vi "SpectrometerSpinCoater_v13.vi"() -> ()   [LabVIEW 2020]
uses:
  TypDef/TabControl_InSitu_Type.ctl
  <instrlib>/Classes/CCD/Abstract_CCD/Abstract_CCD.lvclass
  <instrlib>/Classes/SpinCoater/SpinCoater.lvclass
  TypDef/DeviceQueue_TypeDef.ctl
  TypDef/DeviceQueue_Action.ctl
  TypDef/TabControl.ctl
  TypDef/DataQueue_TypeDef.ctl
  TypDef/DataQueue_Action.ctl
  <vilib>/Utility/error.llb/DialogType.ctl
  <instrlib>/Classes/CCD/Avantes/Avantes.lvclass
  C:/Program Files/National Instruments/LabVIEW 2020/instr.lib/Classes/CCD/Abstract_CCD/Abstract_CCD.lvclass
  <vilib>/Analysis/baseanly.llb/A x Vector.vi
  <vilib>/Analysis/NI_AALBase.lvlib
panel:
  out "x-y":dbl
  in  "Reference\nValue":dbl=1.0
  out "WL-Det\nPos":i32
  in  "Motor_ShortStop":bool
  out "UpperWLLimit":i32=1065
  out "LowerWLLimit":i32=149
  out "Nr After Spin":u16
  out "Action":string="TimeOut"
  out "Time.spin":refnum<file>
  out "Meas.spin":refnum<file>
  out "Arduino":bool
  out "NKT":bool
  out "Spectromter":bool
  in  "Abort Button":bool
  in  "Stop Button":bool=TRUE
  in  "Tab Control":T1(tab)=enum."Settings"
  in  "Trim\nSpec":bool=TRUE
  in  "Wl \nUp":dbl[unit]=9.102385253906251e-07
  in  "Wl \nLow":dbl[unit]=3.7998095703125003e-07
  in  "Frames for Ref/Dark":dbl=10000.0
  in  "Shutter Toggle":bool
  in  "Program Spin Coater":T2(array[cluster])=[{"Speed (rpm)"=1430.0, "Time (s)"=45.0, "Acc (rpm/s)"=0.0}]
  in  "Spectra Count":u16
  in  "Measure_MeasureSpectrum":bool
  out "Overall Time":dbl=47.0
  in  "Frames":i32=123685
  in  "StartMeasurement_Button":bool
  in  "Measure_Preview":bool
  out "Measure_Graph":T3(graph) caption="XY Graph"
  in  "Measure_FramesSpectrometer":dbl=200.0 caption="Frames for Spectrometer"
  in  "StartSpin_Button":bool
  in  "Record RefSpec":bool
  in  "Measure:\nRecord_Darkspec":bool
  in  "Measure_Comments":string="Just for testing" caption="Comments"
  in  "Measure_FileName":string="Testing" caption="File Name"
  in  "Measure_SavePath":path=path "C:/Users/Cerberus/Desktop/Test/v12Test" caption="Save Path"
  out "Measure_FrameRate":dbl[unit]=2631.5791015625 caption="Frame Rate"
  in  "Measure_IntegrationTime":dbl[unit]=3e-05 caption="Integration Time"
  in  "Tab Control SpinType":T4
  in  "Seconds after Spin":dbl[unit]=1.0
  in  "Calculate Frames_Normal":bool=TRUE caption="Calculate Frames"
  in  "periodic time":dbl[unit]=2.0
  in  "Duration after":dbl[unit]
  in  "Spin at end":bool
  in  "Seconds to Spin_Normal":dbl[unit]=1.0 caption="Seconds to Spin"
  in  "Threshold":dbl=0.3
  in  "Time Detect":dbl[unit]=2.0
  in  "Seconds to Spin_Short":dbl[unit]=1.0 caption="Seconds to Spin"
  in  "Spin Time":dbl[unit]=2.0
  in  "Calculate Frames_Short":bool=TRUE caption="Calculate Frames"
  in  "Wavelenght Detect":dbl[unit]=6.000000000000001e-07
  out "SS_StepsLeft":dbl
  out "SS_TimePrediction":dbl[unit]=-6.0
  out "Horizontal Progress Bar":u8(slide) scale=0.0..100.0
  in  "SpectralStability:\nRecord_Darkspec":bool
  in  "SpectralStability_Record":bool
  in  "SpectralStability_\nMeasurementNumber":u32 caption="Measurement Number"
  in  "SpectralStability_Duration":dbl[unit] caption="Duration"
  in  "Duration/Times":bool
  in  "SpectralStability_\nPeriodicTime":dbl[unit] caption="Periodic Time"
  in  "SpectralStability_MeasureSpectrum":bool
  in  "SpectralStability_Preview":bool
  out "SpectralStability_Graph":T3(graph) caption="XY Graph"
  in  "SpectralStability_FramesSpectrometer":dbl=200.0 caption="Frames for Spectrometer"
  in  "SpectralStability_Comments":string="Just for testing" caption="Comments"
  in  "SpectralStability_FileName":string="TestingAfter" caption="File Name"
  in  "SpectralStability_SavePath":path=path "C:/Users/Timo/Desktop/Test/180824" caption="Save Path"
  out "SpectralStability_FrameRate":dbl[unit]=2631.5791015625 caption="Frame Rate"
  in  "SpectralStability_IntegrationTime":dbl[unit]=3e-05 caption="Integration Time"
  in  "Shutter Close":bool
  in  "Shutter Open":bool
  in  "SHUTTER DEBUG":bool
  in  "Shutter Position":u16=1000
  in  "Dividider Get Spectra":u32=1 min=1
  in  "Automatically \nadjust count":bool=TRUE
  in  "Reset Count\nafter Spin Coating":bool=TRUE
  in  "ESC_Speed":dbl
  in  "ESC_Milliseconds":dbl
  in  "ESC DEBUG":bool
  in  "Port Arduino":refnum<visa-resource-name>="COM7"
  out "Error Arduino":bool caption="Error"
  in  "Init_Arduino":bool caption="Init"
  out "Caption_Settings_Arduino":string="Arduino"
  out "Caption_Settings_NKT":string="NKT Laser"
  out "Error_Spectromter":bool caption="Error"
  in  "Init_Spectrometer":bool caption="Init"
  out "Caption_Settings_Spectrometer":string="Spectromter"
  # "Speed (rpm)   Time (s)        Acceleration \n                                               (rpm/s)"
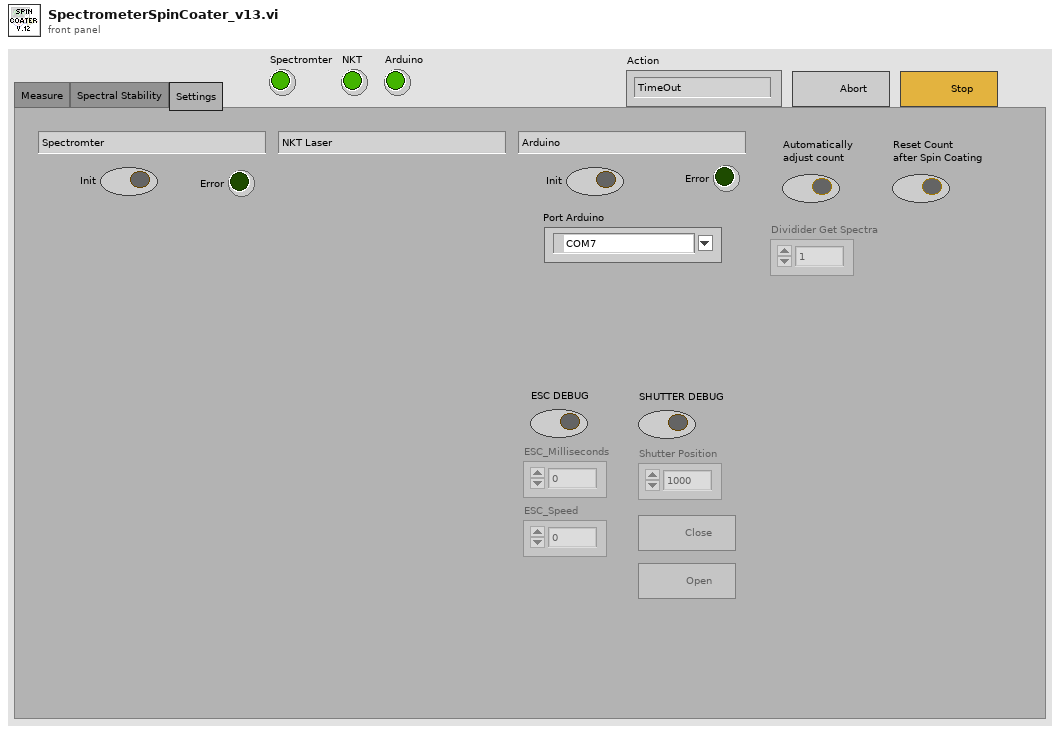
[diagram p1: front panel]
types:
  T1 = enum32{"Measure", "Spectral Stability", "Settings"}
  T2 = cluster{"Speed (rpm)":dbl, "Time (s)":dbl, "Acc (rpm/s)":dbl}[]
  T3 = cluster{"Wavlength":dbl[unit][], "Image":dbl[]}[]
  T4 = typedef "TabControl_InSitu_Type.ctl" = enum32{"Normal", "Short"}
  T5 = cluster{"Dark":cluster{"Image":dbl[][][], "Frame Size":cluster{"F":i32, "Y":i32, "X":i32}}[], "Ref":cluster{"Image":dbl[][][], "Frame Size":cluster{"F":i32, "Y":i32, "X":i32}}[], "Wavlength":dbl[unit][], "Wavlength Trim":dbl[unit][], "spec":dbl[][]}
  T6 = cluster{"Abstract_CCD.lvclass":refnum<class "Abstract_CCD.lvclass">, "SpinCoater.lvclass":refnum<class "SpinCoater.lvclass">}
  T7 = enum8{"Enabled", "Disabled", "Disabled and Grayed Out"}
  T8 = typedef "DataQueue_TypeDef.ctl" = cluster{"QueueAction":T9, "Data":cluster{"Image":dbl[][][], "Frame Size":cluster{"F":i32, "Y":i32, "X":i32}}[], "Data_Raw":cluster{"Image":dbl[][][], "Frame Size":cluster{"F":i32, "Y":i32, "X":i32}}[], "Data_Dark":cluster{"Image":dbl[][][], "Frame Size":cluster{"F":i32, "Y":i32, "X":i32}}[], "Data_Ref":cluster{"Image":dbl[][][], "Frame Size":cluster{"F":i32, "Y":i32, "X":i32}}[], "Device Information":string[], "Numeric Control":dbl, "Boolean":bool, "Wavelength":dbl[unit][], "Time":dbl[], "Time Stamp":timestamp, "Numeric Control 2":dbl, "TabControl":T10, "Numeric Control 3":dbl}
  T9 = typedef "DataQueue_Action.ctl" = enum16{"TimeOut", "Close_Program", "Abort", "Stop_Measurement", "Measure_InSituSpinCoating", "Measure_InSituSpinCoating_Short", "Measure_Spectrum", "Measure_SpectrumAdvanced", "Measure_SpectralStability", "Save_InSitu", "Save_SpectralStability", "Set_Ref", "Set_Dark", "Set_Wavelength", "Spectrometer_Measure", "Spectrometer_Preview", "Transfer_Settings", "Change_TrimSettings"}
  T10 = typedef "TabControl.ctl" = enum16{"Measure", "Spectral Stability", "Settings"}
  T11 = typedef "DeviceQueue_TypeDef.ctl" = cluster{"QueueAction":T12, "Numeric 1":dbl, "Numeric 2":dbl, "Boolean 1":bool, "Boolean 2":bool, "Spin Program":dbl[][], "Spin Prg v07":cluster{"Speed (rpm)":dbl, "Time (s)":dbl, "Acc (rpm/s)":dbl}[], "Time Stamp":timestamp, "TabControl":T10}
  T12 = typedef "DeviceQueue_Action.ctl" = enum16{"TimeOut", "Wait", "Close_Program", "Abort", "Spectrometer_Init", "Spectrometer_Close", "Spectrometer_DeviceInformation", "Spectrometer_Measure", "Spectrometer_MeasureAdvanced", "Spectrometer_Preview", "Spectrometer_Abort", "Spectrometer_StartMeasurement", "Spectrometer_GetData", "Spectrometer_GetData_Short", "Spectrometer_StopMeasurement", "Spectrometer_SetIntegrationTime", "Spectrometer_SetFrames", "Spectrometer_SetDarkspec", "Spectrometer_SetReference", "Spectrometer_SetTriggerMode", "Laser_Init", "Laser_Close", "Arduino_Init", "Arduino_Close", "Arduino_LoadProgram", "Arduino_StartProgram", "Arduino_SetSpeed", "Arduino_SetMillis", "Arduino_StopSpin", "Arduino_ShortStop", "Arduino_Shutter_SetPosition", "Arduino_Shutter_Close", "Arduino_Shutter_Open", "Measure_InSitu", "Measure_Spectrum", "Measure_InSituAdvanced", "Measure_InSituAdvanced_Short", "Measure_SpectralStability", "Measure_Stop"}
  T13 = enum16{"open", "replace", "create", "open or create", "replace or create", "replace or create with confirmation"}
  T14 = cluster{"Image":dbl[][][], "Frame Size":cluster{"F":i32, "Y":i32, "X":i32}}[]
  T15 = cluster{"Image":dbl[][][], "Frame Size":cluster{"F":i32, "Y":i32, "X":i32}}
  T16 = cluster{"Wavlength":dbl[unit][], "A x Vector":dbl[]}
  T17 = cluster{"Wavlength":dbl[unit][], "A x Vector":dbl[]}[]
  T18 = cluster{u16[][][], u16[][][], dbl[], "Numeric Control":dbl, "Numeric Control 2":dbl}
  T19 = typedef "DialogType.ctl" = u16
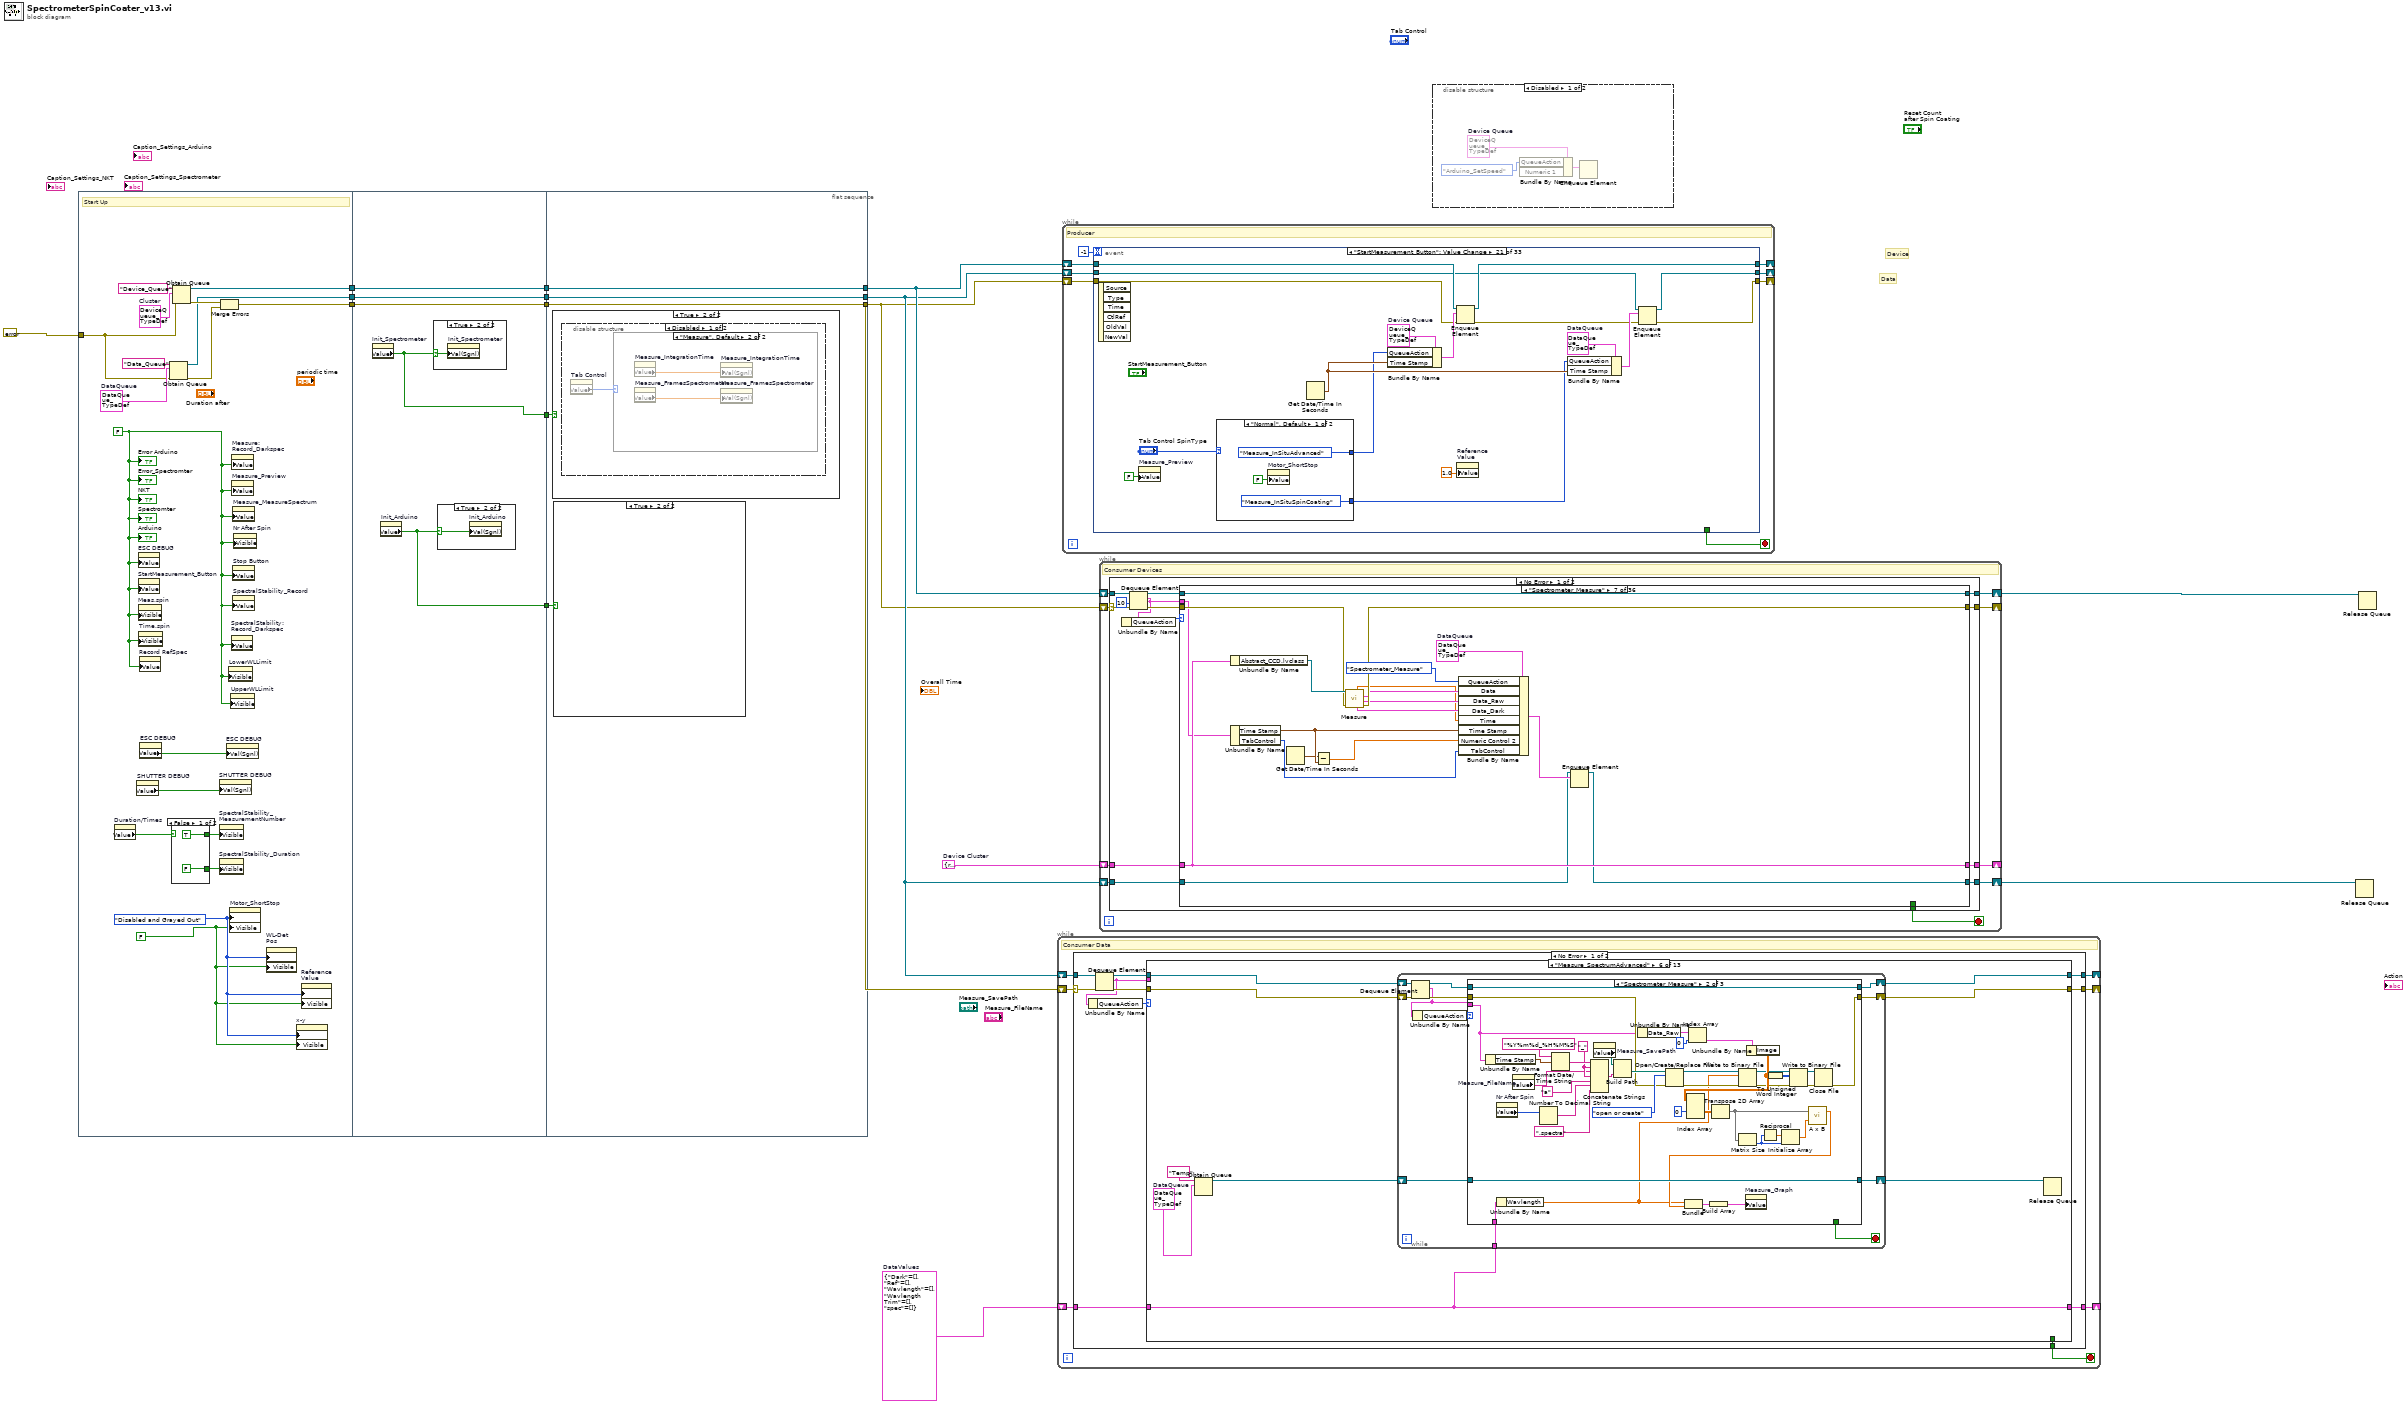
[diagram p0: block diagram]
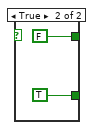
[diagram p3: hidden frame]
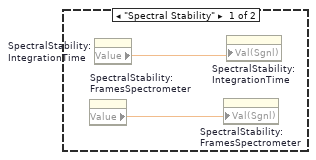
[diagram p8: hidden frame]
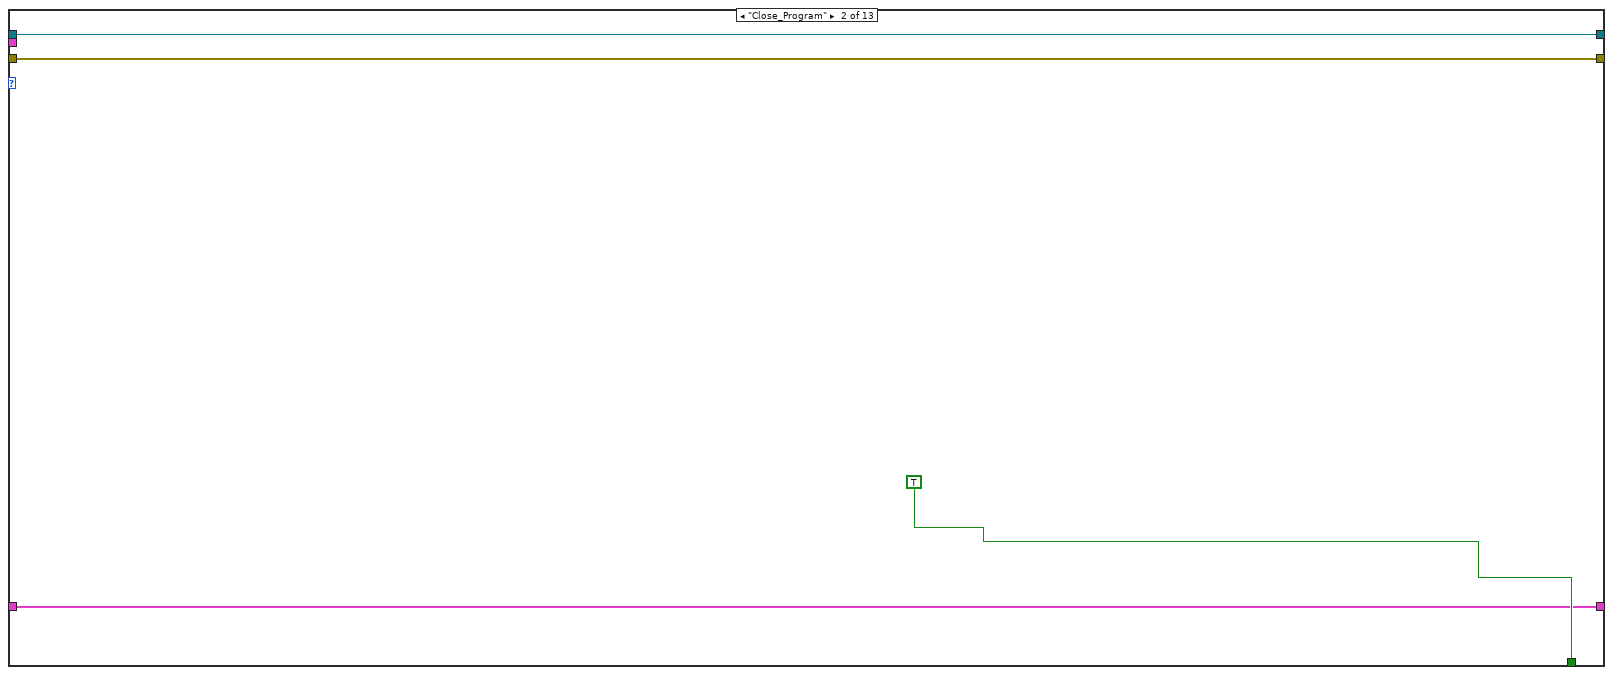
[diagram p11: hidden frame]
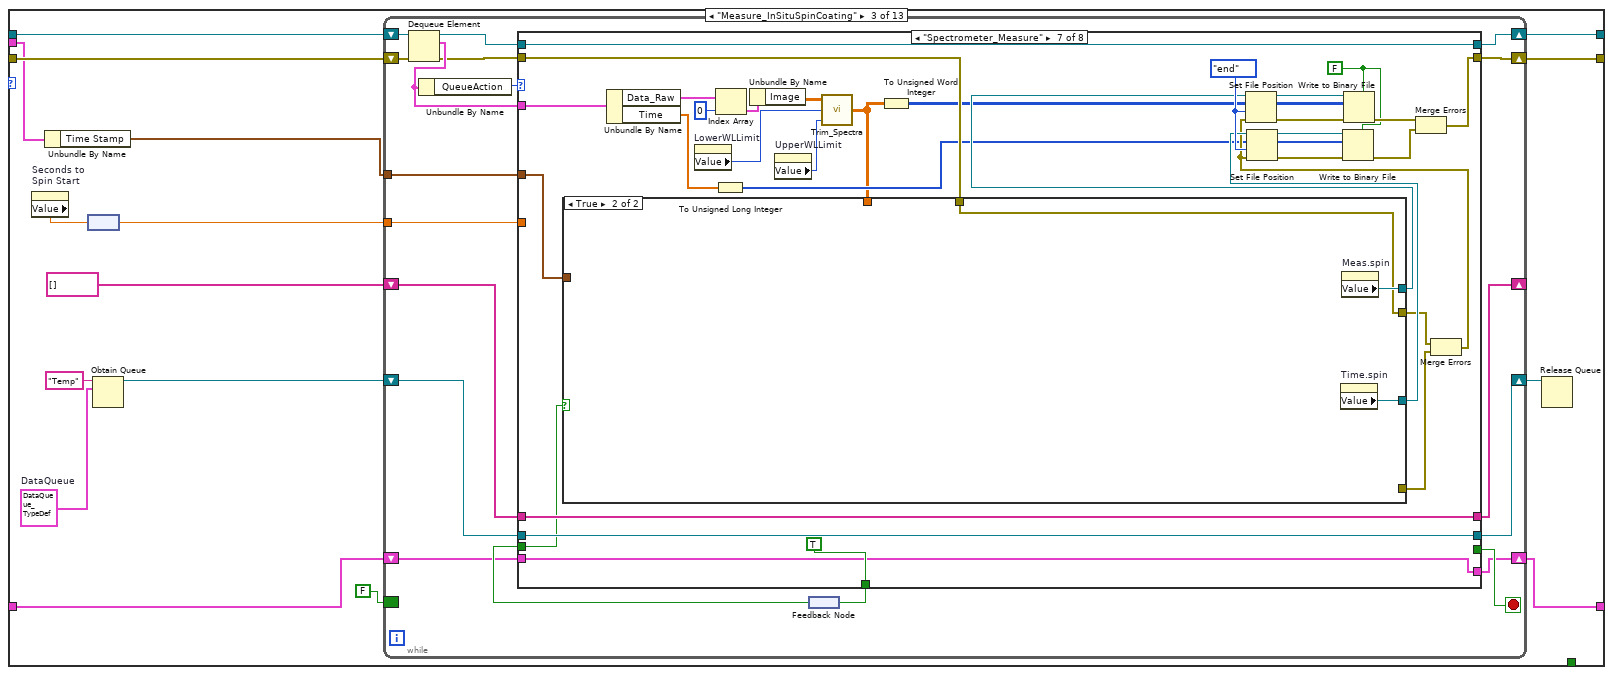
[diagram p12: hidden frame]
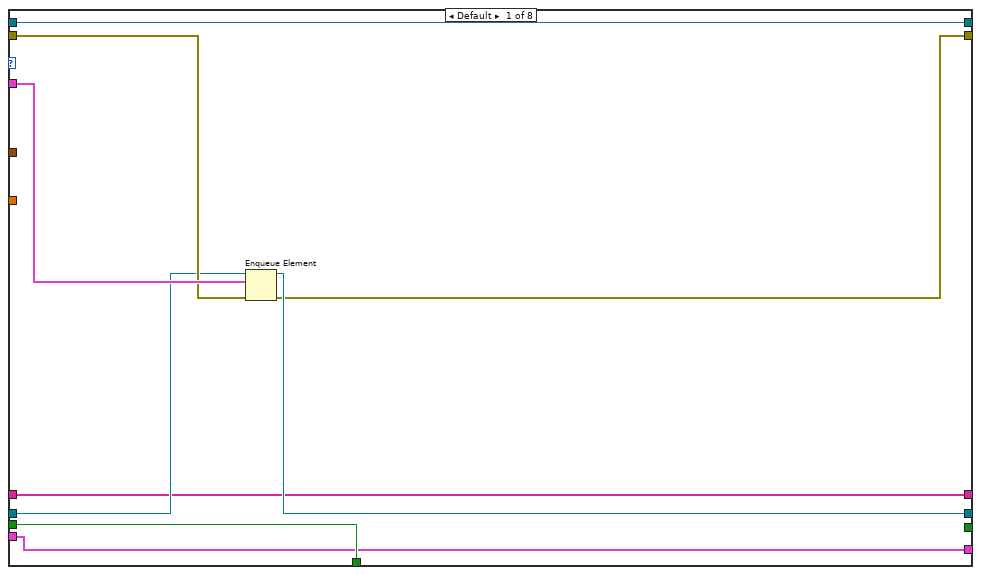
[diagram p13: hidden frame]
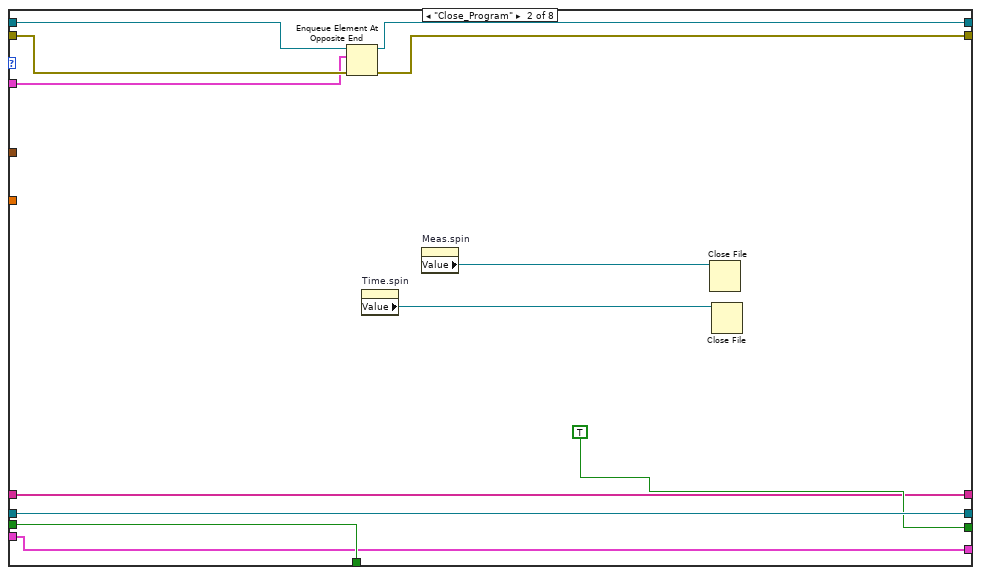
[diagram p14: hidden frame]
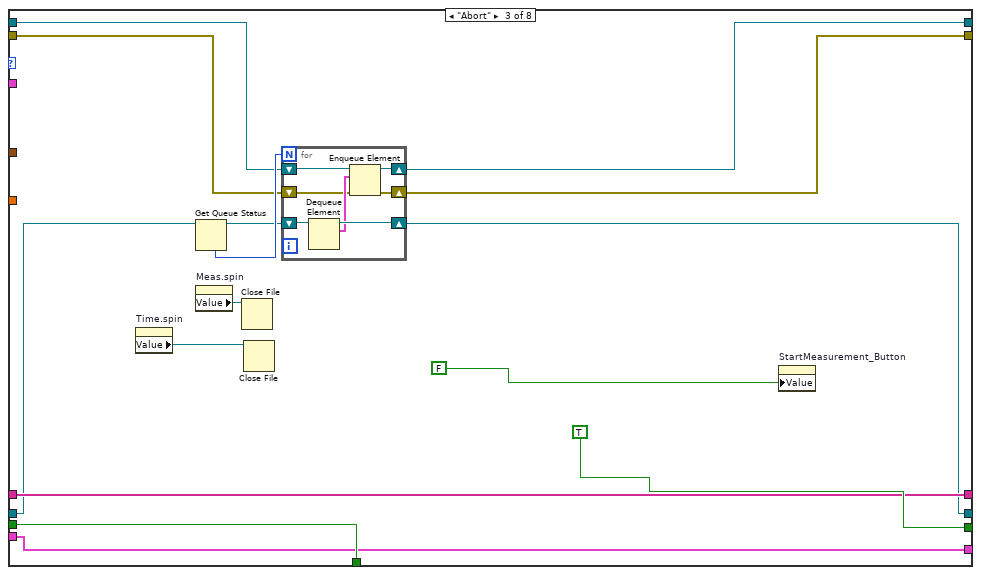
[diagram p15: hidden frame]
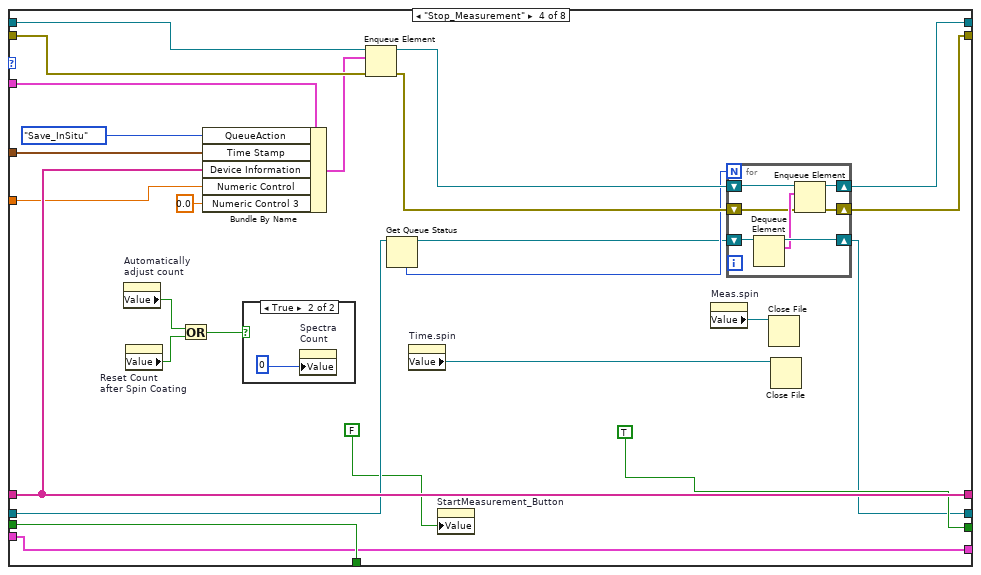
[diagram p16: hidden frame]
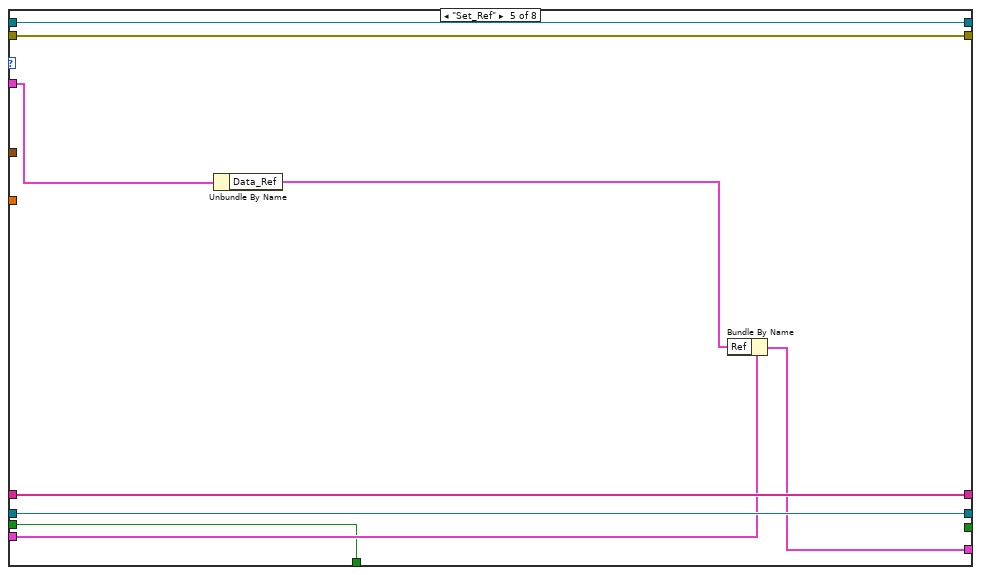
[diagram p18: hidden frame]
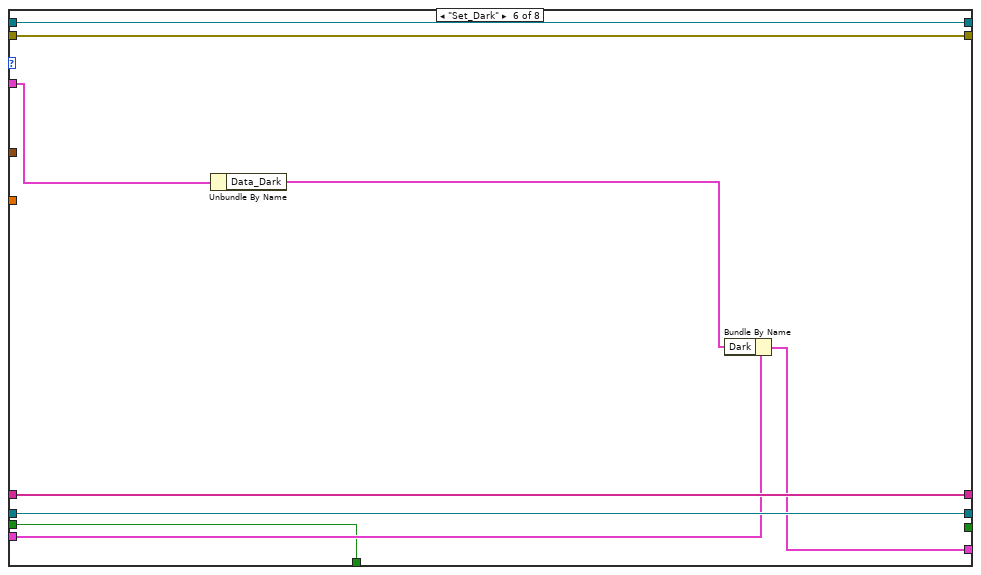
[diagram p19: hidden frame]
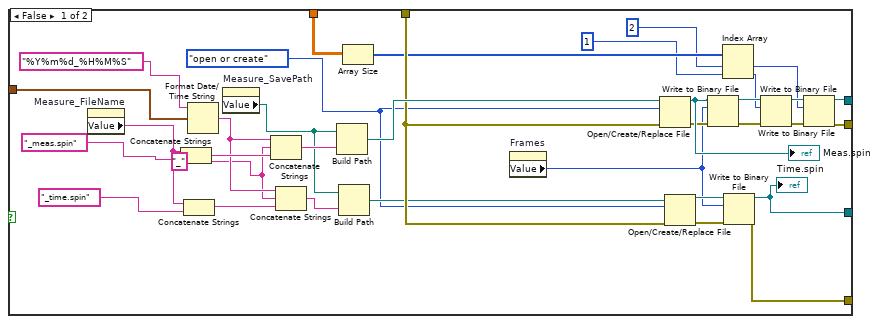
[diagram p20: hidden frame]
diagram:
  w7 = T5 {"Dark"=[], "Ref"=[], "Wavlength"=[], "Wavlength Trim"=[], "spec"=[]}  # DataValues
  w11 = T6 {"Abstract_CCD.lvclass"=refnum, "SpinCoater.lvclass"=refnum}  # Device Cluster
  # "Data"
  # "Device"
  n1 = flat-sequence {
    tunnel: errorcluster {"status"=FALSE, "code"=0, "source"=""} ("error constant") -> [w29]
    tunnel: [w32] -> w15
    tunnel: [w26] -> w14
    tunnel: [w25] -> w13
    tunnel: w15 -> [w43]
    tunnel: w14 -> [w42]
    tunnel: w13 -> [w41]
    tunnel: [w43] -> w6
    tunnel: [w42] -> w5
    tunnel: [w41] -> w4
    tunnel: [w40] -> w3
    tunnel: [w39] -> w2
    tunnel: [w48] -> w1
    tunnel: [w49] -> w8
    tunnel: [w50] -> w12
    tunnel: w6 -> [w50]
    tunnel: w5 -> [w49]
    tunnel: w4 -> [w48]
    tunnel: w3 -> [w47]
    tunnel: w2 -> [w46]
    frame #0 {
      w18 = T7."Disabled and Grayed Out" ("Disabled")
      w17 = FALSE ("Visible")
      w30 = T8 {"QueueAction"=enum."TimeOut", "Data"=[], "Data_Raw"=[], "Data_Dark"=[], "Data_Ref"=[], "Device Information"=[], "Numeric Control"=0.0, "Boolean"=FALSE, "Wavelength"=[], "Time"=[], "Time Stamp"=timestamp(0 s since 1904-01-01), "Numeric Control 2"=0.0, "TabControl"=enum."Measure", "Numeric Control 3"=0.0}  # DataQueue
      w33 = T11 {"QueueAction"=enum."TimeOut", "Numeric 1"=0.0, "Numeric 2"=0.0, "Boolean 1"=FALSE, "Boolean 2"=FALSE, "Spin Program"=[], "Spin Prg v07"=[], "Time Stamp"=timestamp(0 s since 1904-01-01), "TabControl"=enum."Measure"}  # Cluster
      w19 = FALSE ("Error Arduino")
      # "Start Up"
      n2 = property on="Duration/Times" class="Bool (strict)"() -> ("Value"=w21:bool)  [unwired: 2 in, 2 out]
      n3 = property on="SHUTTER DEBUG" class="Bool (strict)"() -> ("Value"=w20:bool)  [unwired: 2 in, 2 out]
      n4 = property on="ESC DEBUG" class="Bool (strict)"("Value"=w19) -> ()  [unwired: 2 in, 2 out]
      n5 = property on="StartMeasurement_Button" class="Bool (strict)"("Value"=w19) -> ()  [unwired: 2 in, 2 out]
      n6 = property on="Meas.spin" class="Ref (strict)"("Visible"=w19) -> ()  [unwired: 2 in, 2 out]
      n7 = property on="Time.spin" class="Ref (strict)"("Visible"=w19) -> ()  [unwired: 2 in, 2 out]
      n8 = property on="Record RefSpec" class="Bool (strict)"("Value"=w19) -> ()  [unwired: 2 in, 2 out]
      n9 = property on="ESC DEBUG" class="Bool (strict)"() -> ("Value"=w24:bool)  [unwired: 2 in, 2 out]
      n10 = Obtain Queue(name (unnamed)="Data_Queue", element data type=w30, error in (no error)=w29) -> (queue out=w26:refnum<queue>, error out=w27:errorcluster)  [unwired: 2 in, 1 out]
      n11 = case shown="False" w21 {
        tunnel: [FALSE TRUE] -> w23
        tunnel: [TRUE FALSE] -> w22
        frame False {
        }
        frame True {
        }
      }
      n12 = Obtain Queue(name (unnamed)="Device_Queue", element data type=w33, error in (no error)=w29) -> (queue out=w32:refnum<queue>, error out=w28:errorcluster)  [unwired: 2 in, 1 out]
      n13 = property on="SHUTTER DEBUG" class="Bool (strict)"("Val(Sgnl)"=w20) -> ()  [unwired: 2 in, 2 out]
      n14 = property on="SpectralStability_\nMeasurementNumber" class="DigNum (strict)"("Visible"=w22) -> ()  [unwired: 2 in, 2 out]
      n15 = property on="SpectralStability_Duration" class="DigNum (strict)"("Visible"=w23) -> ()  [unwired: 2 in, 2 out]
      n16 = Merge Errors(w28, w27) -> (w25:errorcluster)
      n17 = property on="ESC DEBUG" class="Bool (strict)"("Val(Sgnl)"=w24) -> ()  [unwired: 2 in, 2 out]
      n18 = property on="LowerWLLimit" class="DigNum (strict)"("Visible"=w19) -> ()  [unwired: 2 in, 2 out]
      n19 = property on="Motor_ShortStop" class="Bool (strict)"("DisabledEnum"=w18, "Visible"=w17) -> ()  [unwired: 2 in, 2 out]
      n20 = property on="UpperWLLimit" class="DigNum (strict)"("Visible"=w19) -> ()  [unwired: 2 in, 2 out]
      n21 = property on="SpectralStability:\nRecord_Darkspec" class="Bool (strict)"("Value"=w19) -> ()  [unwired: 2 in, 2 out]
      n22 = property on="Measure:\nRecord_Darkspec" class="Bool (strict)"("Value"=w19) -> ()  [unwired: 2 in, 2 out]
      n23 = property on="Measure_Preview" class="Bool (strict)"("Value"=w19) -> ()  [unwired: 2 in, 2 out]
      n24 = property on="Measure_MeasureSpectrum" class="Bool (strict)"("Value"=w19) -> ()  [unwired: 2 in, 2 out]
      n25 = property on="Stop Button" class="Bool (strict)"("Value"=w19) -> ()  [unwired: 2 in, 2 out]
      n26 = property on="SpectralStability_Record" class="Bool (strict)"("Value"=w19) -> ()  [unwired: 2 in, 2 out]
      n27 = property on="Nr After Spin" class="DigNum (strict)"("Visible"=w19) -> ()  [unwired: 2 in, 2 out]
      n28 = property on="WL-Det\nPos" class="DigNum (strict)"("DisabledEnum"=w18, "Visible"=w17) -> ()  [unwired: 2 in, 2 out]
      n29 = property on="x-y" class="DigNum (strict)"("DisabledEnum"=w18, "Visible"=w17) -> ()  [unwired: 2 in, 2 out]
      n30 = property on="Reference\nValue" class="DigNum (strict)"("DisabledEnum"=w18, "Visible"=w17) -> ()  [unwired: 2 in, 2 out]
      "Error_Spectromter" <- w19
      "Error Arduino" <- w19
      "Spectromter" <- w19
      "NKT" <- w19
      "Arduino" <- w19
    }
    frame #1 {
      n31 = property on="Init_Spectrometer" class="Bool (strict)"() -> ("Value"=w40:bool)  [unwired: 2 in, 2 out]
      n32 = property on="Init_Arduino" class="Bool (strict)"() -> ("Value"=w39:bool)  [unwired: 2 in, 2 out]
      n33 = case shown="True" w40 {
        selector: w40 -> [_ w45]
        frame False {
        }
        frame True {
          n34 = property on="Init_Spectrometer" class="Bool (strict)"("Val(Sgnl)"=w45) -> ()  [unwired: 2 in, 2 out]
        }
      }
      n35 = case shown="True" w39 {
        selector: w39 -> [_ w44]
        frame False {
        }
        frame True {
          n36 = property on="Init_Arduino" class="Bool (strict)"("Val(Sgnl)"=w44) -> ()  [unwired: 2 in, 2 out]
        }
      }
    }
    frame #2 {
      n37 = case shown="True" w47 {
        frame False {
        }
        frame True {
          n38 = disable-structure shown="Disabled" {
            frame Disabled {
              n39 = property on="Tab Control" class="TabCtl (strict)"() -> ("Value"=w51:T1)  [unwired: 2 in, 2 out]
              n40 = case shown="\"Measure\", Default" w51 {
                frame "Spectral Stability" {
                  n41 = property on="SpectralStability:\nFramesSpectrometer" class="DigNum (strict)"() -> ("Value"=w52:dbl)  [unwired: 2 in, 2 out]
                  n42 = property on="SpectralStability:\nIntegrationTime" class="DigNum (strict)"() -> ("Value"=w53:dbl[unit])  [unwired: 2 in, 2 out]
                  n43 = property on="SpectralStability:\nFramesSpectrometer" class="DigNum (strict)"("Val(Sgnl)"=w52) -> ()  [unwired: 2 in, 2 out]
                  n44 = property on="SpectralStability:\nIntegrationTime" class="DigNum (strict)"("Val(Sgnl)"=w53) -> ()  [unwired: 2 in, 2 out]
                }
                frame "Measure", Default {
                  n45 = property on="Measure_IntegrationTime" class="DigNum (strict)"() -> ("Value"=w54:dbl[unit])  [unwired: 2 in, 2 out]
                  n46 = property on="Measure_FramesSpectrometer" class="DigNum (strict)"() -> ("Value"=w55:dbl)  [unwired: 2 in, 2 out]
                  n47 = property on="Measure_IntegrationTime" class="DigNum (strict)"("Val(Sgnl)"=w54) -> ()  [unwired: 2 in, 2 out]
                  n48 = property on="Measure_FramesSpectrometer" class="DigNum (strict)"("Val(Sgnl)"=w55) -> ()  [unwired: 2 in, 2 out]
                }
              }
            }
            frame Enabled {
            }
          }
        }
      }
      n49 = case shown="True" w46 {
        frame False {
        }
        frame True {
        }
      }
    }
  }
  n50 = while {
    shift-right: [w56] -> _
    shift-left: w1 -> [w62]
    shift-right: [w57] -> _
    shift-left: w8 -> [w61]
    shift-right: [w58] -> _
    shift-left: w7 -> [w60]
    stop <- w59 stop-if-true
    # "Consumer Data"
    n51 = case shown="No Error" w62 {
      selector: w62 -> [w73 w1053]
      tunnel: w61 -> [w72 w1054]
      tunnel: w60 -> [w70 w1051]
      tunnel: [w69 _] -> w59
      tunnel: [w68 w1051] -> w58
      tunnel: [w67 w1054] -> w57
      tunnel: [w65 w1052] -> w56
      frame No Error {
        n52 = Dequeue Element(queue=w72, error in (no error)=w73) -> (queue out=w66:refnum<queue>, element=w63:T8, error out=w64:errorcluster)  [unwired: 1 in, 1 out]
        n53 = Unbundle By Name(w63) -> ("QueueAction"=w71:T9)
        n54 = case shown="\"Measure_SpectrumAdvanced\"" w71 {
          tunnel: w70 -> [w74 w79 w81 w294 w502 w609 w713 w932 w969 w978 w1001 w1014 w1021]
          tunnel: [_ TRUE _ _ _ _ _ _ _ _ _ _ _] -> w69
          tunnel: [w74 w79 w83 w296 w502 w609 w704 w932 w973 w992 w1000 w1014 w1020] -> w68
          tunnel: [w76 w78 w96 w309 w508 w615 w697 w954 w974 w993 w997 w1016 w1027] -> w67
          tunnel: w66 -> [w76 w78 w94 w307 w509 w616 w708 w954 w974 w993 w997 w1016 w1027]
          tunnel: [w75 w77 w95 w308 w507 w614 w698 w953 w975 w994 w998 w1015 w1024] -> w65
          tunnel: w64 -> [w75 w77 w93 w306 w510 w617 w707 w953 w975 w994 w998 w1015 w1024]
          tunnel: w63 -> [_ _ w88 w301 _ _ w700 w944 w976 w995 w999 w1005 w1026]
          frame "TimeOut", Default {
          }
          frame "Close_Program" {
          }
          frame "Measure_InSituSpinCoating" {
            w91 = T8 {"QueueAction"=enum."TimeOut", "Data"=[], "Data_Raw"=[], "Data_Dark"=[], "Data_Ref"=[], "Device Information"=[], "Numeric Control"=0.0, "Boolean"=FALSE, "Wavelength"=[], "Time"=[], "Time Stamp"=timestamp(0 s since 1904-01-01), "Numeric Control 2"=0.0, "TabControl"=enum."Measure", "Numeric Control 3"=0.0}  # DataQueue
            n55 = property on="Seconds to\nSpin Start" class="DigNum (strict)"() -> ("Value"=w85:dbl[unit])  [unwired: 2 in, 2 out]
            n56 = Unbundle By Name(w88) -> ("Time Stamp"=w87:timestamp)
            n57 = node(w85) -> (w84:dbl)
            n58 = Obtain Queue(name (unnamed)="Temp", element data type=w91) -> (queue out=w90:refnum<queue>)  [unwired: 3 in, 2 out]
            n59 = while {
              shift-right: [w106] -> w96
              shift-left: w94 -> [w115]
              shift-right: [w107] -> w95
              shift-left: w93 -> [w114]
              shift-right: [w108] -> w89
              shift-left: w90 -> [w109]
              tunnel: w87 -> [w102]
              shift-right: [w103] -> _
              shift-left: string[] [] ("Device Information") -> [w104]
              border: FALSE -> [_]
              tunnel: w84 -> [w99]
              shift-right: [w97] -> w83
              shift-left: w81 -> [w98]
              stop <- w105 stop-if-true
              n60 = Dequeue Element(queue=w115, error in (no error)=w114) -> (queue out=w110:refnum<queue>, element=w112:T8, error out=w111:errorcluster)  [unwired: 1 in, 1 out]
              n61 = Unbundle By Name(w112) -> ("QueueAction"=w113:T9)
              n62 = feedback #1() -> (w101:bool)
              n63 = case shown="\"Spectrometer_Measure\"" w113 {
                tunnel: w112 -> [w124 w134 _ w183 w201 w210 w242 w287]
                tunnel: w111 -> [w123 w135 w142 w180 w199 w208 w233 w284]
                tunnel: w110 -> [w119 w136 w141 w179 w200 w209 w241 w285]
                tunnel: w109 -> [w122 w131 w143 w174 w197 w206 w230 w288]
                tunnel: [w121 w131 w138 w171 w197 w206 w230 w288] -> w108
                tunnel: [w120 w132 w140 w170 w199 w208 w231 w284] -> w107
                tunnel: [w119 w133 w139 w169 w200 w209 w241 w285] -> w106
                tunnel: [_ TRUE TRUE TRUE _ _ _ _] -> w105
                tunnel: w104 -> [w118 w129 w150 w181 w198 w207 w228 _]
                tunnel: [w118 w129 w150 w181 w198 w207 w228 w286] -> w103
                tunnel: w102 -> [_ _ _ w182 _ _ w243 _]
                tunnel: w101 -> [w117 w128 w149 w168 w193 w202 w226 w283]
                tunnel: [w117 w128 w149 w168 w193 w202 TRUE w283] -> w100
                tunnel: w99 -> [_ _ _ w165 _ _ _ _]
                tunnel: w98 -> [w116 w125 w137 w160 w196 w205 w211 w282]
                tunnel: [w116 w125 w137 w160 w194 w203 w211 w282] -> w97
                frame Default {
                  n64 = Enqueue Element(queue=w122, element=w124, error in (no error)=w123) -> (queue out=w121:refnum<queue>, error out=w120:errorcluster)  [unwired: 1 in, 1 out]
                }
                frame "Close_Program" {
                  n65 = Enqueue Element At Opposite End(queue=w136, element=w134, error in (no error)=w135) -> (queue out=w133:refnum<queue>, error out=w132:errorcluster)  [unwired: 1 in, 1 out]
                  n66 = property on="Time.spin" class="Ref (strict)"() -> ("Value"=w126:refnum<file>)  [unwired: 2 in, 2 out]
                  n67 = property on="Meas.spin" class="Ref (strict)"() -> ("Value"=w127:refnum<file>)  [unwired: 2 in, 2 out]
                  n68 = Close File(refnum=w127) -> ()  [unwired: 1 in, 2 out]
                  n69 = Close File(refnum=w126) -> ()  [unwired: 1 in, 2 out]
                }
                frame "Abort" {
                  n70 = property on="Time.spin" class="Ref (strict)"() -> ("Value"=w147:refnum<file>)  [unwired: 2 in, 2 out]
                  n71 = Get Queue Status(queue=w143) -> (queue out=w144:refnum<queue>, # elements in queue=w145:i32)  [unwired: 2 in, 6 out]
                  n72 = property on="Meas.spin" class="Ref (strict)"() -> ("Value"=w148:refnum<file>)  [unwired: 2 in, 2 out]
                  n73 = Close File(refnum=w148) -> ()  [unwired: 1 in, 2 out]
                  n74 = Close File(refnum=w147) -> ()  [unwired: 1 in, 2 out]
                  n75 = for {
                    N: w145 -> [_]
                    shift-right: [w157] -> w138
                    shift-left: w144 -> [w158]
                    shift-right: [w154] -> w139
                    shift-left: w141 -> [w155]
                    shift-right: [w152] -> w140
                    shift-left: w142 -> [w153]
                    n76 = Dequeue Element(queue=w158) -> (queue out=w157:refnum<queue>, element=w156:T8)  [unwired: 2 in, 2 out]
                    n77 = Enqueue Element(queue=w155, element=w156, error in (no error)=w153) -> (queue out=w154:refnum<queue>, error out=w152:errorcluster)  [unwired: 1 in, 1 out]
                  }
                  n78 = property on="StartMeasurement_Button" class="Bool (strict)"("Value"=FALSE ("StartMeasurement_Button")) -> ()  [unwired: 2 in, 2 out]
                }
                frame "Stop_Measurement" {
                  n79 = property on="Automatically \nadjust count" class="Bool (strict)"() -> ("Value"=w162:bool)  [unwired: 2 in, 2 out]
                  n80 = property on="Reset Count\nafter Spin Coating" class="Bool (strict)"() -> ("Value"=w163:bool)  [unwired: 2 in, 2 out]
                  n81 = Or(x=w162, y=w163) -> (x .or. y?=w161:bool)
                  n82 = Bundle By Name(cluster=w183, "QueueAction"=DataQueue_Action."Save_InSitu", "Time Stamp"=w182, "Device Information"=w181, "Numeric Control"=w165, "Numeric Control 3"=0.0) -> (w178:T8)
                  n83 = case shown="True" w161 {
                    frame False {
                    }
                    frame True {
                      n84 = property on="Spectra \nCount" class="DigNum (strict)"("Value"=u16 0 ("Spectra Count")) -> ()  [unwired: 2 in, 2 out]
                    }
                  }
                  n85 = Enqueue Element(queue=w179, element=w178, error in (no error)=w180) -> (queue out=w176:refnum<queue>, error out=w175:errorcluster)  [unwired: 1 in, 1 out]
                  n86 = Get Queue Status(queue=w174) -> (queue out=w172:refnum<queue>, # elements in queue=w173:i32)  [unwired: 2 in, 6 out]
                  n87 = property on="Time.spin" class="Ref (strict)"() -> ("Value"=w166:refnum<file>)  [unwired: 2 in, 2 out]
                  n88 = property on="StartMeasurement_Button" class="Bool (strict)"("Value"=FALSE ("StartMeasurement_Button")) -> ()  [unwired: 2 in, 2 out]
                  n89 = property on="Meas.spin" class="Ref (strict)"() -> ("Value"=w167:refnum<file>)  [unwired: 2 in, 2 out]
                  n90 = for {
                    N: w173 -> [_]
                    shift-right: [w191] -> w171
                    shift-left: w172 -> [w192]
                    shift-right: [w188] -> w169
                    shift-left: w176 -> [w189]
                    shift-right: [w186] -> w170
                    shift-left: w175 -> [w187]
                    n91 = Dequeue Element(queue=w192) -> (queue out=w191:refnum<queue>, element=w190:T8)  [unwired: 2 in, 2 out]
                    n92 = Enqueue Element(queue=w189, element=w190, error in (no error)=w187) -> (queue out=w188:refnum<queue>, error out=w186:errorcluster)  [unwired: 1 in, 1 out]
                  }
                  n93 = Close File(refnum=w167) -> ()  [unwired: 1 in, 2 out]
                  n94 = Close File(refnum=w166) -> ()  [unwired: 1 in, 2 out]
                }
                frame "Set_Ref" {
                  n95 = Unbundle By Name(w201) -> ("Data_Ref"=w195:T14)
                  n96 = Bundle By Name(cluster=w196, "Ref"=w195) -> (w194:T5)
                }
                frame "Set_Dark" {
                  n97 = Unbundle By Name(w210) -> ("Data_Dark"=w204:T14)
                  n98 = Bundle By Name(cluster=w205, "Dark"=w204) -> (w203:T5)
                }
                frame "Spectrometer_Measure" {
                  w216 = FALSE ("prepend array or string size? (T)")
                  w229 = enum16{"start", "end", "current"}."end" ("from (0:start)")
                  n99 = Unbundle By Name(w242) -> ("Data_Raw"=w238:T14, "Time"=w232:dbl[])
                  n100 = property on="LowerWLLimit" class="DigNum (strict)"() -> ("Value"=w213:i32)  [unwired: 2 in, 2 out]
                  n101 = To Unsigned Long Integer(number=w232) -> (unsigned 32bit integer=w218:u32[])
                  n102 = Index Array(array=w238, index=0) -> (element=w237:T15)
                  n103 = Unbundle By Name(w237) -> ("Image"=w215:dbl[][][])
                  n104 = property on="UpperWLLimit" class="DigNum (strict)"() -> ("Value"=w212:i32)  [unwired: 2 in, 2 out]
                  n105 = call "Trim_Spectra.vi"("WL_UpperIndex"=w212, "WL_LowerIndex"=w213, "Image"=w215) -> ("ImageCut"=w214:dbl[][][])
                  n106 = case shown="True" w226 {
                    tunnel: w243 -> [w275 _]
                    tunnel: w233 -> [w270 w279]
                    tunnel: [w256 w279] -> w220
                    tunnel: [w244 _] -> w221
                    tunnel: [w255 w281] -> w223
                    tunnel: [w245 w280] -> w222
                    tunnel: w214 -> [w253 _]
                    frame False {
                      w265 = T13."open or create" ("operation (0:open)")
                      w264 = "_" ("string")
                      n107 = property on="Measure_FileName" class="Str"() -> ("Value"=w273:string)  [unwired: 2 in, 2 out]
                      n108 = Concatenate Strings(w273, "_meas.spin" ("string")) -> (w276:string)
                      n109 = Concatenate Strings(w273, "_time.spin" ("string")) -> (w268:string)
                      n110 = Format Date/Time String(time format string (%c)="%Y%m%d_%H%M%S", seconds (now)=w275) -> (date/time string=w269:string)  [unwired: 1 in]
                      n111 = property on="Measure_SavePath" class="Path"() -> ("Value"=w247:path)  [unwired: 2 in, 2 out]
                      n112 = Concatenate Strings(w269, w264, w276) -> (w274:string)
                      n113 = Concatenate Strings(w269, w264, w268) -> (w267:string)
                      n114 = Build Path(base path=w247, name or relative path=w274) -> (appended path=w271:path)
                      n115 = Build Path(base path=w247, name or relative path=w267) -> (appended path=w266:path)
                      n116 = Array Size(array=w253) -> (size(s)=w252:i32[])
                      n117 = property on="Frames" class="DigNum (strict)"() -> ("Value"=w246:i32)  [unwired: 2 in, 2 out]
                      n118 = Open/Create/Replace File(file path (use dialog)=w271, error in=w270, operation (0:open)=w265) -> (refnum out=w263:refnum<file>, error out=w262:errorcluster)  [unwired: 3 in, 1 out]
                      "Meas.spin" <- w263
                      n119 = Open/Create/Replace File(file path (use dialog)=w266, error in=w270, operation (0:open)=w265) -> (refnum out=w261:refnum<file>, error out=w260:errorcluster)  [unwired: 3 in, 1 out]
                      n120 = Write to Binary File(file (use dialog)=w263, data=w246, error in=w262) -> (refnum out=w259:refnum<file>, error out=w258:errorcluster)  [unwired: 3 in, 1 out]
                      n121 = Index Array(array=w252, index #1=2 ("index"), index #2=1 ("index")) -> (element #1=w248:i32, element #2=w249:i32)
                      n122 = Write to Binary File(file (use dialog)=w261, data=w246, error in=w260) -> (refnum out=w245:refnum<file>, error out=w244:errorcluster)  [unwired: 3 in, 1 out]
                      "Time.spin" <- w245
                      n123 = Write to Binary File(file (use dialog)=w259, data=w249, error in=w258) -> (refnum out=w254:refnum<file>, error out=w257:errorcluster)  [unwired: 3 in, 1 out]
                      n124 = Write to Binary File(file (use dialog)=w254, data=w248, error in=w257) -> (refnum out=w255:refnum<file>, error out=w256:errorcluster)  [unwired: 3 in, 1 out]
                    }
                    frame True {
                      n125 = property on="Time.spin" class="Ref (strict)"() -> ("Value"=w280:refnum<file>)  [unwired: 2 in, 2 out]
                      n126 = property on="Meas.spin" class="Ref (strict)"() -> ("Value"=w281:refnum<file>)  [unwired: 2 in, 2 out]
                    }
                  }
                  n127 = To Unsigned Word Integer(number=w214) -> (unsigned 16bit integer=w217:u16[][][])
                  n128 = Merge Errors(w220, w221) -> (w219:errorcluster)
                  n129 = Set File Position(refnum=w223, from (0:start)=w229, error in=w219) -> (refnum out=w235:refnum<file>, error out=w234:errorcluster)  [unwired: 1 in]
                  n130 = Set File Position(refnum=w222, from (0:start)=w229, error in=w219) -> (refnum out=w240:refnum<file>, error out=w239:errorcluster)  [unwired: 1 in]
                  n131 = Write to Binary File(file (use dialog)=w240, data=w218, error in=w239, 5:w216) -> (error out=w224:errorcluster)  [unwired: 2 in, 2 out]
                  n132 = Write to Binary File(file (use dialog)=w235, data=w217, error in=w234, 5:w216) -> (error out=w225:errorcluster)  [unwired: 2 in, 2 out]
                  n133 = Merge Errors(w225, w224) -> (w231:errorcluster)
                }
                frame "Transfer_Settings" {
                  n134 = Unbundle By Name(w287) -> ("Device Information"=w286:string[])
                }
              }
              n135 = feedback-in #1(w100) -> ()
            }
            n136 = Release Queue(queue=w89) -> ()  [unwired: 2 in, 3 out]
          }
          frame "Measure_InSituSpinCoating_Short" {
            w304 = T8 {"QueueAction"=enum."TimeOut", "Data"=[], "Data_Raw"=[], "Data_Dark"=[], "Data_Ref"=[], "Device Information"=[], "Numeric Control"=0.0, "Boolean"=FALSE, "Wavelength"=[], "Time"=[], "Time Stamp"=timestamp(0 s since 1904-01-01), "Numeric Control 2"=0.0, "TabControl"=enum."Measure", "Numeric Control 3"=0.0}  # DataQueue
            n137 = property on="Seconds to\nSpin Start" class="DigNum (strict)"() -> ("Value"=w298:dbl[unit])  [unwired: 2 in, 2 out]
            n138 = Unbundle By Name(w301) -> ("Time Stamp"=w300:timestamp)
            n139 = node(w298) -> (w297:dbl)
            n140 = Obtain Queue(name (unnamed)="Temp", element data type=w304) -> (queue out=w303:refnum<queue>)  [unwired: 3 in, 2 out]
            n141 = Unbundle By Name(w294) -> ("Wavlength"=w292:dbl[unit][])
            n142 = Subtract(x=w292, y="Wavelenght Detect") -> (x-y=w293:dbl[unit][])
            n143 = Absolute Value(x=w293) -> (abs(x)=w291:dbl[unit][])
            n144 = Array Max & Min(array=w291) -> (min index (indices)=→"WL-Det\nPos":i32)  [unwired: 3 out]
            n145 = while {
              shift-right: [w319] -> w309
              shift-left: w307 -> [w328]
              shift-right: [w320] -> w308
              shift-left: w306 -> [w327]
              shift-right: [w321] -> w302
              shift-left: w303 -> [w322]
              tunnel: w300 -> [w315]
              shift-right: [w316] -> _
              shift-left: string[] [] ("Device Information") -> [w317]
              border: FALSE -> [_]
              tunnel: w297 -> [w312]
              shift-right: [w310] -> w296
              shift-left: w294 -> [w311]
              stop <- w318 stop-if-true
              n146 = Dequeue Element(queue=w328, error in (no error)=w327) -> (queue out=w323:refnum<queue>, element=w325:T8, error out=w324:errorcluster)  [unwired: 1 in, 1 out]
              n147 = Unbundle By Name(w325) -> ("QueueAction"=w326:T9)
              n148 = feedback #2() -> (w314:bool)
              n149 = case shown="\"Stop_Measurement\"" w326 {
                tunnel: w325 -> [w337 w347 _ w396 w414 w423 w455 w500]
                tunnel: w324 -> [w336 w348 w357 w393 w412 w421 w446 w497]
                tunnel: w323 -> [w332 w349 w356 w392 w413 w422 w454 w498]
                tunnel: w322 -> [w335 w344 w358 w387 w410 w419 w443 w501]
                tunnel: [w334 w344 w353 w384 w410 w419 w443 w501] -> w321
                tunnel: [w333 w345 w355 w383 w412 w421 w444 w497] -> w320
                tunnel: [w332 w346 w354 w382 w413 w422 w454 w498] -> w319
                tunnel: [_ TRUE TRUE TRUE _ _ _ _] -> w318
                tunnel: w317 -> [w331 w342 w363 w394 w411 w420 w441 _]
                tunnel: [w331 w342 w363 w394 w411 w420 w441 w499] -> w316
                tunnel: w315 -> [_ _ _ w395 _ _ w456 _]
                tunnel: w314 -> [w330 w341 w362 w381 w406 w415 w439 w496]
                tunnel: [w330 w341 w362 w381 w406 w415 TRUE w496] -> w313
                tunnel: w312 -> [_ _ _ w380 _ _ _ _]
                tunnel: w311 -> [w329 w340 w352 w375 w409 w418 w424 w495]
                tunnel: [w329 w340 w352 w375 w407 w416 w424 w495] -> w310
                frame Default {
                  n150 = Enqueue Element(queue=w335, element=w337, error in (no error)=w336) -> (queue out=w334:refnum<queue>, error out=w333:errorcluster)  [unwired: 1 in, 1 out]
                }
                frame "Close_Program" {
                  n151 = property on="Meas.spin" class="Ref (strict)"() -> ("Value"=w339:refnum<file>)  [unwired: 2 in, 2 out]
                  n152 = property on="Time.spin" class="Ref (strict)"() -> ("Value"=w338:refnum<file>)  [unwired: 2 in, 2 out]
                  n153 = Enqueue Element At Opposite End(queue=w349, element=w347, error in (no error)=w348) -> (queue out=w346:refnum<queue>, error out=w345:errorcluster)  [unwired: 1 in, 1 out]
                  n154 = Close File(refnum=w339) -> ()  [unwired: 1 in, 2 out]
                  n155 = Close File(refnum=w338) -> ()  [unwired: 1 in, 2 out]
                }
                frame "Abort" {
                  n156 = property on="Time.spin" class="Ref (strict)"() -> ("Value"=w350:refnum<file>)  [unwired: 2 in, 2 out]
                  n157 = property on="Meas.spin" class="Ref (strict)"() -> ("Value"=w351:refnum<file>)  [unwired: 2 in, 2 out]
                  n158 = Get Queue Status(queue=w358) -> (queue out=w359:refnum<queue>, # elements in queue=w360:i32)  [unwired: 2 in, 6 out]
                  n159 = Close File(refnum=w351) -> ()  [unwired: 1 in, 2 out]
                  n160 = Close File(refnum=w350) -> ()  [unwired: 1 in, 2 out]
                  n161 = for {
                    N: w360 -> [_]
                    shift-right: [w370] -> w353
                    shift-left: w359 -> [w371]
                    shift-right: [w367] -> w354
                    shift-left: w356 -> [w368]
                    shift-right: [w365] -> w355
                    shift-left: w357 -> [w366]
                    n162 = Dequeue Element(queue=w371) -> (queue out=w370:refnum<queue>, element=w369:T8)  [unwired: 2 in, 2 out]
                    n163 = Enqueue Element(queue=w368, element=w369, error in (no error)=w366) -> (queue out=w367:refnum<queue>, error out=w365:errorcluster)  [unwired: 1 in, 1 out]
                  }
                  n164 = property on="StartMeasurement_Button" class="Bool (strict)"("Value"=FALSE ("StartMeasurement_Button")) -> ()  [unwired: 2 in, 2 out]
                }
                frame "Stop_Measurement" {
                  n165 = property on="Automatically \nadjust count" class="Bool (strict)"() -> ("Value"=w377:bool)  [unwired: 2 in, 2 out]
                  n166 = property on="Reset Count\nafter Spin Coating" class="Bool (strict)"() -> ("Value"=w378:bool)  [unwired: 2 in, 2 out]
                  n167 = Or(x=w377, y=w378) -> (x .or. y?=w376:bool)
                  n168 = Bundle By Name(cluster=w396, "QueueAction"=DataQueue_Action."Save_InSitu", "Time Stamp"=w395, "Device Information"=w394, "Numeric Control"=w380, "Numeric Control 3"=1.0) -> (w391:T8)
                  n169 = case shown="True" w376 {
                    frame False {
                    }
                    frame True {
                      n170 = property on="Spectra \nCount" class="DigNum (strict)"("Value"=u16 0 ("Spectra Count")) -> ()  [unwired: 2 in, 2 out]
                    }
                  }
                  n171 = Enqueue Element(queue=w392, element=w391, error in (no error)=w393) -> (queue out=w389:refnum<queue>, error out=w388:errorcluster)  [unwired: 1 in, 1 out]
                  n172 = Get Queue Status(queue=w387) -> (queue out=w385:refnum<queue>, # elements in queue=w386:i32)  [unwired: 2 in, 6 out]
                  n173 = property on="StartMeasurement_Button" class="Bool (strict)"("Value"=FALSE ("StartMeasurement_Button")) -> ()  [unwired: 2 in, 2 out]
                  n174 = property on="Time.spin" class="Ref (strict)"() -> ("Value"=w373:refnum<file>)  [unwired: 2 in, 2 out]
                  n175 = property on="Meas.spin" class="Ref (strict)"() -> ("Value"=w374:refnum<file>)  [unwired: 2 in, 2 out]
                  n176 = for {
                    N: w386 -> [_]
                    shift-right: [w404] -> w384
                    shift-left: w385 -> [w405]
                    shift-right: [w401] -> w382
                    shift-left: w389 -> [w402]
                    shift-right: [w399] -> w383
                    shift-left: w388 -> [w400]
                    n177 = Dequeue Element(queue=w405) -> (queue out=w404:refnum<queue>, element=w403:T8)  [unwired: 2 in, 2 out]
                    n178 = Enqueue Element(queue=w402, element=w403, error in (no error)=w400) -> (queue out=w401:refnum<queue>, error out=w399:errorcluster)  [unwired: 1 in, 1 out]
                  }
                  n179 = Close File(refnum=w374) -> ()  [unwired: 1 in, 2 out]
                  n180 = Close File(refnum=w373) -> ()  [unwired: 1 in, 2 out]
                }
                frame "Set_Ref" {
                  n181 = Unbundle By Name(w414) -> ("Data_Ref"=w408:T14)
                  n182 = Bundle By Name(cluster=w409, "Ref"=w408) -> (w407:T5)
                }
                frame "Set_Dark" {
                  n183 = Unbundle By Name(w423) -> ("Data_Dark"=w417:T14)
                  n184 = Bundle By Name(cluster=w418, "Dark"=w417) -> (w416:T5)
                }
                frame "Spectrometer_Measure" {
                  w429 = FALSE ("prepend array or string size? (T)")
                  w442 = enum16{"start", "end", "current"}."end" ("from (0:start)")
                  n185 = Unbundle By Name(w455) -> ("Data_Raw"=w451:T14, "Time"=w445:dbl[])
                  n186 = property on="LowerWLLimit" class="DigNum (strict)"() -> ("Value"=w426:i32)  [unwired: 2 in, 2 out]
                  n187 = To Unsigned Long Integer(number=w445) -> (unsigned 32bit integer=w431:u32[])
                  n188 = Index Array(array=w451, index=0) -> (element=w450:T15)
                  n189 = Unbundle By Name(w450) -> ("Image"=w428:dbl[][][])
                  n190 = property on="UpperWLLimit" class="DigNum (strict)"() -> ("Value"=w425:i32)  [unwired: 2 in, 2 out]
                  n191 = call "Trim_Spectra.vi"("WL_UpperIndex"=w425, "WL_LowerIndex"=w426, "Image"=w428) -> ("ImageCut"=w427:dbl[][][])
                  n192 = case shown="False" w439 {
                    tunnel: w456 -> [w488 _]
                    tunnel: w446 -> [w483 w494]
                    tunnel: [w470 w494] -> w433
                    tunnel: [w459 _] -> w434
                    tunnel: [w469 w493] -> w436
                    tunnel: [w458 w492] -> w435
                    tunnel: w427 -> [w467 _]
                    frame False {
                      w478 = T13."open or create" ("operation (0:open)")
                      w477 = "_" ("string")
                      n193 = property on="Measure_FileName" class="Str"() -> ("Value"=w486:string)  [unwired: 2 in, 2 out]
                      n194 = Concatenate Strings(w486, "_meas.spin" ("string")) -> (w489:string)
                      n195 = Concatenate Strings(w486, "_time.spin" ("string")) -> (w481:string)
                      n196 = Format Date/Time String(time format string (%c)="%Y%m%d_%H%M%S", seconds (now)=w488) -> (date/time string=w482:string)  [unwired: 1 in]
                      n197 = property on="Measure_SavePath" class="Path"() -> ("Value"=w461:path)  [unwired: 2 in, 2 out]
                      n198 = Concatenate Strings(w482, w477, w489) -> (w487:string)
                      n199 = Concatenate Strings(w482, w477, w481) -> (w480:string)
                      n200 = Build Path(base path=w461, name or relative path=w487) -> (appended path=w484:path)
                      n201 = Build Path(base path=w461, name or relative path=w480) -> (appended path=w479:path)
                      n202 = Array Size(array=w467) -> (size(s)=w466:i32[])
                      n203 = property on="Frames" class="DigNum (strict)"() -> ("Value"=w460:i32)  [unwired: 2 in, 2 out]
                      n204 = Open/Create/Replace File(file path (use dialog)=w484, error in=w483, operation (0:open)=w478) -> (refnum out=w457:refnum<file>, error out=w476:errorcluster)  [unwired: 3 in, 1 out]
                      n205 = Open/Create/Replace File(file path (use dialog)=w479, error in=w483, operation (0:open)=w478) -> (refnum out=w475:refnum<file>, error out=w474:errorcluster)  [unwired: 3 in, 1 out]
                      n206 = Write to Binary File(file (use dialog)=w457, data=w460, error in=w476) -> (refnum out=w473:refnum<file>, error out=w472:errorcluster)  [unwired: 3 in, 1 out]
                      n207 = Index Array(array=w466, index #1=2 ("index"), index #2=1 ("index")) -> (element #1=w462:i32, element #2=w463:i32)
                      n208 = Write to Binary File(file (use dialog)=w475, data=w460, error in=w474) -> (refnum out=w458:refnum<file>, error out=w459:errorcluster)  [unwired: 3 in, 1 out]
                      n209 = property on="Meas.spin" class="Ref (strict)"("Value"=w457) -> ()  [unwired: 2 in, 2 out]
                      n210 = Write to Binary File(file (use dialog)=w473, data=w463, error in=w472) -> (refnum out=w468:refnum<file>, error out=w471:errorcluster)  [unwired: 3 in, 1 out]
                      n211 = property on="Time.spin" class="Ref (strict)"("Value"=w458) -> ()  [unwired: 2 in, 2 out]
                      n212 = Write to Binary File(file (use dialog)=w468, data=w462, error in=w471) -> (refnum out=w469:refnum<file>, error out=w470:errorcluster)  [unwired: 3 in, 1 out]
                    }
                    frame True {
                      n213 = property on="Meas.spin" class="Ref (strict)"() -> ("Value"=w493:refnum<file>)  [unwired: 2 in, 2 out]
                      n214 = property on="Time.spin" class="Ref (strict)"() -> ("Value"=w492:refnum<file>)  [unwired: 2 in, 2 out]
                    }
                  }
                  n215 = To Unsigned Word Integer(number=w427) -> (unsigned 16bit integer=w430:u16[][][])
                  n216 = Merge Errors(w433, w434) -> (w432:errorcluster)
                  n217 = Set File Position(refnum=w436, from (0:start)=w442, error in=w432) -> (refnum out=w448:refnum<file>, error out=w447:errorcluster)  [unwired: 1 in]
                  n218 = Set File Position(refnum=w435, from (0:start)=w442, error in=w432) -> (refnum out=w453:refnum<file>, error out=w452:errorcluster)  [unwired: 1 in]
                  n219 = Write to Binary File(file (use dialog)=w453, data=w431, error in=w452, 5:w429) -> (error out=w437:errorcluster)  [unwired: 2 in, 2 out]
                  n220 = Write to Binary File(file (use dialog)=w448, data=w430, error in=w447, 5:w429) -> (error out=w438:errorcluster)  [unwired: 2 in, 2 out]
                  n221 = Merge Errors(w438, w437) -> (w444:errorcluster)
                }
                frame "Transfer_Settings" {
                  n222 = Unbundle By Name(w500) -> ("Device Information"=w499:string[])
                }
              }
              n223 = feedback-in #2(w313) -> ()
            }
            n224 = Release Queue(queue=w302) -> ()  [unwired: 2 in, 3 out]
          }
          frame "Measure_Spectrum" {
            w505 = T8 {"QueueAction"=enum."TimeOut", "Data"=[], "Data_Raw"=[], "Data_Dark"=[], "Data_Ref"=[], "Device Information"=[], "Numeric Control"=0.0, "Boolean"=FALSE, "Wavelength"=[], "Time"=[], "Time Stamp"=timestamp(0 s since 1904-01-01), "Numeric Control 2"=0.0, "TabControl"=enum."Measure", "Numeric Control 3"=0.0}  # DataQueue
            n225 = Obtain Queue(name (unnamed)="Temp", element data type=w505) -> (queue out=w504:refnum<queue>)  [unwired: 3 in, 2 out]
            n226 = while {
              shift-right: [w514] -> w508
              shift-left: w509 -> [w522]
              shift-right: [w515] -> w507
              shift-left: w510 -> [w523]
              shift-right: [w516] -> w503
              shift-left: w504 -> [w518]
              tunnel: w502 -> [w512]
              stop <- w513 stop-if-true
              n227 = Dequeue Element(queue=w522, error in (no error)=w523) -> (queue out=w520:refnum<queue>, element=w517:T8, error out=w519:errorcluster)  [unwired: 1 in, 1 out]
              n228 = Unbundle By Name(w517) -> ("QueueAction"=w521:T9, "TabControl"=w511:T10)
              n229 = case shown="\"Stop_Measurement\"" w521 {
                tunnel: w520 -> [w524 w556 w594]
                tunnel: w519 -> [w527 w564 w593]
                tunnel: w518 -> [w529 w570 w596]
                tunnel: w517 -> [w525 w546 _]
                tunnel: [w528 w570 w592] -> w516
                tunnel: [w526 w557 w590] -> w515
                tunnel: [w524 w556 w591] -> w514
                tunnel: [_ _ TRUE] -> w513
                tunnel: w512 -> [_ w549 _]
                tunnel: w511 -> [_ w544 w588]
                frame Default {
                  n230 = Enqueue Element(queue=w529, element=w525, error in (no error)=w527) -> (queue out=w528:refnum<queue>, error out=w526:errorcluster)  [unwired: 1 in, 1 out]
                }
                frame "Spectrometer_Measure" {
                  n231 = Unbundle By Name(w546) -> ("Data_Raw"=w563:T14)
                  n232 = case shown="\"Measure\", Default" w544 {
                    tunnel: [w583 "SpectralStability_SavePath"] -> w537
                    tunnel: [w582 "SpectralStability_FileName"] -> w535
                    tunnel: [w578 "SpectralStability_Comments"] -> w538
                    frame "Measure", Default {
                      n233 = property on="Spectra Count" class="DigNum (strict)"() -> ("Value"=w584:u16)  [unwired: 2 in, 2 out]
                      n234 = property on="Measure_SavePath" class="Path"() -> ("Value"=w583:path)  [unwired: 2 in, 2 out]
                      n235 = property on="Measure_Comments" class="Str"() -> ("Value"=w578:string)  [unwired: 2 in, 2 out]
                      n236 = property on="Measure_FileName" class="Str"() -> ("Value"=w579:string)  [unwired: 2 in, 2 out]
                      n237 = Number To Decimal String(number=w584) -> (decimal integer string=w580:string)  [unwired: 1 in]
                      n238 = Concatenate Strings(w579, "_", w580) -> (w582:string)
                    }
                    frame "Spectral Stability" {
                    }
                  }
                  n239 = Index Array(array=w563, index=0) -> (element=w561:T15)
                  n240 = Unbundle By Name(w546) -> ("Time Stamp"=w545:timestamp)
                  n241 = Unbundle By Name(w561) -> ("Image"=w540:dbl[][][])
                  n242 = Index Array(array=w540, index (dim 1)=0 ("disabled index (row)")) -> (element=w555:dbl[][])  [unwired: 2 in]
                  n243 = Transpose 2D Array(2D array=w555) -> (transposed array=w552:dbl[][])
                  n244 = Format Date/Time String(time format string (%c)="%Y%m%d_%H%M%S", seconds (now)=w545) -> (date/time string=w568:string)  [unwired: 1 in]
                  n245 = Matrix Size(0:w552) -> (2:w553:i32)  [unwired: 1 out]
                  n246 = Empty String/Path?(string/path=w538) -> (empty?=w539:bool)
                  n247 = Reciprocal(x=w553) -> (1/x=w554:dbl)
                  n248 = Concatenate Strings(w568, "_") -> (w536:string)
                  n249 = case shown="False" w539 {
                    tunnel: w538 -> [w577 _]
                    tunnel: w537 -> [w576 _]
                    tunnel: w536 -> [w575 _]
                    tunnel: w535 -> [w574 _]
                    frame False {
                      n250 = Concatenate Strings(w575, w574, "_comments.txt" ("string")) -> (w571:string)
                      n251 = Build Path(base path=w576, name or relative path=w571) -> (appended path=w572:path)
                      n252 = Write to Text File(file (use dialog)=w572, text=w577) -> ()  [unwired: 2 in, 3 out]
                    }
                    frame True {
                    }
                  }
                  n253 = Initialize Array(w554, w553) -> (w551:dbl[])
                  n254 = Concatenate Strings(w536, w535, ".spectra" ("string")) -> (w542:string)
                  n255 = Unbundle By Name(w549) -> ("Wavlength"=w530:dbl[unit][])
                  n256 = call-poly <vilib>:"A x B.vi"("Vector"=w551, "A"=w552) -> ("A x Vector"=w541:dbl[])  [unwired: 1 out]
                  n257 = Build Path(base path=w537, name or relative path=w542) -> (appended path=w566:path)
                  n258 = Bundle("Wavlength"=w530, "A x Vector"=w541) -> (w548:T16)  [unwired: 1 in]
                  n259 = Open/Create/Replace File(file path (use dialog)=w566, error in=w564, operation (0:open)=T13."open or create") -> (refnum out=w531:refnum<file>, error out=w534:errorcluster)  [unwired: 3 in, 1 out]
                  n260 = Build Array(w548) -> (w547:T17)
                  n261 = property on="Measure_Graph" class="XYGraph (strict)"("Value"=w547) -> ()  [unwired: 2 in, 2 out]
                  n262 = Write to Binary File(file (use dialog)=w531, data=w530, error in=w534) -> (refnum out=w532:refnum<file>, error out=w533:errorcluster)  [unwired: 3 in, 1 out]
                  n263 = To Unsigned Word Integer(number=w540) -> (unsigned 16bit integer=w560:u16[][][])
                  n264 = Write to Binary File(file (use dialog)=w532, data=w560, error in=w533) -> (refnum out=w558:refnum<file>, error out=w559:errorcluster)  [unwired: 3 in, 1 out]
                  n265 = Close File(refnum=w558, error in=w559) -> (error out=w557:errorcluster)  [unwired: 1 out]
                }
                frame "Stop_Measurement" {
                  w589 = FALSE ("Measure Spectrum")
                  n266 = case shown="Default" w588 {
                    frame Default {
                    }
                    frame "Measure" {
                      n267 = property on="Automatically \nadjust count" class="Bool (strict)"() -> ("Value"=w599:bool)  [unwired: 2 in, 2 out]
                      n268 = case shown="True" w599 {
                        frame False {
                        }
                        frame True {
                          n269 = Increment(x="Spectra Count") -> (x+1=w600:u16)
                          n270 = property on="Spectra Count" class="DigNum (strict)"("Value"=w600) -> ()  [unwired: 2 in, 2 out]
                        }
                      }
                    }
                  }
                  n271 = Get Queue Status(queue=w596) -> (queue out=w597:refnum<queue>, # elements in queue=w595:i32)  [unwired: 2 in, 6 out]
                  n272 = property on="SpectralStability_MeasureSpectrum" class="Bool (strict)"("Value"=w589) -> ()  [unwired: 2 in, 2 out]
                  n273 = property on="Measure_MeasureSpectrum" class="Bool (strict)"("Value"=w589) -> ()  [unwired: 2 in, 2 out]
                  n274 = for {
                    N: w595 -> [_]
                    shift-right: [w607] -> w592
                    shift-left: w597 -> [w608]
                    shift-right: [w604] -> w591
                    shift-left: w594 -> [w605]
                    shift-right: [w602] -> w590
                    shift-left: w593 -> [w603]
                    n275 = Dequeue Element(queue=w608) -> (queue out=w607:refnum<queue>, element=w606:T8)  [unwired: 2 in, 2 out]
                    n276 = Enqueue Element(queue=w605, element=w606, error in (no error)=w603) -> (queue out=w604:refnum<queue>, error out=w602:errorcluster)  [unwired: 1 in, 1 out]
                  }
                }
              }
            }
            n277 = Release Queue(queue=w503) -> ()  [unwired: 2 in, 3 out]
          }
          frame "Measure_SpectrumAdvanced" {
            w612 = T8 {"QueueAction"=enum."TimeOut", "Data"=[], "Data_Raw"=[], "Data_Dark"=[], "Data_Ref"=[], "Device Information"=[], "Numeric Control"=0.0, "Boolean"=FALSE, "Wavelength"=[], "Time"=[], "Time Stamp"=timestamp(0 s since 1904-01-01), "Numeric Control 2"=0.0, "TabControl"=enum."Measure", "Numeric Control 3"=0.0}  # DataQueue
            n278 = Obtain Queue(name (unnamed)="Temp", element data type=w612) -> (queue out=w611:refnum<queue>)  [unwired: 3 in, 2 out]
            n279 = while {
              shift-right: [w620] -> w615
              shift-left: w616 -> [w628]
              shift-right: [w621] -> w614
              shift-left: w617 -> [w629]
              shift-right: [w622] -> w610
              shift-left: w611 -> [w624]
              tunnel: w609 -> [w618]
              stop <- w619 stop-if-true
              n280 = Dequeue Element(queue=w628, error in (no error)=w629) -> (queue out=w626:refnum<queue>, element=w623:T8, error out=w625:errorcluster)  [unwired: 1 in, 1 out]
              n281 = Unbundle By Name(w623) -> ("QueueAction"=w627:T9)
              n282 = case shown="\"Spectrometer_Measure\"" w627 {
                tunnel: w626 -> [w630 w658 w682]
                tunnel: w625 -> [w633 w666 w681]
                tunnel: w624 -> [w635 w675 w684]
                tunnel: w623 -> [w631 w646 _]
                tunnel: [w634 w675 w680] -> w622
                tunnel: [w632 w659 w678] -> w621
                tunnel: [w630 w658 w679] -> w620
                tunnel: [_ _ TRUE] -> w619
                tunnel: w618 -> [_ w650 _]
                frame Default {
                  n283 = Enqueue Element(queue=w635, element=w631, error in (no error)=w633) -> (queue out=w634:refnum<queue>, error out=w632:errorcluster)  [unwired: 1 in, 1 out]
                }
                frame "Spectrometer_Measure" {
                  w672 = "_"
                  n284 = Unbundle By Name(w646) -> ("Time Stamp"=w645:timestamp)
                  n285 = property on="Nr After Spin" class="DigNum (strict)"() -> ("Value"=w644:u16)  [unwired: 2 in, 2 out]
                  n286 = Unbundle By Name(w650) -> ("Wavlength"=w636:dbl[unit][])
                  n287 = property on="Measure_FileName" class="Str"() -> ("Value"=w671:string)  [unwired: 2 in, 2 out]
                  n288 = Number To Decimal String(number=w644) -> (decimal integer string=w642:string)  [unwired: 1 in]
                  n289 = Format Date/Time String(time format string (%c)="%Y%m%d_%H%M%S", seconds (now)=w645) -> (date/time string=w673:string)  [unwired: 1 in]
                  n290 = Concatenate Strings(w673, w672, w671, w672, "a" ("string"), w642, ".spectra" ("string")) -> (w670:string)
                  n291 = property on="Measure_SavePath" class="Path"() -> ("Value"=w669:path)  [unwired: 2 in, 2 out]
                  n292 = Build Path(base path=w669, name or relative path=w670) -> (appended path=w668:path)
                  n293 = Unbundle By Name(w646) -> ("Data_Raw"=w665:T14)
                  n294 = Open/Create/Replace File(file path (use dialog)=w668, error in=w666, operation (0:open)=T13."open or create") -> (refnum out=w637:refnum<file>, error out=w638:errorcluster)  [unwired: 3 in, 1 out]
                  n295 = Index Array(array=w665, index=0) -> (element=w663:T15)
                  n296 = Write to Binary File(file (use dialog)=w637, data=w636, error in=w638) -> (refnum out=w640:refnum<file>, error out=w639:errorcluster)  [unwired: 3 in, 1 out]
                  n297 = Unbundle By Name(w663) -> ("Image"=w651:dbl[][][])
                  n298 = Index Array(array=w651, index (dim 1)=0 ("disabled index (row)")) -> (element=w657:dbl[][])  [unwired: 2 in]
                  n299 = Transpose 2D Array(2D array=w657) -> (transposed array=w654:dbl[][])
                  n300 = Matrix Size(0:w654) -> (2:w655:i32)  [unwired: 1 out]
                  n301 = Reciprocal(x=w655) -> (1/x=w656:dbl)
                  n302 = To Unsigned Word Integer(number=w651) -> (unsigned 16bit integer=w662:u16[][][])
                  n303 = Initialize Array(w656, w655) -> (w653:dbl[])
                  n304 = Write to Binary File(file (use dialog)=w640, data=w662, error in=w639) -> (refnum out=w660:refnum<file>, error out=w661:errorcluster)  [unwired: 3 in, 1 out]
                  n305 = call-poly <vilib>:"A x B.vi"("Vector"=w653, "A"=w654) -> ("A x Vector"=w647:dbl[])  [unwired: 1 out]
                  n306 = Bundle("Wavlength"=w636, "A x Vector"=w647) -> (w649:T16)  [unwired: 1 in]
                  n307 = Build Array(w649) -> (w648:T17)
                  n308 = property on="Measure_Graph" class="XYGraph (strict)"("Value"=w648) -> ()  [unwired: 2 in, 2 out]
                  n309 = Close File(refnum=w660, error in=w661) -> (error out=w659:errorcluster)  [unwired: 1 out]
                }
                frame "Stop_Measurement" {
                  n310 = property on="Automatically \nadjust count" class="Bool (strict)"() -> ("Value"=w676:bool)  [unwired: 2 in, 2 out]
                  n311 = case shown="True" w676 {
                    frame False {
                    }
                    frame True {
                      n312 = property on="Nr After Spin" class="DigNum (strict)"() -> ("Value"=w688:u16)  [unwired: 2 in, 2 out]
                      n313 = Increment(x=w688) -> (x+1=w687:u16)
                      n314 = property on="Nr After Spin" class="DigNum (strict)"("Value"=w687) -> ()  [unwired: 2 in, 2 out]
                    }
                  }
                  n315 = Get Queue Status(queue=w684) -> (queue out=w685:refnum<queue>, # elements in queue=w683:i32)  [unwired: 2 in, 6 out]
                  n316 = property on="Measure_MeasureSpectrum" class="Bool (strict)"("Value"=FALSE ("Measure Spectrum")) -> ()  [unwired: 2 in, 2 out]
                  n317 = for {
                    N: w683 -> [_]
                    shift-right: [w694] -> w680
                    shift-left: w685 -> [w695]
                    shift-right: [w691] -> w679
                    shift-left: w682 -> [w692]
                    shift-right: [w689] -> w678
                    shift-left: w681 -> [w690]
                    n318 = Dequeue Element(queue=w695) -> (queue out=w694:refnum<queue>, element=w693:T8)  [unwired: 2 in, 2 out]
                    n319 = Enqueue Element(queue=w692, element=w693, error in (no error)=w690) -> (queue out=w691:refnum<queue>, error out=w689:errorcluster)  [unwired: 1 in, 1 out]
                  }
                }
              }
            }
            n320 = Release Queue(queue=w610) -> ()  [unwired: 2 in, 3 out]
          }
          frame "Measure_SpectralStability" {
            w711 = T8 {"QueueAction"=enum."TimeOut", "Data"=[], "Data_Raw"=[], "Data_Dark"=[], "Data_Ref"=[], "Device Information"=[], "Numeric Control"=0.0, "Boolean"=FALSE, "Wavelength"=[], "Time"=[], "Time Stamp"=timestamp(0 s since 1904-01-01), "Numeric Control 2"=0.0, "TabControl"=enum."Measure", "Numeric Control 3"=0.0}  # DataQueue
            n321 = Unbundle By Name(w700) -> ("Time Stamp"=w706:timestamp)
            n322 = Unbundle By Name(w700) -> ("Numeric Control"=w696:dbl)
            n323 = property on="SpectralStability\n_SavePath" class="Path"() -> ("Value"=w702:path)  [unwired: 2 in, 2 out]
            n324 = property on="SpectralStability\n_FileName" class="Str"() -> ("Value"=w701:string)  [unwired: 2 in, 2 out]
            n325 = Obtain Queue(name (unnamed)="Temp", element data type=w711) -> (queue out=w710:refnum<queue>)  [unwired: 3 in, 2 out]
            n326 = call "Num2Str_TrailingZero.vi"("Numeric Control"=w696) -> ("format string"=w699:string)  [unwired: 10 in]
            n327 = Format Date/Time String(time format string (%c)="%Y%m%d_%H%M%S", seconds (now)=w706) -> (date/time string=w703:string)  [unwired: 1 in]
            n328 = while {
              shift-right: [w716] -> w704
              shift-left: w713 -> [w716]
              shift-right: [w722] -> _
              shift-left: w710 -> [w724]
              border: 0 -> [_]
              shift-right: [w723] -> w697
              shift-left: w708 -> [w732]
              shift-right: [w721] -> w698
              shift-left: w707 -> [w731]
              tunnel: w703 -> [w719]
              tunnel: w702 -> [w718]
              tunnel: w701 -> [w717]
              tunnel: w699 -> [w715]
              tunnel: w696 -> [w714]
              stop <- w720 stop-if-true
              n329 = Dequeue Element(queue=w732, error in (no error)=w731) -> (queue out=w730:refnum<queue>, element=w728:T8, error out=w729:errorcluster)  [unwired: 1 in, 1 out]
              n330 = Unbundle By Name(w728) -> ("QueueAction"=w727:T9)
              n331 = feedback #3() -> (w725:i32)
              n332 = case shown="\"Spectrometer_Measure\"" w727 {
                tunnel: w730 -> [w736 w745 w751 w769 w852 w859]
                tunnel: w729 -> [w735 w742 w752 w770 _ w860]
                tunnel: w728 -> [w737 w741 _ _ w806 w891]
                tunnel: [w739 w747 w758 w776 w790 w892] -> w726
                tunnel: w725 -> [w739 w747 w758 w776 w850 w892]
                tunnel: w724 -> [w738 w746 w754 w772 w851 w869]
                tunnel: [w736 w744 w749 w767 w852 w859] -> w723
                tunnel: [w734 w746 w753 w771 w851 w869] -> w722
                tunnel: [w733 w743 w750 w768 w795 w860] -> w721
                tunnel: [_ TRUE TRUE TRUE _ _] -> w720
                tunnel: w719 -> [_ _ _ _ w848 w889]
                tunnel: w718 -> [_ _ _ _ w815 w857]
                tunnel: w717 -> [_ _ _ _ w847 w887]
                tunnel: w716 -> [_ _ _ _ w822 w886]
                tunnel: w715 -> [_ _ _ _ w849 _]
                tunnel: w714 -> [_ _ _ _ w791 _]
                frame Default {
                  n333 = Enqueue Element(queue=w738, element=w737, error in (no error)=w735) -> (queue out=w734:refnum<queue>, error out=w733:errorcluster)  [unwired: 1 in, 1 out]
                }
                frame "Close_Program" {
                  n334 = Enqueue Element At Opposite End(queue=w745, element=w741, error in (no error)=w742) -> (queue out=w744:refnum<queue>, error out=w743:errorcluster)  [unwired: 1 in, 1 out]
                }
                frame "Abort" {
                  n335 = Get Queue Status(queue=w754) -> (queue out=w756:refnum<queue>, # elements in queue=w757:i32)  [unwired: 2 in, 6 out]
                  n336 = for {
                    N: w757 -> [_]
                    shift-right: [w764] -> w753
                    shift-left: w756 -> [w765]
                    shift-right: [w761] -> w749
                    shift-left: w751 -> [w762]
                    shift-right: [w759] -> w750
                    shift-left: w752 -> [w760]
                    n337 = Dequeue Element(queue=w765) -> (queue out=w764:refnum<queue>, element=w763:T8)  [unwired: 2 in, 2 out]
                    n338 = Enqueue Element(queue=w762, element=w763, error in (no error)=w760) -> (queue out=w761:refnum<queue>, error out=w759:errorcluster)  [unwired: 1 in, 1 out]
                  }
                  n339 = property on="SpectralStability_Record" class="Bool (strict)"("Value"=FALSE ("SpectralStability_Record")) -> ()  [unwired: 2 in, 2 out]
                }
                frame "Stop_Measurement" {
                  n340 = Get Queue Status(queue=w772) -> (queue out=w774:refnum<queue>, # elements in queue=w775:i32)  [unwired: 2 in, 6 out]
                  n341 = for {
                    N: w775 -> [_]
                    shift-right: [w782] -> w771
                    shift-left: w774 -> [w783]
                    shift-right: [w779] -> w767
                    shift-left: w769 -> [w780]
                    shift-right: [w777] -> w768
                    shift-left: w770 -> [w778]
                    n342 = Dequeue Element(queue=w783) -> (queue out=w782:refnum<queue>, element=w781:T8)  [unwired: 2 in, 2 out]
                    n343 = Enqueue Element(queue=w780, element=w781, error in (no error)=w778) -> (queue out=w779:refnum<queue>, error out=w777:errorcluster)  [unwired: 1 in, 1 out]
                  }
                  n344 = property on="SpectralStability_Record" class="Bool (strict)"("Value"=FALSE ("SpectralStability_Record")) -> ()  [unwired: 2 in, 2 out]
                }
                frame "Spectrometer_Measure" {
                  w846 = "_"
                  n345 = Increment(x=w850) -> (x+1=w790:i32)
                  n346 = Unbundle By Name(w806) -> ("Numeric Control 2"=w805:dbl)
                  n347 = Unbundle By Name(w806) -> ("Data_Raw"=w844:T14)
                  n348 = Format Into String(format string=w849, w850) -> (resulting string=w804:string)  [unwired: 2 in, 1 out]
                  n349 = Concatenate Strings(w848, w846, w847, w846) -> (w817:string)
                  n350 = Unbundle By Name(w822) -> ("Wavlength"=w820:dbl[unit][])
                  n351 = Index Array(array=w844, index=0) -> (element=w842:T15)
                  n352 = Divide(x=w790, y=w791) -> (x/y=w794:dbl)
                  n353 = Concatenate Strings(w817, "s" ("string"), w804, ".smean" ("string")) -> (w826:string)
                  n354 = Concatenate Strings(w817, "raw" ("string"), w804, ".spectra" ("string")) -> (w834:string)
                  n355 = Unbundle By Name(w842) -> ("Image"=w830:dbl[][][])
                  n356 = Concatenate Strings(w817, "timing.txt" ("string")) -> (w814:string)
                  n357 = Subtract(x=w791, y=w790) -> (x-y=w786:dbl)
                  "SS_StepsLeft" <- w786
                  n358 = Number To Exponential String(number=w805, 1:FALSE ("use system decimal point (T)")) -> (E-format string=w802:string)  [unwired: 2 in]
                  n359 = Build Path(base path=w815, name or relative path=w826) -> (appended path=w823:path)
                  n360 = Build Path(base path=w815, name or relative path=w814) -> (appended path=w813:path)
                  n361 = Multiply(x=w794, y=100.0) -> (x*y=w793:dbl)
                  n362 = property on="SS:PeriodicTime" class="DigNum (strict)"() -> ("Value"=w788:dbl[unit])  [unwired: 2 in, 2 out]
                  n363 = Build Path(base path=w815, name or relative path=w834) -> (appended path=w831:path)
                  n364 = Index Array(array=w830, index (dim 1)=0 ("disabled index (row)")) -> (element=w841:dbl[][])  [unwired: 2 in]
                  n365 = To Unsigned Byte Integer(number=w793) -> (unsigned 8bit integer=→"Horizontal Progress Bar":u8)
                  n366 = To Unsigned Word Integer(number=w830) -> (unsigned 16bit integer=w829:u16[][][])
                  n367 = Open/Create/Replace File(file path (use dialog)=w813, operation (0:open)=T13."open or create") -> (refnum out=w811:refnum<file>, error out=w808:errorcluster)  [unwired: 4 in, 1 out]
                  n368 = Concatenate Strings(w804, "\t", w802, "\r\n") -> (w801:string)
                  n369 = Transpose 2D Array(2D array=w841) -> (transposed array=w838:dbl[][])
                  n370 = Write to Binary File(file (use dialog)=w831, data=w829) -> (refnum out=w827:refnum<file>, error out=w828:errorcluster)  [unwired: 4 in, 1 out]
                  n371 = Multiply(x=w788, y=w786) -> (x*y=→"SS_TimePrediction":dbl[unit])
                  n372 = Set File Position(refnum=w811, from (0:start)=enum16{"start", "end", "current"}."end", error in=w808) -> (refnum out=w809:refnum<file>, error out=w807:errorcluster)  [unwired: 1 in]
                  n373 = Matrix Size(0:w838) -> (2:w839:i32)  [unwired: 1 out]
                  n374 = Close File(refnum=w827, error in=w828) -> (error out=w798:errorcluster)  [unwired: 1 out]
                  n375 = Reciprocal(x=w839) -> (1/x=w840:dbl)
                  n376 = Write to Text File(file (use dialog)=w809, text=w801, error in=w807) -> (refnum out=w800:refnum<file>, error out=w799:errorcluster)  [unwired: 1 in, 1 out]
                  n377 = Initialize Array(w840, w839) -> (w837:dbl[])
                  n378 = call-poly <vilib>:"A x B.vi"("Vector"=w837, "A"=w838) -> ("A x Vector"=w819:dbl[])  [unwired: 1 out]
                  n379 = Bundle("Wavlength"=w820, "A x Vector"=w819) -> (w821:T16)  [unwired: 1 in]
                  n380 = Close File(refnum=w800, error in=w799) -> (error out=w796:errorcluster)  [unwired: 1 out]
                  n381 = Write to Binary File(file (use dialog)=w823, data=w819) -> (refnum out=w825:refnum<file>, error out=w824:errorcluster)  [unwired: 4 in, 1 out]
                  n382 = Build Array(w821) -> (w818:T17)
                  n383 = Close File(refnum=w825, error in=w824) -> (error out=w797:errorcluster)  [unwired: 1 out]
                  n384 = property on="SpectralStability:\nGraph" class="XYGraph (strict)"("Value"=w818) -> ()  [unwired: 2 in, 2 out]
                  n385 = Merge Errors(w798, w797, w796) -> (w795:errorcluster)
                }
                frame "Transfer_Settings" {
                  w862 = "\r\n"
                  w876 = 0.0
                  w882 = 0 ("index")
                  n386 = Unbundle By Name(w886) -> ("Dark"=w883:T14, "Ref"=w884:T14, "Wavlength"=w885:dbl[unit][])
                  n387 = Concatenate Strings(w889, "_", w887) -> (w875:string)
                  n388 = property on="SpectralStability_\nPeriodicTime" class="DigNum (strict)"() -> ("Value"=w868:dbl[unit])  [unwired: 2 in, 2 out]
                  n389 = Unbundle By Name(w891) -> ("Device Information"=w890:string[])
                  n390 = property on="SpectralStability_Duration" class="DigNum (strict)"() -> ("Value"=w867:dbl[unit])  [unwired: 2 in, 2 out]
                  n391 = Index Array(array=w883, index=w882) -> (element=w880:T15)
                  n392 = Index Array(array=w884, index=w882) -> (element=w881:T15)
                  n393 = Concatenate Strings(w875, "_add.spin" ("string")) -> (w872:string)
                  n394 = Concatenate Strings(w875, "_comments.txt" ("string")) -> (w858:string)
                  n395 = Unbundle By Name(w880) -> ("Image"=w854:dbl[][][])
                  n396 = Unbundle By Name(w881) -> ("Image"=w853:dbl[][][])
                  n397 = property on="SpectralStability_\nMeasurementNumber" class="DigNum (strict)"() -> ("Value"=w866:u32)  [unwired: 2 in, 2 out]
                  n398 = Build Path(base path=w857, name or relative path=w872) -> (appended path=w871:path)
                  n399 = Build Path(base path=w857, name or relative path=w858) -> (appended path=w856:path)
                  n400 = node(w885) -> (w877:dbl[])
                  n401 = property on="Duration/Times" class="Bool (strict)"() -> ("Value"=w865:bool)  [unwired: 2 in, 2 out]
                  n402 = To Unsigned Word Integer(number=w854) -> (unsigned 16bit integer=w879:u16[][][])
                  n403 = To Unsigned Word Integer(number=w853) -> (unsigned 16bit integer=w878:u16[][][])
                  n404 = call "DeviceInfo2Str.vi"("Device Information"=w890) -> ("String"=w864:string)  [unwired: 10 in]
                  n405 = property on="SpectralStability:\nComments" class="Str"() -> ("Value"=w861:string)  [unwired: 2 in, 2 out]
                  n406 = Bundle(w879, w878, w877, w876, w876) -> (w870:cluster{u16[][][], u16[][][], dbl[], dbl, dbl})  [unwired: 1 in]
                  n407 = call "String_SpectralStabilitySettings.vi"("Duration/Times"=w865, "Measurement Number"=w866, "Duration"=w867, "Periodic Time"=w868) -> ("String"=w863:string)  [unwired: 7 in]
                  n408 = Concatenate Strings(w864, w862, w863, w862, w861) -> (w855:string)
                  n409 = Write to Binary File(file (use dialog)=w871, data=w870) -> ()  [unwired: 4 in, 3 out]
                  n410 = Write to Text File(file (use dialog)=w856, text=w855) -> ()  [unwired: 2 in, 3 out]
                }
              }
              n411 = feedback-in #3(w726) -> ()
            }
          }
          frame "Save_InSitu" {
            w910 = "\r\n"
            n412 = Unbundle By Name(w944) -> ("Time Stamp"=w942:timestamp, "Device Information"=w934:string[], "Numeric Control"=w931:dbl, "Numeric Control 2"=w930:dbl, "Numeric Control 3"=w894:dbl)
            n413 = case shown="0, Default" w894 {
              tunnel: ["In-Situ Normal:\n" ("string") "In-Situ Short\n" ("string")] -> w893
              frame 0, Default {
              }
              frame 1 {
              }
            }
            n414 = Unbundle By Name(w932) -> ("Dark"=w950:T14, "Ref"=w948:T14, "Wavlength Trim"=w952:dbl[unit][])
            n415 = property on="Threshold" class="DigNum (strict)"() -> ("Value"=w895:dbl)  [unwired: 2 in, 2 out]
            n416 = node(w952) -> (w945:dbl[])
            n417 = property on="Frames" class="DigNum (strict)"() -> ("Value"=w918:i32)  [unwired: 2 in, 2 out]
            n418 = property on="Wavelenght Detect" class="DigNum (strict)"() -> ("Value"=w896:dbl[unit])  [unwired: 2 in, 2 out]
            n419 = call "DeviceInfo2Str.vi"("Device Information"=w934) -> ("String"=w933:string)  [unwired: 10 in]
            n420 = Number To Decimal String(number=w918) -> (decimal integer string=w917:string)  [unwired: 1 in]
            n421 = Index Array(array=w948, index=0) -> (element=w946:T15)
            n422 = property on="Time Detect" class="DigNum (strict)"() -> ("Value"=w897:dbl[unit])  [unwired: 2 in, 2 out]
            n423 = property on="LowerWLLimit" class="DigNum (strict)"() -> ("Value"=w906:i32)  [unwired: 2 in, 2 out]
            n424 = Index Array(array=w950, index=0) -> (element=w947:T15)
            n425 = property on="Measure_FileName" class="Str"() -> ("Value"=w927:string)  [unwired: 2 in, 2 out]
            n426 = property on="Spin Time" class="DigNum (strict)"() -> ("Value"=w898:dbl[unit])  [unwired: 2 in, 2 out]
            n427 = property on="Seconds to Spin_Normal" class="DigNum (strict)"() -> ("Value"=w900:dbl[unit])  [unwired: 2 in, 2 out]
            n428 = Unbundle By Name(w947) -> ("Image"=w907:dbl[][][])
            n429 = Unbundle By Name(w946) -> ("Image"=w908:dbl[][][])
            n430 = property on="UpperWLLimit" class="DigNum (strict)"() -> ("Value"=w905:i32)  [unwired: 2 in, 2 out]
            n431 = Format Date/Time String(time format string (%c)="%Y%m%d_%H%M%S", seconds (now)=w942) -> (date/time string=w941:string)  [unwired: 1 in]
            n432 = property on="Seconds after Spin" class="DigNum (strict)"() -> ("Value"=w899:dbl[unit])  [unwired: 2 in, 2 out]
            n433 = Concatenate Strings(w941, "_" ("string"), w927) -> (w939:string)
            n434 = property on="Program Spin Coater" class="Arr (strict)"() -> ("Value"=w916:T2)  [unwired: 2 in, 2 out]
            n435 = call "Trim_Spectra.vi"("WL_UpperIndex"=w905, "WL_LowerIndex"=w906, "Image"=w908) -> ("ImageCut"=w903:dbl[][][])
            n436 = call "Trim_Spectra.vi"("WL_UpperIndex"=w905, "WL_LowerIndex"=w906, "Image"=w907) -> ("ImageCut"=w904:dbl[][][])
            n437 = call "MeasurementSpin2String_v02.vi"("Program Spin Coater"=w916, "Seconds to Spin Start"=w900, "Seconds after Spin Stop"=w899, "Spin Time"=w898, "Time Detect"=w897, "Wavelength Detect"=w896, "Threshold"=w895) -> ("concatenated string"=w915:string)  [unwired: 8 in]
            n438 = To Unsigned Word Integer(number=w903) -> (unsigned 16bit integer=w920:u16[][][])
            n439 = To Unsigned Word Integer(number=w904) -> (unsigned 16bit integer=w921:u16[][][])
            n440 = property on="Duration after" class="DigNum (strict)"() -> ("Value"=w912:dbl[unit])  [unwired: 2 in, 2 out]
            n441 = property on="periodic time" class="DigNum (strict)"() -> ("Value"=w913:dbl[unit])  [unwired: 2 in, 2 out]
            n442 = property on="Spin at end" class="Bool (strict)"() -> ("Value"=w911:bool)  [unwired: 2 in, 2 out]
            n443 = call "AfterSpinOptions.vi"("Spin at end"=w911, "Duration after"=w912, "periodic time"=w913) -> ("concatenated string"=w914:string)  [unwired: 8 in]
            n444 = Concatenate Strings(w893, w933, w910, "Frames:\t" ("string"), w917, w910, w915, w910, w914, w910, "Comments:" ("string"), w910, "Measure_Comments") -> (w929:string)
            n445 = Bundle(w921, w920, w945, "Numeric Control"=w931, "Numeric Control 2"=w930) -> (w924:T18)  [unwired: 1 in]
            n446 = property on="Measure_SavePath" class="Path"() -> ("Value"=w926:path)  [unwired: 2 in, 2 out]
            n447 = Concatenate Strings(w939, "_add.spin" ("string")) -> (w938:string)
            n448 = Concatenate Strings(w939, "_comments.txt" ("string")) -> (w937:string)
            n449 = Build Path(base path=w926, name or relative path=w938) -> (appended path=w925:path)
            n450 = Build Path(base path=w926, name or relative path=w937) -> (appended path=w936:path)
            n451 = Write to Text File(file (use dialog)=w936, text=w929) -> (error out=w923:errorcluster)  [unwired: 2 in, 2 out]
            n452 = Write to Binary File(file (use dialog)=w925, data=w924) -> (error out=w922:errorcluster)  [unwired: 4 in, 2 out]
            n453 = flat-sequence {
              tunnel: w923 -> [_]
              tunnel: w922 -> [_]
              frame #0 {
                n454 = property on="Action" class="Str"("Value"="" ("Action")) -> ()  [unwired: 2 in, 2 out]
              }
            }
            n455 = property on="Action" class="Str"("Value"="Saving" ("Action")) -> ()  [unwired: 2 in, 2 out]
          }
          frame "Set_Dark" {
            # "Averaging"
            n456 = Unbundle By Name(w969) -> ("Wavlength"=w968:dbl[unit][])
            n457 = Unbundle By Name(w976) -> ("Data_Dark"=w966:T14)
            n458 = Index Array(array=w966, index=0) -> (element=w971:T15)
            n459 = Unbundle By Name(w971) -> ("Image"=w965:dbl[][][])
            n460 = Index Array(array=w965, index (dim 1)=0 ("disabled index (row)")) -> (element=w963:dbl[][])  [unwired: 2 in]
            n461 = Transpose 2D Array(2D array=w963) -> (transposed array=w960:dbl[][])
            n462 = Matrix Size(0:w960) -> (2:w961:i32)  [unwired: 1 out]
            n463 = Reciprocal(x=w961) -> (1/x=w962:dbl)
            n464 = Initialize Array(w962, w961) -> (w959:dbl[])
            n465 = call-poly <vilib>:"A x B.vi"("Vector"=w959, "A"=w960) -> ("A x Vector"=w958:dbl[])  [unwired: 1 out]
            n466 = Bundle("Wavlength"=w968, "A x Vector"=w958) -> (w970:T16)  [unwired: 1 in]
            n467 = Build Array(w970) -> (w967:T17)
            n468 = property on="Measure_Graph" class="XYGraph (strict)"("Value"=w967) -> ()  [unwired: 2 in, 2 out]
            n469 = Bundle By Name(cluster=w969, "Dark"=w966) -> (w973:T5)
          }
          frame "Set_Ref" {
            # "Averaging"
            n470 = Unbundle By Name(w978) -> ("Wavlength"=w977:dbl[unit][])
            n471 = Unbundle By Name(w995) -> ("Data_Ref"=w982:T14)
            n472 = Index Array(array=w982, index=0) -> (element=w990:T15)
            n473 = Unbundle By Name(w990) -> ("Image"=w989:dbl[][][])
            n474 = Index Array(array=w989, index (dim 1)=0 ("disabled index (row)")) -> (element=w987:dbl[][])  [unwired: 2 in]
            n475 = Transpose 2D Array(2D array=w987) -> (transposed array=w984:dbl[][])
            n476 = Matrix Size(0:w984) -> (2:w985:i32)  [unwired: 1 out]
            n477 = Reciprocal(x=w985) -> (1/x=w986:dbl)
            n478 = Initialize Array(w986, w985) -> (w983:dbl[])
            n479 = call-poly <vilib>:"A x B.vi"("Vector"=w983, "A"=w984) -> ("A x Vector"=w979:dbl[])  [unwired: 1 out]
            n480 = Bundle("Wavlength"=w977, "A x Vector"=w979) -> (w981:T16)  [unwired: 1 in]
            n481 = Build Array(w981) -> (w980:T17)
            n482 = Bundle By Name(cluster=w978, "Ref"=w982) -> (w992:T5)
            n483 = property on="Measure_Graph" class="XYGraph (strict)"("Value"=w980) -> ()  [unwired: 2 in, 2 out]
          }
          frame "Set_Wavelength" {
            n484 = Unbundle By Name(w999) -> ("Wavelength"=w1002:dbl[unit][])
            n485 = Bundle By Name(cluster=w1001, "Wavlength"=w1002) -> (w1000:T5)
            n486 = property on="Trim\nSpec" class="Bool (strict)"() -> ("Value"=w996:bool)  [unwired: 2 in, 2 out]
            n487 = property on="Trim\nSpec" class="Bool (strict)"("Val(Sgnl)"=w996) -> ()  [unwired: 2 in, 2 out]
          }
          frame "Spectrometer_Preview" {
            w1009 = 0 ("index (page)")
            n488 = Unbundle By Name(w1005) -> ("Data_Raw"=w1013:T14)
            n489 = Unbundle By Name(w1014) -> ("Wavlength"=w1008:dbl[unit][])
            n490 = Unbundle By Name(w1005) -> ("TabControl"=w1004:T10)
            n491 = Index Array(array=w1013, index=0) -> (element=w1011:T15)
            n492 = Unbundle By Name(w1011) -> ("Image"=w1010:dbl[][][])
            n493 = Index Array(array=w1010, index (dim 0)=w1009, index (dim 1)=w1009) -> (element=w1007:dbl[])  [unwired: 1 in]
            n494 = Bundle("Wavlength"=w1008, "Image"=w1007) -> (w1006:cluster{"Wavlength":dbl[unit][], "Image":dbl[]})  [unwired: 1 in]
            n495 = Build Array(w1006) -> (w1003:T3)
            n496 = case shown="Default" w1004 {
              tunnel: w1003 -> [w1017 w1018 _]
              frame "Measure" {
                "Measure_Graph" <- w1017
              }
              frame "Spectral Stability" {
                "SpectralStability_Graph" <- w1018
              }
              frame Default {
              }
            }
          }
          frame "Change_TrimSettings" {
            n497 = Unbundle By Name(w1026) -> ("Boolean"=w1025:bool)
            n498 = case shown="True" w1025 {
              tunnel: w1021 -> [w1032 w1050]
              tunnel: w1026 -> [_ w1045]
              tunnel: [0 w1036] -> w1023
              tunnel: [w1030 w1037] -> w1022
              tunnel: [w1028 w1033] -> w1019
              frame False {
                n499 = Unbundle By Name(w1032) -> ("Wavlength"=w1028:dbl[unit][])
                n500 = Array Size(array=w1028) -> (size(s)=w1031:i32)
                n501 = Decrement(x=w1031) -> (x-1=w1030:i32)
              }
              frame True {
                n502 = Unbundle By Name(w1045) -> ("Numeric Control"=w1049:dbl, "Numeric Control 2"=w1043:dbl)
                n503 = Unbundle By Name(w1050) -> ("Wavlength"=w1038:dbl[unit][])
                n504 = node(w1049) -> (w1048:dbl[unit])
                n505 = node(w1043) -> (w1042:dbl[unit])
                n506 = Subtract(x=w1038, y=w1042) -> (x-y=w1041:dbl[unit][])
                n507 = Subtract(x=w1038, y=w1048) -> (x-y=w1047:dbl[unit][])
                n508 = Absolute Value(x=w1041) -> (abs(x)=w1040:dbl[unit][])
                n509 = Absolute Value(x=w1047) -> (abs(x)=w1046:dbl[unit][])
                n510 = Array Max & Min(array=w1040) -> (min index (indices)=w1037:i32)  [unwired: 3 out]
                n511 = Array Max & Min(array=w1046) -> (min index (indices)=w1036:i32)  [unwired: 3 out]
                n512 = Subtract(x=w1037, y=w1036) -> (x-y=w1035:i32)
                n513 = Index Array(array=w1038, index=w1037) -> (element=w1039:dbl[unit])
                n514 = Index Array(array=w1038, index=w1036) -> (element=w1044:dbl[unit])
                n515 = Increment(x=w1035) -> (x+1=w1034:i32)
                n516 = Array Subset(array=w1038, index=w1036, length=w1034) -> (w1033:dbl[unit][])
                n517 = property on="Wl \nLow" class="DigNum (strict)"("Value"=w1044) -> ()  [unwired: 2 in, 2 out]
                n518 = property on="Wl \nUp" class="DigNum (strict)"("Value"=w1039) -> ()  [unwired: 2 in, 2 out]
              }
            }
            "LowerWLLimit" <- w1023
            "UpperWLLimit" <- w1022
            n519 = Bundle By Name(cluster=w1021, "Wavlength Trim"=w1019) -> (w1020:T5)
          }
        }
      }
      frame Error {
        w1056 = T19 4 items=["no dialog", "OK message", "continue or stop message", "OK message + warnings", "continue/stop + warnings"] ("type of dialog (OK msg:1)")
        n520 = call <vilib>:"General Error Handler.vi"("type of dialog (OK msg:1)"=w1056, "error in (no error)"=w1053) -> ("error out"=w1055:errorcluster)  [unwired: 9 in, 4 out]
        n521 = call <vilib>:"Clear Errors.vi"("error in (no error)"=w1055) -> ("error out"=w1052:errorcluster)  [unwired: 5 in, 1 out]
      }
    }
  }
  n522 = while {
    shift-right: [w1059] -> _
    shift-left: w12 -> [w1057]
    shift-right: [w1062] -> _
    shift-left: w8 -> [w1063]
    shift-right: [w1060] -> _
    shift-left: w1 -> [w1061]
    stop <- w1058 stop-if-true
    # "Producer"
    n523 = event shown="[20] \"StartMeasurement_Button\": Value Change" {
      selector: _ -> [_ _ _ _ _ _ _ _ _ _ _ _ _ _ _ _ _ _ _ _ _ _ _ _ _ _ _ _ _ _ _ _ _]
      dyn-events: _ -> [_ _ _ _ _ _ _ _ _ _ _ _ _ _ _ _ _ _ _ _ _ _ _ _ _ _ _ _ _ _ _ _ _]
      timeout: -1 -> [_ _ _ _ _ _ _ _ _ _ _ _ _ _ _ _ _ _ _ _ _ _ _ _ _ _ _ _ _ _ _ _ _]
      tunnel: w1063 -> [w1066 w1081 w1089 w1102 w1117 w1134 w1139 w1154 w1158 w1167 w1179 w1194 w1218 w1222 w1225 w1229 w1238 w1288 w1293 w1337 w1346 w1371 w1380 w1389 w1397 w1403 w1417 w1444 w1461 w1467 w1482 w1523 w1529]
      tunnel: [w1066 w1078 w1088 w1102 w1117 w1134 w1139 w1154 w1158 w1167 w1179 w1194 w1218 w1222 w1225 w1229 w1238 w1288 w1293 w1337 w1345 w1371 w1380 w1389 w1397 w1403 w1415 w1442 w1461 w1467 w1482 w1522 w1529] -> w1062
      tunnel: w1061 -> [w1065 w1080 w1092 w1100 w1114 w1133 w1138 w1151 w1159 w1168 w1180 w1192 w1213 w1221 w1226 w1228 w1235 w1253 w1292 w1329 w1350 w1370 w1379 w1388 w1396 w1402 w1420 w1448 w1462 w1466 w1480 w1515 w1528]
      tunnel: [w1065 w1074 w1083 w1096 w1113 w1131 w1138 w1150 w1160 w1169 w1181 w1190 w1212 w1221 w1226 w1228 w1233 w1270 w1290 w1313 w1344 w1365 w1376 w1385 w1396 w1402 w1420 w1448 w1462 w1466 w1477 w1515 w1527] -> w1060
      tunnel: w1057 -> [w1067 w1082 w1093 w1101 w1116 w1135 w1140 w1153 w1162 w1171 w1183 w1193 w1215 w1223 w1224 w1230 w1236 w1276 w1294 w1330 w1352 w1372 w1381 w1390 w1398 w1404 w1413 w1449 w1460 w1468 w1481 w1526 w1531]
      tunnel: [w1067 w1079 w1091 w1097 w1115 w1132 w1140 w1152 w1161 w1170 w1182 w1191 w1214 w1223 w1224 w1230 w1237 w1269 w1291 w1312 w1351 w1366 w1377 w1386 w1398 w1401 w1408 w1447 w1460 w1468 w1478 w1526 w1530] -> w1059
      tunnel: [_ TRUE _ _ _ _ _ _ _ _ _ _ _ _ _ _ _ _ _ _ _ _ _ _ _ _ _ _ _ _ _ _ _] -> w1058
      event Timeout {
        n524 = event-data() -> ()  [unwired: 1 in, 3 out]
      }
      event "Stop Button": Value Change {
        w1070 = T8 {"QueueAction"=enum."TimeOut", "Data"=[], "Data_Raw"=[], "Data_Dark"=[], "Data_Ref"=[], "Device Information"=[], "Numeric Control"=0.0, "Boolean"=FALSE, "Wavelength"=[], "Time"=[], "Time Stamp"=timestamp(0 s since 1904-01-01), "Numeric Control 2"=0.0, "TabControl"=enum."Measure", "Numeric Control 3"=0.0}  # DataQueue
        w1073 = T11 {"QueueAction"=enum."TimeOut", "Numeric 1"=0.0, "Numeric 2"=0.0, "Boolean 1"=FALSE, "Boolean 2"=FALSE, "Spin Program"=[], "Spin Prg v07"=[], "Time Stamp"=timestamp(0 s since 1904-01-01), "TabControl"=enum."Measure"}  # Device Queue
        n525 = event-data() -> ()  [unwired: 1 in, 6 out]
        n526 = Bundle By Name(cluster=w1073, "QueueAction"=DeviceQueue_Action."Close_Program") -> (w1071:T11)
        n527 = Enqueue Element At Opposite End(queue=w1082, element=w1071, error in (no error)=w1080) -> (queue out=w1079:refnum<queue>, error out=w1075:errorcluster)  [unwired: 1 in, 1 out]
        n528 = Bundle By Name(cluster=w1070, "QueueAction"=DataQueue_Action."Close_Program") -> (w1068:T8)
        n529 = Enqueue Element At Opposite End(queue=w1081, element=w1068, error in (no error)=w1080) -> (queue out=w1078:refnum<queue>, error out=w1076:errorcluster)  [unwired: 1 in, 1 out]
        n530 = Merge Errors(w1076, w1075) -> (w1074:errorcluster)
      }
      event "Abort Button": Value Change {
        w1087 = T8 {"QueueAction"=enum."TimeOut", "Data"=[], "Data_Raw"=[], "Data_Dark"=[], "Data_Ref"=[], "Device Information"=[], "Numeric Control"=0.0, "Boolean"=FALSE, "Wavelength"=[], "Time"=[], "Time Stamp"=timestamp(0 s since 1904-01-01), "Numeric Control 2"=0.0, "TabControl"=enum."Measure", "Numeric Control 3"=0.0}  # DataQueue
        w1095 = T11 {"QueueAction"=enum."TimeOut", "Numeric 1"=0.0, "Numeric 2"=0.0, "Boolean 1"=FALSE, "Boolean 2"=FALSE, "Spin Program"=[], "Spin Prg v07"=[], "Time Stamp"=timestamp(0 s since 1904-01-01), "TabControl"=enum."Measure"}  # Device Queue
        n531 = event-data() -> ()  [unwired: 1 in, 6 out]
        n532 = Bundle By Name(cluster=w1095, "QueueAction"=DeviceQueue_Action."Abort") -> (w1094:T11)
        n533 = Bundle By Name(cluster=w1087, "QueueAction"=DataQueue_Action."Abort") -> (w1085:T8)
        n534 = Enqueue Element At Opposite End(queue=w1093, element=w1094, error in (no error)=w1092) -> (queue out=w1091:refnum<queue>, error out=w1084:errorcluster)  [unwired: 1 in, 1 out]
        n535 = Enqueue Element At Opposite End(queue=w1089, element=w1085, error in (no error)=w1084) -> (queue out=w1088:refnum<queue>, error out=w1083:errorcluster)  [unwired: 1 in, 1 out]
      }
      event "Init_Spectrometer": Value Change {
        n536 = event-data() -> ()  [unwired: 1 in, 6 out]
        n537 = case shown="False" "Init_Spectrometer" {
          tunnel: [w1104 w1107] -> w1098
          frame True {
            n538 = property on="Tab Control" class="TabCtl (strict)"() -> ("Value"=w1103:T1)  [unwired: 2 in, 2 out]
            n539 = Bundle By Name(cluster=T11 {"QueueAction"=enum."TimeOut", "Numeric 1"=0.0, "Numeric 2"=0.0, "Boolean 1"=FALSE, "Boolean 2"=FALSE, "Spin Program"=[], "Spin Prg v07"=[], "Time Stamp"=timestamp(0 s since 1904-01-01), "TabControl"=enum."Measure"} ("element"), "QueueAction"=DeviceQueue_Action."Spectrometer_Init", "TabControl"=w1103) -> (w1104:T11)
          }
          frame False {
            n540 = Bundle By Name(cluster=T11 {"QueueAction"=enum."TimeOut", "Numeric 1"=0.0, "Numeric 2"=0.0, "Boolean 1"=FALSE, "Boolean 2"=FALSE, "Spin Program"=[], "Spin Prg v07"=[], "Time Stamp"=timestamp(0 s since 1904-01-01), "TabControl"=enum."Measure"} ("element"), "QueueAction"=DeviceQueue_Action."Spectrometer_Close") -> (w1107:T11)
          }
        }
        n541 = Enqueue Element(queue=w1101, element=w1098, error in (no error)=w1100) -> (queue out=w1097:refnum<queue>, error out=w1096:errorcluster)  [unwired: 1 in, 1 out]
      }
      event "Init_Arduino": Value Change {
        # "Shutter is closed after init"
        n542 = event-data() -> ("NewVal"=w1112:bool)  [unwired: 1 in, 5 out]
        n543 = case shown="True" w1112 {
          tunnel: [w1118 w1121] -> w1111
          frame False {
            w1120 = T11 {"QueueAction"=enum."TimeOut", "Numeric 1"=0.0, "Numeric 2"=0.0, "Boolean 1"=FALSE, "Boolean 2"=FALSE, "Spin Program"=[], "Spin Prg v07"=[], "Time Stamp"=timestamp(0 s since 1904-01-01), "TabControl"=enum."Measure"}  # Device Queue
            n544 = Bundle By Name(cluster=w1120, "QueueAction"=DeviceQueue_Action."Arduino_Close") -> (w1118:T11)
          }
          frame True {
            w1123 = T11 {"QueueAction"=enum."TimeOut", "Numeric 1"=0.0, "Numeric 2"=0.0, "Boolean 1"=FALSE, "Boolean 2"=FALSE, "Spin Program"=[], "Spin Prg v07"=[], "Time Stamp"=timestamp(0 s since 1904-01-01), "TabControl"=enum."Measure"}  # Device Queue
            n545 = Bundle By Name(cluster=w1123, "QueueAction"=DeviceQueue_Action."Arduino_Init") -> (w1121:T11)
          }
        }
        n546 = property on="Shutter Toggle" class="Bool (strict)"("Value"=FALSE ("Shutter Toggle")) -> ()  [unwired: 2 in, 2 out]
        n547 = Enqueue Element(queue=w1116, element=w1111, error in (no error)=w1114) -> (queue out=w1115:refnum<queue>, error out=w1113:errorcluster)  [unwired: 1 in, 1 out]
      }
      event "Program Spin Coater": Value Change {
        w1137 = T11 {"QueueAction"=enum."TimeOut", "Numeric 1"=0.0, "Numeric 2"=0.0, "Boolean 1"=FALSE, "Boolean 2"=FALSE, "Spin Program"=[], "Spin Prg v07"=[], "Time Stamp"=timestamp(0 s since 1904-01-01), "TabControl"=enum."Measure"}  # Device Queue
        n548 = event-data() -> ("NewVal"=w1126:T2)  [unwired: 1 in, 5 out]
        n549 = property on="Seconds to Spin_Normal" class="DigNum (strict)"() -> ("Value"=w1128:dbl[unit])  [unwired: 2 in, 2 out]
        n550 = property on="Spin Time" class="DigNum (strict)"() -> ("Value"=w1125:dbl[unit])  [unwired: 2 in, 2 out]
        n551 = node(w1125) -> (w1124:dbl)
        n552 = node(w1128) -> (w1127:dbl)
        n553 = Bundle By Name(cluster=w1137, "QueueAction"=DeviceQueue_Action."Arduino_LoadProgram", "Spin Prg v07"=w1126, "Numeric 1"=w1127, "Numeric 2"=w1124) -> (w1136:T11)
        n554 = Enqueue Element(queue=w1135, element=w1136, error in (no error)=w1133) -> (queue out=w1132:refnum<queue>, error out=w1131:errorcluster)  [unwired: 1 in, 1 out]
        n555 = property on="Measure_IntegrationTime" class="DigNum (strict)"() -> ("Value"=w1129:dbl[unit])  [unwired: 2 in, 2 out]
        n556 = property on="Measure_IntegrationTime" class="DigNum (strict)"("Val(Sgnl)"=w1129) -> ()  [unwired: 2 in, 2 out]
      }
      event "SHUTTER DEBUG": Value Change {
        n557 = event-data() -> ("NewVal"=w1142:bool)  [unwired: 1 in, 5 out]
        n558 = Select(t=u8 0, s=w1142, f=u8 2) -> (s? t:f=w1141:u8)
        n559 = property on="Shutter Position" class="DigNum (strict)"("DisabledEnum"=w1141) -> ()  [unwired: 2 in, 2 out]
        n560 = property on="Shutter Close" class="Bool (strict)"("DisabledEnum"=w1141) -> ()  [unwired: 2 in, 2 out]
        n561 = property on="Shutter Open" class="Bool (strict)"("DisabledEnum"=w1141) -> ()  [unwired: 2 in, 2 out]
      }
      event "Shutter Position": Value Change {
        w1149 = FALSE ("Shutter Close")
        w1147 = T11 {"QueueAction"=enum."TimeOut", "Numeric 1"=0.0, "Numeric 2"=0.0, "Boolean 1"=FALSE, "Boolean 2"=FALSE, "Spin Program"=[], "Spin Prg v07"=[], "Time Stamp"=timestamp(0 s since 1904-01-01), "TabControl"=enum."Measure"}  # Device Queue
        (unwired) DeviceQueue_Action."Arduino_SetSpeed" ("QueueAction")
        (unwired) T11 {"QueueAction"=enum."TimeOut", "Numeric 1"=0.0, "Numeric 2"=0.0, "Boolean 1"=FALSE, "Boolean 2"=FALSE, "Spin Program"=[], "Spin Prg v07"=[], "Time Stamp"=timestamp(0 s since 1904-01-01), "TabControl"=enum."Measure"}  # Device Queue
        n562 = event-data() -> ("NewVal"=w1145:u16)  [unwired: 1 in, 5 out]
        n563 = property on="Shutter Close" class="Bool (strict)"("Value"=w1149) -> ()  [unwired: 2 in, 2 out]
        n564 = property on="Shutter Open" class="Bool (strict)"("Value"=w1149) -> ()  [unwired: 2 in, 2 out]
        n565 = Bundle By Name(cluster=w1147, "QueueAction"=DeviceQueue_Action."Arduino_Shutter_SetPosition", "Numeric 1"=w1145) -> (w1148:T11)
        n566 = Enqueue Element(queue=w1153, element=w1148, error in (no error)=w1151) -> (queue out=w1152:refnum<queue>, error out=w1150:errorcluster)  [unwired: 1 in, 1 out]
      }
      event "Shutter Close": Value Change {
        w1157 = T11 {"QueueAction"=enum."TimeOut", "Numeric 1"=0.0, "Numeric 2"=0.0, "Boolean 1"=FALSE, "Boolean 2"=FALSE, "Spin Program"=[], "Spin Prg v07"=[], "Time Stamp"=timestamp(0 s since 1904-01-01), "TabControl"=enum."Measure"}  # Device Queue
        (unwired) DeviceQueue_Action."Arduino_SetSpeed" ("QueueAction")
        (unwired) T11 {"QueueAction"=enum."TimeOut", "Numeric 1"=0.0, "Numeric 2"=0.0, "Boolean 1"=FALSE, "Boolean 2"=FALSE, "Spin Program"=[], "Spin Prg v07"=[], "Time Stamp"=timestamp(0 s since 1904-01-01), "TabControl"=enum."Measure"}  # Device Queue
        n567 = event-data() -> ()  [unwired: 1 in, 6 out]
        n568 = property on="Shutter Open" class="Bool (strict)"("Value"=FALSE ("Shutter Open")) -> ()  [unwired: 2 in, 2 out]
        n569 = Bundle By Name(cluster=w1157, "QueueAction"=DeviceQueue_Action."Arduino_Shutter_Close") -> (w1156:T11)
        n570 = Enqueue Element(queue=w1162, element=w1156, error in (no error)=w1159) -> (queue out=w1161:refnum<queue>, error out=w1160:errorcluster)  [unwired: 1 in, 1 out]
      }
      event "Shutter Open": Value Change {
        w1166 = T11 {"QueueAction"=enum."TimeOut", "Numeric 1"=0.0, "Numeric 2"=0.0, "Boolean 1"=FALSE, "Boolean 2"=FALSE, "Spin Program"=[], "Spin Prg v07"=[], "Time Stamp"=timestamp(0 s since 1904-01-01), "TabControl"=enum."Measure"}  # Device Queue
        (unwired) DeviceQueue_Action."Arduino_SetSpeed" ("QueueAction")
        (unwired) T11 {"QueueAction"=enum."TimeOut", "Numeric 1"=0.0, "Numeric 2"=0.0, "Boolean 1"=FALSE, "Boolean 2"=FALSE, "Spin Program"=[], "Spin Prg v07"=[], "Time Stamp"=timestamp(0 s since 1904-01-01), "TabControl"=enum."Measure"}  # Device Queue
        n571 = event-data() -> ()  [unwired: 1 in, 6 out]
        n572 = property on="Shutter Close" class="Bool (strict)"("Value"=FALSE ("Shutter Open")) -> ()  [unwired: 2 in, 2 out]
        n573 = Bundle By Name(cluster=w1166, "QueueAction"=DeviceQueue_Action."Arduino_Shutter_Open") -> (w1165:T11)
        n574 = Enqueue Element(queue=w1171, element=w1165, error in (no error)=w1168) -> (queue out=w1170:refnum<queue>, error out=w1169:errorcluster)  [unwired: 1 in, 1 out]
      }
      event "Shutter Toggle": Value Change {
        w1178 = T11 {"QueueAction"=enum."TimeOut", "Numeric 1"=0.0, "Numeric 2"=0.0, "Boolean 1"=FALSE, "Boolean 2"=FALSE, "Spin Program"=[], "Spin Prg v07"=[], "Time Stamp"=timestamp(0 s since 1904-01-01), "TabControl"=enum."Measure"}  # Device Queue
        (unwired) T11 {"QueueAction"=enum."TimeOut", "Numeric 1"=0.0, "Numeric 2"=0.0, "Boolean 1"=FALSE, "Boolean 2"=FALSE, "Spin Program"=[], "Spin Prg v07"=[], "Time Stamp"=timestamp(0 s since 1904-01-01), "TabControl"=enum."Measure"}  # Device Queue
        n575 = event-data() -> ("NewVal"=w1176:bool)  [unwired: 1 in, 5 out]
        n576 = Select(t=DeviceQueue_Action."Arduino_Shutter_Open" ("QueueAction"), s=w1176, f=DeviceQueue_Action."Arduino_Shutter_Close" ("QueueAction")) -> (s? t:f=w1173:T12)
        n577 = Bundle By Name(cluster=w1178, "QueueAction"=w1173) -> (w1177:T11)
        n578 = Enqueue Element(queue=w1183, element=w1177, error in (no error)=w1180) -> (queue out=w1182:refnum<queue>, error out=w1181:errorcluster)  [unwired: 1 in, 1 out]
      }
      event "Measure_IntegrationTime", "SpectralStability_IntegrationTime": Value Change {
        w1196 = T11 {"QueueAction"=enum."TimeOut", "Numeric 1"=0.0, "Numeric 2"=0.0, "Boolean 1"=FALSE, "Boolean 2"=FALSE, "Spin Program"=[], "Spin Prg v07"=[], "Time Stamp"=timestamp(0 s since 1904-01-01), "TabControl"=enum."Measure"}  # Device Queue
        n579 = event-data() -> ("NewVal"=w1188:dbl[unit])  [unwired: 1 in, 5 out]
        n580 = property on="Calculate Frames_Normal" class="Bool (strict)"() -> ("Value"=w1184:bool)  [unwired: 2 in, 2 out]
        n581 = node(w1188) -> (w1187:dbl)
        n582 = property on="Tab Control" class="TabCtl (strict)"() -> ("Value"=w1186:T1)  [unwired: 2 in, 2 out]
        n583 = property on="Tab Control" class="TabCtl (strict)"() -> ("Value"=w1185:T1)  [unwired: 2 in, 2 out]
        n584 = case shown="\"Measure\"" w1186 {
          tunnel: w1196 -> [w1197 w1203 w1209]
          tunnel: [w1197 w1200 w1206] -> w1195
          tunnel: DeviceQueue_Action."Spectrometer_SetIntegrationTime" ("QueueAction") -> [_ w1202 w1208]
          tunnel: w1187 -> [_ w1201 w1207]
          tunnel: w1185 -> [_ w1199 w1204]
          tunnel: w1184 -> [_ w1198 _]
          frame Default {
          }
          frame "Measure" {
            n585 = Bundle By Name(cluster=w1203, "QueueAction"=w1202, "Numeric 1"=w1201, "Boolean 1"=w1198, "TabControl"=w1199) -> (w1200:T11)
          }
          frame "Spectral Stability" {
            n586 = Bundle By Name(cluster=w1209, "QueueAction"=w1208, "Numeric 1"=w1207, "Boolean 1"=FALSE, "TabControl"=w1204) -> (w1206:T11)
          }
        }
        n587 = Enqueue Element(queue=w1193, element=w1195, error in (no error)=w1192) -> (queue out=w1191:refnum<queue>, error out=w1190:errorcluster)  [unwired: 1 in, 1 out]
      }
      event "Frames": Value Change {
        w1217 = T11 {"QueueAction"=enum."TimeOut", "Numeric 1"=0.0, "Numeric 2"=0.0, "Boolean 1"=FALSE, "Boolean 2"=FALSE, "Spin Program"=[], "Spin Prg v07"=[], "Time Stamp"=timestamp(0 s since 1904-01-01), "TabControl"=enum."Measure"}  # Device Queue
        n588 = event-data() -> ()  [unwired: 1 in, 6 out]
        n589 = Bundle By Name(cluster=w1217, "QueueAction"=DeviceQueue_Action."Spectrometer_SetFrames", "Numeric 1"="Frames") -> (w1216:T11)
        n590 = Enqueue Element(queue=w1215, element=w1216, error in (no error)=w1213) -> (queue out=w1214:refnum<queue>, error out=w1212:errorcluster)  [unwired: 1 in, 1 out]
      }
      event "Seconds to Spin_Normal", "Seconds to Spin_Short": Value Change {
        n591 = event-data() -> ("NewVal"=w1219:dbl[unit])  [unwired: 1 in, 5 out]
        n592 = property on="Seconds to Spin_Short" class="DigNum (strict)"("Value"=w1219) -> ()  [unwired: 2 in, 2 out]
        n593 = property on="Seconds to Spin_Normal" class="DigNum (strict)"("Value"=w1219) -> ()  [unwired: 2 in, 2 out]
        n594 = property on="Program Spin Coater" class="Arr (strict)"() -> ("Value"=w1220:T2)  [unwired: 2 in, 2 out]
        n595 = property on="Program Spin Coater" class="Arr (strict)"("Val(Sgnl)"=w1220) -> ()  [unwired: 2 in, 2 out]
      }
      event "Spin Time": Value Change {
        n596 = event-data() -> ()  [unwired: 1 in, 6 out]
        n597 = property on="Program Spin Coater" class="Arr (strict)"() -> ("Value"=w1227:T2)  [unwired: 2 in, 2 out]
        n598 = property on="Program Spin Coater" class="Arr (strict)"("Val(Sgnl)"=w1227) -> ()  [unwired: 2 in, 2 out]
      }
      event "Seconds after Spin": Value Change {
        n599 = event-data() -> ()  [unwired: 1 in, 6 out]
        n600 = property on="Measure_IntegrationTime" class="DigNum (strict)"() -> ("Value"=w1231:dbl[unit])  [unwired: 2 in, 2 out]
        n601 = property on="Measure_IntegrationTime" class="DigNum (strict)"("Val(Sgnl)"=w1231) -> ()  [unwired: 2 in, 2 out]
      }
      event "Calculate Frames_Normal", "Calculate Frames_Short": Value Change {
        n602 = event-data() -> ("NewVal"=w1232:bool)  [unwired: 1 in, 5 out]
        n603 = case shown="False" w1232 {
          tunnel: [0 2] -> w1234
          tunnel: w1236 -> [w1240 w1249]
          tunnel: [w1240 w1247] -> w1237
          tunnel: w1235 -> [w1239 w1246]
          tunnel: [w1239 w1242] -> w1233
          frame False {
          }
          frame True {
            w1248 = T11 {"QueueAction"=enum."TimeOut", "Numeric 1"=0.0, "Numeric 2"=0.0, "Boolean 1"=FALSE, "Boolean 2"=FALSE, "Spin Program"=[], "Spin Prg v07"=[], "Time Stamp"=timestamp(0 s since 1904-01-01), "TabControl"=enum."Measure"}  # Device Queue
            n604 = property on="Measure_IntegrationTime" class="DigNum (strict)"() -> ("Value"=w1244:dbl[unit])  [unwired: 2 in, 2 out]
            n605 = node(w1244) -> (w1243:dbl)
            n606 = Bundle By Name(cluster=w1248, "QueueAction"=DeviceQueue_Action."Spectrometer_SetIntegrationTime", "Numeric 1"=w1243) -> (w1250:T11)
            n607 = Enqueue Element(queue=w1249, element=w1250, error in (no error)=w1246) -> (queue out=w1247:refnum<queue>, error out=w1242:errorcluster)  [unwired: 1 in, 1 out]
          }
        }
        n608 = property on="Calculate Frames_Short" class="Bool (strict)"("Value"=w1232) -> ()  [unwired: 2 in, 2 out]
        n609 = property on="Calculate Frames_Normal" class="Bool (strict)"("Value"=w1232) -> ()  [unwired: 2 in, 2 out]
        n610 = property on="Frames" class="DigNum (strict)"("DisabledEnum"=w1234) -> ()  [unwired: 2 in, 2 out]
      }
      event "Record RefSpec": Value Change {
        w1257 = T11 {"QueueAction"=enum."TimeOut", "Numeric 1"=0.0, "Numeric 2"=0.0, "Boolean 1"=FALSE, "Boolean 2"=FALSE, "Spin Program"=[], "Spin Prg v07"=[], "Time Stamp"=timestamp(0 s since 1904-01-01), "TabControl"=enum."Measure"}  # Device Queue
        n611 = event-data() -> ()  [unwired: 1 in, 6 out]
        n612 = property on="Shutter Toggle" class="Bool (strict)"("Value"=FALSE ("Shutter Toggle")) -> ()  [unwired: 2 in, 2 out]
        n613 = property on="Frames for Ref/Dark" class="DigNum (strict)"() -> ("Value"=w1266:dbl)  [unwired: 2 in, 2 out]
        n614 = property on="Measure_FramesSpectrometer" class="DigNum (strict)"() -> ("Value"=w1261:dbl)  [unwired: 2 in, 2 out]
        n615 = Bundle By Name(cluster=w1257, "QueueAction"=DeviceQueue_Action."Spectrometer_SetTriggerMode", "Numeric 1"=0.0) -> (w1256:T11)
        n616 = Bundle By Name(cluster=w1256, "QueueAction"=DeviceQueue_Action."Arduino_Shutter_Open") -> (w1252:T11)
        n617 = Bundle By Name(cluster=w1252, "QueueAction"=DeviceQueue_Action."Wait", "Numeric 1"=0.5) -> (w1267:T11)
        n618 = Enqueue Element(queue=w1276, element=w1256, error in (no error)=w1253) -> (queue out=w1258:refnum<queue>, error out=w1254:errorcluster)  [unwired: 1 in, 1 out]
        n619 = Bundle By Name(cluster=w1267, "QueueAction"=DeviceQueue_Action."Spectrometer_SetFrames", "Numeric 1"=w1266) -> (w1265:T11)
        n620 = Enqueue Element(queue=w1258, element=w1252, error in (no error)=w1254) -> (queue out=w1282:refnum<queue>, error out=w1279:errorcluster)  [unwired: 1 in, 1 out]
        n621 = Bundle By Name(cluster=w1265, "QueueAction"=DeviceQueue_Action."Spectrometer_SetReference") -> (w1264:T11)
        n622 = Enqueue Element(queue=w1282, element=w1267, error in (no error)=w1279) -> (queue out=w1281:refnum<queue>, error out=w1278:errorcluster)  [unwired: 1 in, 1 out]
        n623 = Bundle By Name(cluster=w1264, "QueueAction"=DeviceQueue_Action."Arduino_Shutter_Close") -> (w1262:T11)
        n624 = Enqueue Element(queue=w1281, element=w1265, error in (no error)=w1278) -> (queue out=w1280:refnum<queue>, error out=w1277:errorcluster)  [unwired: 1 in, 1 out]
        n625 = Bundle By Name(cluster=w1262, "QueueAction"=DeviceQueue_Action."Spectrometer_SetFrames", "Numeric 1"=w1261) -> (w1260:T11)
        n626 = Enqueue Element(queue=w1280, element=w1264, error in (no error)=w1277) -> (queue out=w1273:refnum<queue>, error out=w1274:errorcluster)  [unwired: 1 in, 1 out]
        n627 = Enqueue Element(queue=w1273, element=w1262, error in (no error)=w1274) -> (queue out=w1271:refnum<queue>, error out=w1272:errorcluster)  [unwired: 1 in, 1 out]
        n628 = Enqueue Element(queue=w1271, element=w1260, error in (no error)=w1272) -> (queue out=w1269:refnum<queue>, error out=w1270:errorcluster)  [unwired: 1 in, 1 out]
      }
      event "Measure_Preview", "SpectralStability_Preview": Value Change {
        n629 = event-data() -> ("NewVal"=w1289:bool)  [unwired: 1 in, 5 out]
        n630 = case shown="False" w1289 {
          tunnel: w1294 -> [w1296 w1301]
          tunnel: w1292 -> [w1295 w1300]
          tunnel: [w1296 w1299] -> w1291
          tunnel: [w1295 w1298] -> w1290
          frame False {
          }
          frame True {
            w1304 = T11 {"QueueAction"=enum."TimeOut", "Numeric 1"=0.0, "Numeric 2"=0.0, "Boolean 1"=FALSE, "Boolean 2"=FALSE, "Spin Program"=[], "Spin Prg v07"=[], "Time Stamp"=timestamp(0 s since 1904-01-01), "TabControl"=enum."Measure"}  # Device Queue
            n631 = property on="Tab Control" class="TabCtl (strict)"() -> ("Value"=w1297:T1)  [unwired: 2 in, 2 out]
            n632 = Bundle By Name(cluster=w1304, "QueueAction"=DeviceQueue_Action."Spectrometer_Preview", "TabControl"=w1297) -> (w1303:T11)
            n633 = Enqueue Element(queue=w1301, element=w1303, error in (no error)=w1300) -> (queue out=w1299:refnum<queue>, error out=w1298:errorcluster)  [unwired: 1 in, 1 out]
          }
        }
      }
      event "Measure:\nRecord_Darkspec", "SpectralStability:\nRecord_Darkspec": Value Change {
        w1335 = T11 {"QueueAction"=enum."TimeOut", "Numeric 1"=0.0, "Numeric 2"=0.0, "Boolean 1"=FALSE, "Boolean 2"=FALSE, "Spin Program"=[], "Spin Prg v07"=[], "Time Stamp"=timestamp(0 s since 1904-01-01), "TabControl"=enum."Measure"}  # Device Queue
        n634 = event-data() -> ()  [unwired: 1 in, 6 out]
        n635 = property on="Shutter Toggle" class="Bool (strict)"("Value"=FALSE ("Shutter Toggle")) -> ()  [unwired: 2 in, 2 out]
        n636 = property on="Frames for Ref/Dark" class="DigNum (strict)"() -> ("Value"=w1320:dbl)  [unwired: 2 in, 2 out]
        n637 = property on="Measure_FramesSpectrometer" class="DigNum (strict)"() -> ("Value"=w1314:dbl)  [unwired: 2 in, 2 out]
        n638 = Bundle By Name(cluster=w1335, "QueueAction"=DeviceQueue_Action."Arduino_Shutter_Close") -> (w1310:T11)
        n639 = Bundle By Name(cluster=w1310, "QueueAction"=DeviceQueue_Action."Spectrometer_SetTriggerMode", "Numeric 1"=0.0) -> (w1309:T11)
        n640 = Bundle By Name(cluster=w1309, "QueueAction"=DeviceQueue_Action."Wait", "Numeric 1"=0.5) -> (w1334:T11)
        n641 = Bundle By Name(cluster=w1334, "QueueAction"=DeviceQueue_Action."Spectrometer_SetFrames", "Numeric 1"=w1320) -> (w1318:T11)
        n642 = Enqueue Element(queue=w1330, element=w1310, error in (no error)=w1329) -> (queue out=w1328:refnum<queue>, error out=w1306:errorcluster)  [unwired: 1 in, 1 out]
        n643 = Bundle By Name(cluster=w1318, "QueueAction"=DeviceQueue_Action."Spectrometer_SetDarkspec") -> (w1316:T11)
        n644 = Enqueue Element(queue=w1328, element=w1309, error in (no error)=w1306) -> (queue out=w1311:refnum<queue>, error out=w1305:errorcluster)  [unwired: 1 in, 1 out]
        n645 = Bundle By Name(cluster=w1316, "QueueAction"=DeviceQueue_Action."Spectrometer_SetFrames", "Numeric 1"=w1314) -> (w1317:T11)
        n646 = Enqueue Element(queue=w1311, element=w1334, error in (no error)=w1305) -> (queue out=w1326:refnum<queue>, error out=w1327:errorcluster)  [unwired: 1 in, 1 out]
        n647 = Enqueue Element(queue=w1326, element=w1318, error in (no error)=w1327) -> (queue out=w1324:refnum<queue>, error out=w1323:errorcluster)  [unwired: 1 in, 1 out]
        n648 = Enqueue Element(queue=w1324, element=w1316, error in (no error)=w1323) -> (queue out=w1322:refnum<queue>, error out=w1321:errorcluster)  [unwired: 1 in, 1 out]
        n649 = Enqueue Element(queue=w1322, element=w1317, error in (no error)=w1321) -> (queue out=w1312:refnum<queue>, error out=w1313:errorcluster)  [unwired: 1 in, 1 out]
      }
      event "StartMeasurement_Button": Value Change {
        w1347 = T8 {"QueueAction"=enum."TimeOut", "Data"=[], "Data_Raw"=[], "Data_Dark"=[], "Data_Ref"=[], "Device Information"=[], "Numeric Control"=0.0, "Boolean"=FALSE, "Wavelength"=[], "Time"=[], "Time Stamp"=timestamp(0 s since 1904-01-01), "Numeric Control 2"=0.0, "TabControl"=enum."Measure", "Numeric Control 3"=0.0}  # DataQueue
        w1354 = T11 {"QueueAction"=enum."TimeOut", "Numeric 1"=0.0, "Numeric 2"=0.0, "Boolean 1"=FALSE, "Boolean 2"=FALSE, "Spin Program"=[], "Spin Prg v07"=[], "Time Stamp"=timestamp(0 s since 1904-01-01), "TabControl"=enum."Measure"}  # Device Queue
        n650 = event-data() -> ()  [unwired: 1 in, 6 out]
        n651 = property on="Measure_Preview" class="Bool (strict)"("Value"=FALSE ("Preview")) -> ()  [unwired: 2 in, 2 out]
        n652 = case shown="\"Normal\", Default" "Tab Control SpinType" {
          tunnel: [DeviceQueue_Action."Measure_InSituAdvanced" ("QueueAction") DeviceQueue_Action."Measure_InSituAdvanced_Short" ("QueueAction")] -> w1340
          tunnel: [DataQueue_Action."Measure_InSituSpinCoating" ("QueueAction") DataQueue_Action."Measure_InSituSpinCoating_Short" ("QueueAction")] -> w1339
          frame "Normal", Default {
            n653 = property on="Motor_ShortStop" class="Bool (strict)"("Value"=FALSE ("Motor_ShortStop")) -> ()  [unwired: 2 in, 2 out]
          }
          frame "Short" {
            n654 = property on="Motor_ShortStop" class="Bool (strict)"("Value"=TRUE ("Motor_ShortStop")) -> ()  [unwired: 2 in, 2 out]
          }
        }
        n655 = Get Date/Time In Seconds() -> (seconds since 1Jan1904=w1342:timestamp)
        n656 = Bundle By Name(cluster=w1354, "QueueAction"=w1340, "Time Stamp"=w1342) -> (w1353:T11)
        n657 = Enqueue Element(queue=w1352, element=w1353, error in (no error)=w1350) -> (queue out=w1351:refnum<queue>, error out=w1343:errorcluster)  [unwired: 1 in, 1 out]
        n658 = property on="Reference\nValue" class="DigNum (strict)"("Value"=1.0 ("Reference\nValue")) -> ()  [unwired: 2 in, 2 out]
        n659 = Bundle By Name(cluster=w1347, "QueueAction"=w1339, "Time Stamp"=w1342) -> (w1348:T8)
        n660 = Enqueue Element(queue=w1346, element=w1348, error in (no error)=w1343) -> (queue out=w1345:refnum<queue>, error out=w1344:errorcluster)  [unwired: 1 in, 1 out]
      }
      event "StartSpin_Button": Value Change {
        w1373 = T11 {"QueueAction"=enum."TimeOut", "Numeric 1"=0.0, "Numeric 2"=0.0, "Boolean 1"=FALSE, "Boolean 2"=FALSE, "Spin Program"=[], "Spin Prg v07"=[], "Time Stamp"=timestamp(0 s since 1904-01-01), "TabControl"=enum."Measure"}  # Device Queue
        n661 = event-data() -> ()  [unwired: 1 in, 6 out]
        n662 = Bundle By Name(cluster=w1373, "QueueAction"=DeviceQueue_Action."Arduino_StartProgram", "Numeric 1"=1.0) -> (w1364:T11)
        n663 = Bundle By Name(cluster=w1364, "QueueAction"=DeviceQueue_Action."Arduino_Shutter_Close") -> (w1362:T11)
        n664 = Enqueue Element(queue=w1372, element=w1364, error in (no error)=w1370) -> (queue out=w1367:refnum<queue>, error out=w1368:errorcluster)  [unwired: 1 in, 1 out]
        n665 = Enqueue Element(queue=w1367, element=w1362, error in (no error)=w1368) -> (queue out=w1366:refnum<queue>, error out=w1365:errorcluster)  [unwired: 1 in, 1 out]
      }
      event "ESC_Milliseconds": Value Change {
        w1382 = T11 {"QueueAction"=enum."TimeOut", "Numeric 1"=0.0, "Numeric 2"=0.0, "Boolean 1"=FALSE, "Boolean 2"=FALSE, "Spin Program"=[], "Spin Prg v07"=[], "Time Stamp"=timestamp(0 s since 1904-01-01), "TabControl"=enum."Measure"}  # Device Queue
        n666 = event-data() -> ()  [unwired: 1 in, 6 out]
        n667 = Bundle By Name(cluster=w1382, "QueueAction"=DeviceQueue_Action."Arduino_SetMillis", "Numeric 1"="ESC_Milliseconds") -> (w1378:T11)
        n668 = Enqueue Element(queue=w1381, element=w1378, error in (no error)=w1379) -> (queue out=w1377:refnum<queue>, error out=w1376:errorcluster)  [unwired: 1 in, 1 out]
      }
      event "ESC_Speed": Value Change {
        w1391 = T11 {"QueueAction"=enum."TimeOut", "Numeric 1"=0.0, "Numeric 2"=0.0, "Boolean 1"=FALSE, "Boolean 2"=FALSE, "Spin Program"=[], "Spin Prg v07"=[], "Time Stamp"=timestamp(0 s since 1904-01-01), "TabControl"=enum."Measure"}  # Device Queue
        n669 = event-data() -> ()  [unwired: 1 in, 6 out]
        n670 = Bundle By Name(cluster=w1391, "QueueAction"=DeviceQueue_Action."Arduino_SetSpeed", "Numeric 1"="ESC_Speed") -> (w1387:T11)
        n671 = Enqueue Element(queue=w1390, element=w1387, error in (no error)=w1388) -> (queue out=w1386:refnum<queue>, error out=w1385:errorcluster)  [unwired: 1 in, 1 out]
      }
      event "ESC DEBUG": Value Change {
        n672 = event-data() -> ()  [unwired: 1 in, 6 out]
        n673 = Select(t=u8 0, s="ESC DEBUG", f=u8 2) -> (s? t:f=w1392:u8)
        n674 = property on="ESC_Milliseconds" class="DigNum (strict)"("DisabledEnum"=w1392) -> ()  [unwired: 2 in, 2 out]
        n675 = property on="ESC_Speed" class="DigNum (strict)"("DisabledEnum"=w1392) -> ()  [unwired: 2 in, 2 out]
      }
      event "Measure_FramesSpectrometer", "SpectralStability_FramesSpectrometer": Value Change {
        w1406 = T11 {"QueueAction"=enum."TimeOut", "Numeric 1"=0.0, "Numeric 2"=0.0, "Boolean 1"=FALSE, "Boolean 2"=FALSE, "Spin Program"=[], "Spin Prg v07"=[], "Time Stamp"=timestamp(0 s since 1904-01-01), "TabControl"=enum."Measure"}  # Device Queue
        n676 = event-data() -> ("NewVal"=w1400:dbl)  [unwired: 1 in, 5 out]
        n677 = property on="Tab Control" class="TabCtl (strict)"() -> ("Value"=w1399:T1)  [unwired: 2 in, 2 out]
        n678 = Bundle By Name(cluster=w1406, "QueueAction"=DeviceQueue_Action."Spectrometer_SetFrames", "Numeric 1"=w1400, "TabControl"=w1399) -> (w1407:T11)
        n679 = Enqueue Element(queue=w1404, element=w1407) -> (queue out=w1401:refnum<queue>)  [unwired: 2 in, 2 out]
      }
      event "Measure_MeasureSpectrum", "SpectralStability_MeasureSpectrum": Value Change {
        w1419 = T8 {"QueueAction"=enum."TimeOut", "Data"=[], "Data_Raw"=[], "Data_Dark"=[], "Data_Ref"=[], "Device Information"=[], "Numeric Control"=0.0, "Boolean"=FALSE, "Wavelength"=[], "Time"=[], "Time Stamp"=timestamp(0 s since 1904-01-01), "Numeric Control 2"=0.0, "TabControl"=enum."Measure", "Numeric Control 3"=0.0}  # DataQueue
        n680 = event-data() -> ()  [unwired: 1 in, 6 out]
        n681 = property on="Tab Control" class="TabCtl (strict)"() -> ("Value"=w1411:T1)  [unwired: 2 in, 2 out]
        n682 = case shown="\"Measure\"" w1411 {
          tunnel: w1413 -> [w1431 w1434]
          tunnel: [w1431 w1433] -> w1412
          tunnel: [w1430 w1432] -> w1410
          frame Default {
            w1430 = T11 {"QueueAction"=enum."TimeOut", "Numeric 1"=0.0, "Numeric 2"=0.0, "Boolean 1"=FALSE, "Boolean 2"=FALSE, "Spin Program"=[], "Spin Prg v07"=[], "Time Stamp"=timestamp(0 s since 1904-01-01), "TabControl"=enum."Measure"}  # Device Queue
          }
          frame "Measure" {
            w1437 = T11 {"QueueAction"=enum."TimeOut", "Numeric 1"=0.0, "Numeric 2"=0.0, "Boolean 1"=FALSE, "Boolean 2"=FALSE, "Spin Program"=[], "Spin Prg v07"=[], "Time Stamp"=timestamp(0 s since 1904-01-01), "TabControl"=enum."Measure"}  # Device Queue
            (unwired) T11 {"QueueAction"=enum."TimeOut", "Numeric 1"=0.0, "Numeric 2"=0.0, "Boolean 1"=FALSE, "Boolean 2"=FALSE, "Spin Program"=[], "Spin Prg v07"=[], "Time Stamp"=timestamp(0 s since 1904-01-01), "TabControl"=enum."Measure"}  # Device Queue
            n683 = Bundle By Name(cluster=w1437, "QueueAction"=DeviceQueue_Action."Spectrometer_SetFrames", "Numeric 1"="Frames for Ref/Dark") -> (w1432:T11)
            n684 = Enqueue Element(queue=w1434, element=w1432) -> (queue out=w1433:refnum<queue>)  [unwired: 2 in, 2 out]
          }
        }
        n685 = Get Date/Time In Seconds() -> (seconds since 1Jan1904=w1414:timestamp)
        n686 = Bundle By Name(cluster=w1410, "QueueAction"=DeviceQueue_Action."Measure_Spectrum", "Time Stamp"=w1414, "TabControl"=w1411) -> (w1422:T11)
        n687 = Enqueue Element(queue=w1412, element=w1422) -> (queue out=w1409:refnum<queue>)  [unwired: 2 in, 2 out]
        n688 = case shown="Default" w1411 {
          tunnel: w1410 -> [_ w1428]
          tunnel: w1409 -> [w1423 w1427]
          tunnel: [w1423 w1426] -> w1408
          frame Default {
          }
          frame "Measure" {
            n689 = property on="Measure_FramesSpectrometer" class="DigNum (strict)"() -> ("Value"=w1425:dbl)  [unwired: 2 in, 2 out]
            n690 = Bundle By Name(cluster=w1428, "QueueAction"=DeviceQueue_Action."Spectrometer_SetFrames", "Numeric 1"=w1425) -> (w1424:T11)
            n691 = Enqueue Element(queue=w1427, element=w1424) -> (queue out=w1426:refnum<queue>)  [unwired: 2 in, 2 out]
          }
        }
        n692 = Bundle By Name(cluster=w1419, "QueueAction"=DataQueue_Action."Measure_Spectrum", "TabControl"=w1411) -> (w1416:T8)
        n693 = Enqueue Element(queue=w1417, element=w1416) -> (queue out=w1415:refnum<queue>)  [unwired: 2 in, 2 out]
      }
      event "SpectralStability_Record": Value Change {
        w1446 = T8 {"QueueAction"=enum."TimeOut", "Data"=[], "Data_Raw"=[], "Data_Dark"=[], "Data_Ref"=[], "Device Information"=[], "Numeric Control"=0.0, "Boolean"=FALSE, "Wavelength"=[], "Time"=[], "Time Stamp"=timestamp(0 s since 1904-01-01), "Numeric Control 2"=0.0, "TabControl"=enum."Measure", "Numeric Control 3"=0.0}  # DataQueue
        w1451 = T11 {"QueueAction"=enum."TimeOut", "Numeric 1"=0.0, "Numeric 2"=0.0, "Boolean 1"=FALSE, "Boolean 2"=FALSE, "Spin Program"=[], "Spin Prg v07"=[], "Time Stamp"=timestamp(0 s since 1904-01-01), "TabControl"=enum."Measure"}  # Device Queue
        n694 = event-data() -> ()  [unwired: 1 in, 6 out]
        n695 = property on="Duration/\nTimes" class="Bool (strict)"() -> ("Value"=w1439:bool)  [unwired: 2 in, 2 out]
        n696 = case shown="False" w1439 {
          tunnel: ["SpectralStability_\nMeasurementNumber" w1454] -> w1438
          frame False {
            # "Number"
          }
          frame True {
            # "Duration"
            n697 = property on="SpectralStability_\nPeriodicTime" class="DigNum (strict)"() -> ("Value"=w1456:dbl[unit])  [unwired: 2 in, 2 out]
            n698 = Divide(x="SpectralStability_Duration", y=w1456) -> (x/y=w1457:dbl)
            n699 = Round Toward +Infinity(x=w1457) -> (ceil(x): smallest int >= x=w1455:dbl)
            n700 = Increment(x=w1455) -> (x+1=w1454:dbl)
          }
        }
        n701 = Get Date/Time In Seconds() -> (seconds since 1Jan1904=w1440:timestamp)
        n702 = property on="Tab Control" class="TabCtl (strict)"() -> ("Value"=w1441:T1)  [unwired: 2 in, 2 out]
        n703 = Bundle By Name(cluster=w1451, "QueueAction"=DeviceQueue_Action."Measure_SpectralStability", "Time Stamp"=w1440, "TabControl"=w1441, "Numeric 1"=w1438) -> (w1452:T11)
        n704 = property on="SS_StepsLeft" class="DigNum (strict)"("Value"=w1438) -> ()  [unwired: 2 in, 2 out]
        n705 = Enqueue Element(queue=w1449, element=w1452) -> (queue out=w1447:refnum<queue>)  [unwired: 2 in, 2 out]
        n706 = Bundle By Name(cluster=w1446, "QueueAction"=DataQueue_Action."Measure_SpectralStability", "TabControl"=w1441, "Time Stamp"=w1440, "Numeric Control"=w1438) -> (w1443:T8)
        n707 = Enqueue Element(queue=w1444, element=w1443) -> (queue out=w1442:refnum<queue>)  [unwired: 2 in, 2 out]
      }
      event "Automatically \nadjust count": Value Change {
        n708 = event-data() -> ("NewVal"=w1465:bool)  [unwired: 1 in, 5 out]
        n709 = Select(t=u8 2, s=w1465, f=u8 0) -> (s? t:f=w1459:u8)
        n710 = property on="Spectra Count" class="DigNum (strict)"("DisabledEnum"=w1459) -> ()  [unwired: 2 in, 2 out]
      }
      event "Duration/Times": Value Change {
        n711 = event-data() -> ("NewVal"=w1471:bool)  [unwired: 1 in, 5 out]
        n712 = case shown="False" w1471 {
          tunnel: [FALSE TRUE] -> w1470
          tunnel: [TRUE FALSE] -> w1469
          frame False {
          }
          frame True {
          }
        }
        n713 = property on="SpectralStability_Duration" class="DigNum (strict)"("Visible"=w1470) -> ()  [unwired: 2 in, 2 out]
        n714 = property on="SpectralStability_\nMeasurementNumber" class="DigNum (strict)"("Visible"=w1469) -> ()  [unwired: 2 in, 2 out]
      }
      event "Tab Control": Value Change {
        w1476 = FALSE ("SpectralStability_Preview")
        n715 = event-data() -> ("NewVal"=w1479:T1)  [unwired: 1 in]
        n716 = case shown="\"Spectral Stability\"" w1479 {
          tunnel: w1481 -> [w1484 w1497 w1512]
          tunnel: [w1484 w1486 w1503] -> w1478
          tunnel: w1480 -> [w1483 w1496 w1511]
          tunnel: w1479 -> [_ w1495 w1510]
          tunnel: [w1483 w1485 w1502] -> w1477
          frame Default {
          }
          frame "Measure" {
            w1499 = T11 {"QueueAction"=enum."TimeOut", "Numeric 1"=0.0, "Numeric 2"=0.0, "Boolean 1"=FALSE, "Boolean 2"=FALSE, "Spin Program"=[], "Spin Prg v07"=[], "Time Stamp"=timestamp(0 s since 1904-01-01), "TabControl"=enum."Measure"}  # Device Queue
            n717 = property on="Measure_IntegrationTime" class="DigNum (strict)"() -> ("Value"=w1494:dbl[unit])  [unwired: 2 in, 2 out]
            n718 = node(w1494) -> (w1493:dbl)
            n719 = Bundle By Name(cluster=w1499, "QueueAction"=DeviceQueue_Action."Spectrometer_SetIntegrationTime", "Numeric 1"=w1493, "TabControl"=w1495) -> (w1490:T11)
            n720 = property on="Measure_FramesSpectrometer" class="DigNum (strict)"() -> ("Value"=w1488:dbl)  [unwired: 2 in, 2 out]
            n721 = Enqueue Element(queue=w1497, element=w1490, error in (no error)=w1496) -> (queue out=w1492:refnum<queue>, error out=w1491:errorcluster)  [unwired: 1 in, 1 out]
            n722 = Bundle By Name(cluster=w1490, "QueueAction"=DeviceQueue_Action."Spectrometer_SetFrames", "Numeric 1"=w1488) -> (w1487:T11)
            n723 = Enqueue Element(queue=w1492, element=w1487, error in (no error)=w1491) -> (queue out=w1486:refnum<queue>, error out=w1485:errorcluster)  [unwired: 1 in, 1 out]
          }
          frame "Spectral Stability" {
            w1514 = T11 {"QueueAction"=enum."TimeOut", "Numeric 1"=0.0, "Numeric 2"=0.0, "Boolean 1"=FALSE, "Boolean 2"=FALSE, "Spin Program"=[], "Spin Prg v07"=[], "Time Stamp"=timestamp(0 s since 1904-01-01), "TabControl"=enum."Measure"}  # Device Queue
            n724 = property on="SpectralStability_IntegrationTime" class="DigNum (strict)"() -> ("Value"=w1501:dbl[unit])  [unwired: 2 in, 2 out]
            n725 = node(w1501) -> (w1509:dbl)
            n726 = property on="SpectralStability_FramesSpectrometer" class="DigNum (strict)"() -> ("Value"=w1500:dbl)  [unwired: 2 in, 2 out]
            n727 = Bundle By Name(cluster=w1514, "QueueAction"=DeviceQueue_Action."Spectrometer_SetIntegrationTime", "Numeric 1"=w1509, "TabControl"=w1510) -> (w1506:T11)
            n728 = Enqueue Element(queue=w1512, element=w1506, error in (no error)=w1511) -> (queue out=w1508:refnum<queue>, error out=w1507:errorcluster)  [unwired: 1 in, 1 out]
            n729 = Bundle By Name(cluster=w1506, "QueueAction"=DeviceQueue_Action."Spectrometer_SetFrames", "Numeric 1"=w1500) -> (w1504:T11)
            n730 = Enqueue Element(queue=w1508, element=w1504, error in (no error)=w1507) -> (queue out=w1503:refnum<queue>, error out=w1502:errorcluster)  [unwired: 1 in, 1 out]
          }
        }
        n731 = property on="SpectralStability_Preview" class="Bool (strict)"("Value"=w1476) -> ()  [unwired: 2 in, 2 out]
        n732 = property on="Measure_Preview" class="Bool (strict)"("Value"=w1476) -> ()  [unwired: 2 in, 2 out]
      }
      event "Trim\nSpec", "Wl \nUp", "Wl \nLow": Value Change {
        w1524 = T8 {"QueueAction"=enum."TimeOut", "Data"=[], "Data_Raw"=[], "Data_Dark"=[], "Data_Ref"=[], "Device Information"=[], "Numeric Control"=0.0, "Boolean"=FALSE, "Wavelength"=[], "Time"=[], "Time Stamp"=timestamp(0 s since 1904-01-01), "Numeric Control 2"=0.0, "TabControl"=enum."Measure", "Numeric Control 3"=0.0}  # DataQueue
        n733 = event-data() -> ()  [unwired: 1 in, 6 out]
        n734 = node("Wl \nLow") -> (w1518:dbl)
        n735 = node("Wl \nUp") -> (w1517:dbl)
        n736 = Bundle By Name(cluster=w1524, "QueueAction"=DataQueue_Action."Change_TrimSettings", "Numeric Control"=w1518, "Numeric Control 2"=w1517, "Boolean"="Trim\nSpec") -> (w1525:T8)
        n737 = Enqueue Element(queue=w1523, element=w1525) -> (queue out=w1522:refnum<queue>)  [unwired: 2 in, 2 out]
      }
      event "Motor_ShortStop": Value Change {
        w1533 = T11 {"QueueAction"=enum."TimeOut", "Numeric 1"=0.0, "Numeric 2"=0.0, "Boolean 1"=FALSE, "Boolean 2"=FALSE, "Spin Program"=[], "Spin Prg v07"=[], "Time Stamp"=timestamp(0 s since 1904-01-01), "TabControl"=enum."Measure"}  # Device Queue
        n738 = event-data() -> ()  [unwired: 1 in, 6 out]
        n739 = Bundle By Name(cluster=w1533, "QueueAction"=DeviceQueue_Action."Arduino_ShortStop") -> (w1532:T11)
        n740 = Enqueue Element At Opposite End(queue=w1531, element=w1532, error in (no error)=w1528) -> (queue out=w1530:refnum<queue>, error out=w1527:errorcluster)  [unwired: 1 in, 1 out]
      }
    }
  }
  n741 = while {
    shift-right: [w1539] -> _
    shift-left: w1 -> [w1543]
    shift-right: [w1540] -> w10
    shift-left: w12 -> [w1542]
    shift-right: [w1537] -> w9
    shift-left: w8 -> [w1538]
    shift-right: [w1535] -> _
    shift-left: w11 -> [w1536]
    stop <- w1541 stop-if-true
    # "Consumer Devices"
    n742 = case shown="No Error" w1543 {
      selector: w1543 -> [w1556 w2450]
      tunnel: w1542 -> [w1557 w2451]
      tunnel: [w1553 _] -> w1541
      tunnel: [w1552 w2451] -> w1540
      tunnel: [w1550 w2447] -> w1539
      tunnel: w1538 -> [w1548 w2445]
      tunnel: [w1549 w2445] -> w1537
      tunnel: w1536 -> [w1547 w2446]
      tunnel: [w1546 w2446] -> w1535
      frame No Error {
        n743 = Dequeue Element(queue=w1557, timeout in ms (-1)=10, error in (no error)=w1556) -> (queue out=w1555:refnum<queue>, element=w1545:T11, error out=w1551:errorcluster)  [unwired: 1 out]
        n744 = Unbundle By Name(w1545) -> ("QueueAction"=w1554:T12)
        n745 = case shown="\"Spectrometer_Measure\"" w1554 {
          tunnel: w1555 -> [w1562 w1583 w1624 w1647 w1658 w1713 w1732 w1757 w1768 w1791 w1798 w1817 w1882 w1939 w1970 w1989 w2004 w2014 w2026 w2027 w2049 w2073 w2080 w2087 w2099 w2105 w2111 w2123 w2130 w2137 w2146 w2192 w2287 w2390 w2406 w2416]
          tunnel: [_ _ w1626 _ _ _ _ _ _ _ _ _ _ _ _ _ _ _ _ _ _ _ _ _ _ _ _ _ _ _ _ _ _ _ _ _] -> w1553
          tunnel: [w1562 w1583 w1609 w1634 w1654 w1713 w1732 w1757 w1769 w1791 w1798 w1817 w1882 w1939 w1970 w1989 w2004 w2014 w2026 w2027 w2049 w2073 w2080 w2087 w2099 w2105 w2111 w2123 w2130 w2137 w2146 w2154 w2203 w2350 w2397 w2419] -> w1552
          tunnel: w1551 -> [w1561 w1582 w1608 w1646 w1669 w1714 w1731 w1756 w1764 w1794 w1802 w1814 w1870 w1949 w1968 w1979 w1995 w2011 w2022 w2034 w2052 w2067 w2077 w2085 w2094 w2102 w2108 w2114 w2126 w2133 w2139 w2148 w2248 w2354 w2405 w2415]
          tunnel: [w1561 w1582 w1607 w1628 w1657 w1708 w1730 w1755 w1762 w1792 w1799 w1805 w1824 w1943 w1967 w1974 w1991 w2009 w2016 w2037 w2051 w2064 w2076 w2083 w2093 w2101 w2107 w2113 w2125 w2132 w2138 w2155 w2202 w2343 w2396 w2420] -> w1550
          tunnel: [w1559 w1580 w1606 w1651 w1655 w1710 w1723 w1737 w1773 w1790 w1797 w1808 w1876 w1951 w1971 w1983 w1998 w2005 w2018 w2039 w2050 w2072 w2082 w2091 w2097 w2106 w2112 w2122 w2129 w2136 w2141 w2163 w2260 w2365 w2404 w2436] -> w1549
          tunnel: w1548 -> [w1559 w1580 w1606 w1651 w1656 w1710 w1722 w1746 w1774 w1790 w1797 w1809 w1877 w1951 w1971 w1986 w2001 w2005 w2020 w2039 w2050 w2072 w2082 w2091 w2097 w2106 w2112 w2122 w2129 w2136 w2142 w2163 w2260 w2365 w2404 w2436]
          tunnel: w1547 -> [w1560 w1581 w1605 w1650 w1666 w1712 w1729 w1754 w1767 w1789 w1801 w1810 w1861 w1942 w1964 w1982 w1997 w2008 w2015 w2036 w2045 w2066 w2081 w2090 w2096 w2104 w2110 w2121 w2128 w2135 w2140 w2195 w2290 w2393 w2403 w2435]
          tunnel: [w1560 w1581 w1605 w1650 w1660 w1711 w1729 w1754 w1766 w1787 w1796 w1810 w1861 w1940 w1965 w1981 w1996 w2006 w2015 w2038 w2043 w2063 w2081 w2090 w2096 w2104 w2110 w2121 w2128 w2135 w2140 w2195 w2290 w2393 w2403 w2435] -> w1546
          tunnel: w1545 -> [_ w1576 _ _ w1653 _ w1721 w1748 w1760 _ _ w1816 w1881 w1946 w1972 _ _ w2012 _ _ _ w2071 w2075 w2089 w2098 _ _ w2119 _ _ _ _ w2230 _ w2394 w2410]
          frame "TimeOut", Default {
            n746 = property on="Action" class="Str"("Value"="TimeOut" ("Action")) -> ()  [unwired: 2 in, 2 out]
          }
          frame "Wait" {
            n747 = flat-sequence {
              tunnel: [w1594] -> w1577
              tunnel: w1576 -> [w1594]
              tunnel: [w1593] -> w1574
              frame #0 {
                n748 = Tick Count (ms)() -> (millisecond timer value=w1593:u32)
              }
            }
            n749 = Unbundle By Name(w1577) -> ("Numeric 1"=w1568:dbl)
            n750 = property on="SS:PeriodicTime" class="DigNum (strict)"() -> ("Value"=w1570:dbl[unit])  [unwired: 2 in, 2 out]
            n751 = Multiply(x=w1568, y=1000.0) -> (x*y=w1572:dbl)
            n752 = node(w1568) -> (w1569:dbl[unit])
            n753 = property on="SS_StepsLeft" class="DigNum (strict)"() -> ("Value"=w1567:dbl)  [unwired: 2 in, 2 out]
            n754 = Round Toward -Infinity(1:w1568) -> (0:w1571:dbl)
            n755 = Subtract(x=w1570, y=w1569) -> (x-y=w1564:dbl[unit])
            n756 = Decrement(x=w1567) -> (x-1=w1566:dbl)
            n757 = Multiply(x=w1566, y=w1570) -> (x*y=w1565:dbl[unit])
            n758 = Add(x=w1565, y=w1564) -> (x+y=w1563:dbl[unit])
            n759 = for {
              N: w1571 -> [_]
              tunnel: 1000.0 ("y") -> [w1595]
              tunnel: [w1603] -> w1575
              tunnel: w1563 -> [w1600]
              i -> [w1598]
              stop <- w1603 stop-if-true
              n760 = Increment(x=w1598) -> (x+1=w1596:i32)
              n761 = Multiply(x=w1595, y=w1596) -> (x*y=w1597:dbl)
              n762 = node(w1597) -> (w1599:dbl[unit])
              n763 = property on="Stop Button" class="Bool (strict)"() -> ("Value"=w1603:bool)  [unwired: 2 in, 2 out]
              n764 = Wait (ms)(milliseconds to wait=w1595) -> (millisecond timer value=w1601:u32)
              n765 = Subtract(x=w1600, y=w1599) -> (x-y=w1602:dbl[unit])
              n766 = flat-sequence {
                tunnel: w1602 -> [w1604]
                tunnel: w1601 -> [_]
                frame #0 {
                  n767 = property on="SS_TimePrediction" class="DigNum (strict)"("Value"=w1604) -> ()  [unwired: 2 in, 2 out]
                }
              }
            }
            n768 = property on="Action" class="Str"("Value"="Wait" ("Action")) -> ()  [unwired: 2 in, 2 out]
            n769 = case shown="False" w1575 {
              tunnel: w1574 -> [w1589 _]
              tunnel: w1572 -> [w1584 _]
              frame False {
                n770 = flat-sequence {
                  tunnel: [w1592] -> w1590
                  frame #0 {
                    n771 = Tick Count (ms)() -> (millisecond timer value=w1592:u32)
                  }
                }
                n772 = Subtract(x=w1590, y=w1589) -> (x-y=w1588:u32)
                n773 = To Double Precision Float(number=w1588) -> (double precision float=w1585:dbl)
                n774 = Subtract(x=w1584, y=w1585) -> (x-y=w1586:dbl)
                n775 = Greater Than 0?(x=w1586) -> (x > 0?=w1587:bool)
                n776 = case shown="True" w1587 {
                  tunnel: w1586 -> [_ w1591]
                  frame False {
                  }
                  frame True {
                    n777 = Wait (ms)(milliseconds to wait=w1591) -> ()  [unwired: 1 out]
                  }
                }
              }
              frame True {
                # "If Aborted, do nothing"
              }
            }
          }
          frame "Close_Program" {
            w1625 = T11 {"QueueAction"=enum."TimeOut", "Numeric 1"=0.0, "Numeric 2"=0.0, "Boolean 1"=FALSE, "Boolean 2"=FALSE, "Spin Program"=[], "Spin Prg v07"=[], "Time Stamp"=timestamp(0 s since 1904-01-01), "TabControl"=enum."Measure"}  # Device Queue
            n778 = Bundle By Name(cluster=w1625, "QueueAction"=DeviceQueue_Action."Spectrometer_Close") -> (w1620:T11)
            n779 = Bundle By Name(cluster=w1620, "QueueAction"=DeviceQueue_Action."Laser_Close") -> (w1618:T11)
            n780 = Bundle By Name(cluster=w1618, "QueueAction"=DeviceQueue_Action."Arduino_Close") -> (w1612:T11)
            n781 = Enqueue Element(queue=w1624, element=w1620, error in (no error)=w1608) -> (queue out=w1622:refnum<queue>, error out=w1617:errorcluster)  [unwired: 1 in, 1 out]
            n782 = Bundle By Name(cluster=w1612, "QueueAction"=DeviceQueue_Action."Close_Program") -> (w1610:T11)
            n783 = Enqueue Element(queue=w1622, element=w1618, error in (no error)=w1617) -> (queue out=w1616:refnum<queue>, error out=w1615:errorcluster)  [unwired: 1 in, 1 out]
            n784 = Enqueue Element(queue=w1616, element=w1612, error in (no error)=w1615) -> (queue out=w1614:refnum<queue>, error out=w1613:errorcluster)  [unwired: 1 in, 1 out]
            n785 = Enqueue Element(queue=w1614, element=w1610, error in (no error)=w1613) -> (queue out=w1609:refnum<queue>, error out=w1607:errorcluster)  [unwired: 1 in, 1 out]
            n786 = First Call?() -> (First Call?: T/F=w1627:bool)
            n787 = Not(x=w1627) -> (.not. x?=w1626:bool)
          }
          frame "Abort" {
            w1649 = T11 {"QueueAction"=enum."TimeOut", "Numeric 1"=0.0, "Numeric 2"=0.0, "Boolean 1"=FALSE, "Boolean 2"=FALSE, "Spin Program"=[], "Spin Prg v07"=[], "Time Stamp"=timestamp(0 s since 1904-01-01), "TabControl"=enum."Measure"}  # Device Queue
            n788 = Flush Queue(queue=w1647, error in (no error)=w1646) -> (queue out=w1645:refnum<queue>, error out=w1644:errorcluster)  [unwired: 1 out]
            n789 = Bundle By Name(cluster=w1649, "QueueAction"=DeviceQueue_Action."Spectrometer_StopMeasurement") -> (w1641:T11)
            n790 = Bundle By Name(cluster=w1641, "QueueAction"=DeviceQueue_Action."Arduino_StopSpin") -> (w1637:T11)
            n791 = Enqueue Element(queue=w1645, element=w1641, error in (no error)=w1644) -> (queue out=w1643:refnum<queue>, error out=w1642:errorcluster)  [unwired: 1 in, 1 out]
            n792 = Bundle By Name(cluster=w1637, "QueueAction"=DeviceQueue_Action."Measure_Stop") -> (w1632:T11)
            n793 = Enqueue Element(queue=w1643, element=w1637, error in (no error)=w1642) -> (queue out=w1639:refnum<queue>, error out=w1638:errorcluster)  [unwired: 1 in, 1 out]
            n794 = Bundle By Name(cluster=w1632, "QueueAction"=DeviceQueue_Action."Spectrometer_SetTriggerMode", "Numeric 1"=0.0) -> (w1629:T11)
            n795 = Enqueue Element(queue=w1639, element=w1632, error in (no error)=w1638) -> (queue out=w1635:refnum<queue>, error out=w1633:errorcluster)  [unwired: 1 in, 1 out]
            n796 = Enqueue Element(queue=w1635, element=w1629, error in (no error)=w1633) -> (queue out=w1634:refnum<queue>, error out=w1628:errorcluster)  [unwired: 1 in, 1 out]
          }
          frame "Spectrometer_Init" {
            n797 = call-dynamic "Init.vi"("error in (no error)"=w1669, "Variant"=0, "Avantes in"=refnum<class "Avantes.lvclass"> refnum ("Avantes.lvclass")) -> ("error out"=w1668:errorcluster, "Avantes out"=w1667:refnum<class "Avantes.lvclass">)  [unwired: 7 in]
            n798 = call-dynamic "IsInit.vi"("error in (no error)"=w1668, "Avantes in"=w1667) -> ("error out"=w1664:errorcluster, "Is Init?"=w1663:bool, "Avantes out"=w1665:refnum<class "Avantes.lvclass">)  [unwired: 7 in]
            n799 = Unbundle By Name(w1653) -> ("TabControl"=w1652:T10)
            n800 = property on="Spectromter" class="Bool (strict)"("Value"=w1663) -> ()  [unwired: 2 in, 2 out]
            n801 = property on="Init_Spectrometer" class="Bool (strict)"("Value"=w1663) -> ()  [unwired: 2 in, 2 out]
            n802 = call-dynamic "Set_ExposurePerFrame.vi"("error in (no error)"=w1664, "Exposure per Frame"=1, "Avantes in"=w1665) -> ("error out"=w1659:errorcluster, "Avantes out"=w1662:refnum<class "Avantes.lvclass">)  [unwired: 7 in]
            n803 = case shown="True" w1663 {
              tunnel: w1662 -> [_ w1692]
              tunnel: w1659 -> [w1675 w1690]
              tunnel: [refnum<class "Abstract_CCD.lvclass"> refnum ("Abstract_CCD.lvclass") w1691] -> w1661
              tunnel: w1658 -> [w1673 w1702]
              tunnel: [w1675 w1695] -> w1657
              tunnel: w1656 -> [w1674 w1687]
              tunnel: [w1674 w1685] -> w1655
              tunnel: [w1673 w1683] -> w1654
              tunnel: w1653 -> [_ w1680]
              tunnel: w1652 -> [_ w1679]
              frame False {
              }
              frame True {
                w1693 = T8 {"QueueAction"=enum."TimeOut", "Data"=[], "Data_Raw"=[], "Data_Dark"=[], "Data_Ref"=[], "Device Information"=[], "Numeric Control"=0.0, "Boolean"=FALSE, "Wavelength"=[], "Time"=[], "Time Stamp"=timestamp(0 s since 1904-01-01), "Numeric Control 2"=0.0, "TabControl"=enum."Measure", "Numeric Control 3"=0.0}  # DataQueue
                n804 = case shown="\"Spectral Stability\"" w1679 {
                  tunnel: [w1704 w1706] -> w1678
                  tunnel: [w1703 w1705] -> w1677
                  frame "Measure", Default {
                    n805 = property on="Measure_IntegrationTime" class="DigNum (strict)"() -> ("Value"=w1704:dbl[unit])  [unwired: 2 in, 2 out]
                    n806 = property on="Measure_FramesSpectrometer" class="DigNum (strict)"() -> ("Value"=w1703:dbl)  [unwired: 2 in, 2 out]
                  }
                  frame "Spectral Stability" {
                    n807 = property on="SpectralStability_FramesSpectrometer" class="DigNum (strict)"() -> ("Value"=w1705:dbl)  [unwired: 2 in, 2 out]
                    n808 = property on="SpectralStability_IntegrationTime" class="DigNum (strict)"() -> ("Value"=w1706:dbl[unit])  [unwired: 2 in, 2 out]
                  }
                }
                n809 = call-dynamic "Get_WavelengthAxis.vi"("error in (no error)"=w1690, "Avantes in"=w1692) -> ("error out"=w1689:errorcluster, "lambda"=w1684:dbl[unit][], "Avantes out"=w1691:refnum<class "Avantes.lvclass">)  [unwired: 7 in]
                n810 = Unbundle(w1689) -> ("status"=w1688:bool)  [unwired: 2 out]
                n811 = property on="Error_Spectromter" class="Bool (strict)"("Value"=w1688) -> ()  [unwired: 2 in, 2 out]
                n812 = property on="Calculate Frames_Normal" class="Bool (strict)"() -> ("Value"=w1681:bool)  [unwired: 2 in, 2 out]
                n813 = Bundle By Name(cluster=w1693, "QueueAction"=DataQueue_Action."Set_Wavelength", "Wavelength"=w1684) -> (w1694:T8)
                n814 = node(w1678) -> (w1700:dbl)
                n815 = Bundle By Name(cluster=w1680, "QueueAction"=DeviceQueue_Action."Spectrometer_SetIntegrationTime", "Numeric 1"=w1700, "Boolean 1"=w1681) -> (w1698:T11)
                n816 = Enqueue Element(queue=w1687, element=w1694) -> (queue out=w1685:refnum<queue>)  [unwired: 2 in, 2 out]
                n817 = Bundle By Name(cluster=w1698, "QueueAction"=DeviceQueue_Action."Spectrometer_SetFrames", "Numeric 1"=w1677) -> (w1697:T11)
                n818 = Enqueue Element(queue=w1702, element=w1698, error in (no error)=w1690) -> (queue out=w1699:refnum<queue>, error out=w1696:errorcluster)  [unwired: 1 in, 1 out]
                n819 = Enqueue Element(queue=w1699, element=w1697, error in (no error)=w1696) -> (queue out=w1683:refnum<queue>, error out=w1695:errorcluster)  [unwired: 1 in, 1 out]
              }
            }
            n820 = Bundle By Name(cluster=w1666, "Abstract_CCD.lvclass"=w1661) -> (w1660:T6)
          }
          frame "Spectrometer_Close" {
            n821 = property on="Spectromter" class="Bool (strict)"("Value"=FALSE ("Spectromter")) -> ()  [unwired: 2 in, 2 out]
            n822 = Unbundle By Name(w1712) -> ("Abstract_CCD.lvclass"=w1715:refnum<class "Abstract_CCD.lvclass">)
            n823 = flat-sequence {
              tunnel: [refnum<class "Abstract_CCD.lvclass"> refnum ("Abstract_CCD.lvclass")] -> w1709
              tunnel: w1708 -> [_]
              frame #0 {
              }
            }
            n824 = call-dynamic "Close.vi"("error in (no error)"=w1714, "Abstract_CCD in"=w1715) -> ("error out"=w1708:errorcluster)  [unwired: 8 in, 1 out]
            n825 = Bundle By Name(cluster=w1712, "Abstract_CCD.lvclass"=w1709) -> (w1711:T6)
          }
          frame "Spectrometer_Measure" {
            w1734 = T8 {"QueueAction"=enum."TimeOut", "Data"=[], "Data_Raw"=[], "Data_Dark"=[], "Data_Ref"=[], "Device Information"=[], "Numeric Control"=0.0, "Boolean"=FALSE, "Wavelength"=[], "Time"=[], "Time Stamp"=timestamp(0 s since 1904-01-01), "Numeric Control 2"=0.0, "TabControl"=enum."Measure", "Numeric Control 3"=0.0}  # DataQueue
            n826 = Unbundle By Name(w1729) -> ("Abstract_CCD.lvclass"=w1733:refnum<class "Abstract_CCD.lvclass">)
            n827 = Unbundle By Name(w1721) -> ("Time Stamp"=w1718:timestamp, "TabControl"=w1719:T10)
            n828 = Get Date/Time In Seconds() -> (seconds since 1Jan1904=w1717:timestamp)
            n829 = Subtract(x=w1717, y=w1718) -> (x-y=w1720:dbl)
            n830 = call-dynamic "Measure.vi"("error in (no error)"=w1731, "Abstract_CCD in"=w1733) -> ("error out"=w1730:errorcluster, "Data Raw"=w1726:T14, "Data"=w1727:T14, "Darkspec"=w1725:T14, "Time"=w1724:dbl[])  [unwired: 3 in, 2 out]
            n831 = Bundle By Name(cluster=w1734, "QueueAction"=DataQueue_Action."Spectrometer_Measure", "Data"=w1727, "Data_Raw"=w1726, "Data_Dark"=w1725, "Time"=w1724, "Time Stamp"=w1718, "Numeric Control 2"=w1720, "TabControl"=w1719) -> (w1735:T8)
            n832 = Enqueue Element(queue=w1722, element=w1735) -> (queue out=w1723:refnum<queue>)  [unwired: 2 in, 2 out]
          }
          frame "Spectrometer_MeasureAdvanced" {
            w1745 = T8 {"QueueAction"=enum."TimeOut", "Data"=[], "Data_Raw"=[], "Data_Dark"=[], "Data_Ref"=[], "Device Information"=[], "Numeric Control"=0.0, "Boolean"=FALSE, "Wavelength"=[], "Time"=[], "Time Stamp"=timestamp(0 s since 1904-01-01), "Numeric Control 2"=0.0, "TabControl"=enum."Measure", "Numeric Control 3"=0.0}  # DataQueue
            w1759 = T8 {"QueueAction"=enum."TimeOut", "Data"=[], "Data_Raw"=[], "Data_Dark"=[], "Data_Ref"=[], "Device Information"=[], "Numeric Control"=0.0, "Boolean"=FALSE, "Wavelength"=[], "Time"=[], "Time Stamp"=timestamp(0 s since 1904-01-01), "Numeric Control 2"=0.0, "TabControl"=enum."Measure", "Numeric Control 3"=0.0}  # DataQueue
            n833 = Unbundle By Name(w1754) -> ("Abstract_CCD.lvclass"=w1758:refnum<class "Abstract_CCD.lvclass">)
            n834 = Unbundle By Name(w1748) -> ("Time Stamp"=w1747:timestamp)
            n835 = call-dynamic "Measure.vi"("error in (no error)"=w1756, "Abstract_CCD in"=w1758) -> ("error out"=w1755:errorcluster, "Data Raw"=w1751:T14, "Data"=w1752:T14, "Darkspec"=w1750:T14, "Time"=w1749:dbl[])  [unwired: 3 in, 2 out]
            n836 = Bundle By Name(cluster=w1745, "QueueAction"=DataQueue_Action."Measure_SpectrumAdvanced") -> (w1743:T8)
            n837 = Bundle By Name(cluster=w1759, "QueueAction"=DataQueue_Action."Spectrometer_Measure", "Data"=w1752, "Data_Raw"=w1751, "Data_Dark"=w1750, "Time"=w1749, "Time Stamp"=w1747) -> (w1740:T8)
            n838 = Enqueue Element(queue=w1746, element=w1743) -> (queue out=w1742:refnum<queue>)  [unwired: 2 in, 2 out]
            n839 = Enqueue Element(queue=w1742, element=w1740) -> (queue out=w1741:refnum<queue>)  [unwired: 2 in, 2 out]
            n840 = Bundle By Name(cluster=w1740, "QueueAction"=DataQueue_Action."Stop_Measurement") -> (w1738:T8)
            n841 = property on="Action" class="Str"("Value"="Measure Spectra A" ("Action")) -> ()  [unwired: 2 in, 2 out]
            n842 = Enqueue Element(queue=w1741, element=w1738) -> (queue out=w1737:refnum<queue>)  [unwired: 2 in, 2 out]
          }
          frame "Spectrometer_Preview" {
            w1775 = T8 {"QueueAction"=enum."TimeOut", "Data"=[], "Data_Raw"=[], "Data_Dark"=[], "Data_Ref"=[], "Device Information"=[], "Numeric Control"=0.0, "Boolean"=FALSE, "Wavelength"=[], "Time"=[], "Time Stamp"=timestamp(0 s since 1904-01-01), "Numeric Control 2"=0.0, "TabControl"=enum."Measure", "Numeric Control 3"=0.0}  # DataQueue
            n843 = Unbundle By Name(w1767) -> ("Abstract_CCD.lvclass"=w1765:refnum<class "Abstract_CCD.lvclass">)
            n844 = Unbundle By Name(w1760) -> ("TabControl"=w1761:T10)
            n845 = call-dynamic "Measure.vi"("error in (no error)"=w1764, "Abstract_CCD in"=w1765) -> ("error out"=w1762:errorcluster, "Data Raw"=w1772:T14, "Abstract_CCD out"=w1763:refnum<class "Abstract_CCD.lvclass">)  [unwired: 3 in, 4 out]
            n846 = case shown="\"Measure\"" w1761 {
              tunnel: [FALSE ("Value") w1779 w1780] -> w1770
              tunnel: w1762 -> [_ w1778 _]
              frame Default {
              }
              frame "Measure" {
                n847 = property on="Measure_Preview" class="Bool (strict)"(error in=w1778) -> ("Value"=w1779:bool)  [unwired: 1 in, 2 out]
              }
              frame "Spectral Stability" {
                n848 = property on="SpectralStability_Preview" class="Bool (strict)"() -> ("Value"=w1780:bool)  [unwired: 2 in, 2 out]
              }
            }
            n849 = case shown="True" w1770 {
              tunnel: [w1781 w1784] -> w1769
              tunnel: w1768 -> [w1781 w1783]
              tunnel: w1760 -> [_ w1782]
              frame False {
              }
              frame True {
                n850 = Bundle By Name(cluster=w1782, "QueueAction"=DeviceQueue_Action."Spectrometer_Preview") -> (w1785:T11)
                n851 = Enqueue Element(queue=w1783, element=w1785) -> (queue out=w1784:refnum<queue>)  [unwired: 2 in, 2 out]
              }
            }
            n852 = Bundle By Name(cluster=w1775, "Data_Raw"=w1772, "QueueAction"=DataQueue_Action."Spectrometer_Preview", "TabControl"=w1761) -> (w1776:T8)
            n853 = Enqueue Element(queue=w1774, element=w1776) -> (queue out=w1773:refnum<queue>)  [unwired: 2 in, 2 out]
            n854 = Bundle By Name(cluster=w1767, "Abstract_CCD.lvclass"=w1763) -> (w1766:T6)
          }
          frame "Spectrometer_StartMeasurement" {
            n855 = Unbundle By Name(w1789) -> ("Abstract_CCD.lvclass"=w1793:refnum<class "Abstract_CCD.lvclass">)
            n856 = call-dynamic "StartMeasure.vi"("error in (no error)"=w1794, "Frames"=-1, "Abstract_CCD in"=w1793) -> ("error out"=w1792:errorcluster, "Abstract_CCD out"=w1788:refnum<class "Abstract_CCD.lvclass">)  [unwired: 7 in]
            n857 = Bundle By Name(cluster=w1789, "Abstract_CCD.lvclass"=w1788) -> (w1787:T6)
          }
          frame "Spectrometer_StopMeasurement" {
            n858 = Unbundle By Name(w1801) -> ("Abstract_CCD.lvclass"=w1803:refnum<class "Abstract_CCD.lvclass">)
            n859 = call-dynamic "StopMeasurement.vi"("error in (no error)"=w1802, "Abstract_CCD in"=w1803) -> ("error out"=w1799:errorcluster, "Abstract_CCD out"=w1800:refnum<class "Abstract_CCD.lvclass">)  [unwired: 8 in]
            n860 = Bundle By Name(cluster=w1801, "Abstract_CCD.lvclass"=w1800) -> (w1796:T6)
          }
          frame "Spectrometer_GetData" {
            w1813 = T8 {"QueueAction"=enum."TimeOut", "Data"=[], "Data_Raw"=[], "Data_Dark"=[], "Data_Ref"=[], "Device Information"=[], "Numeric Control"=0.0, "Boolean"=FALSE, "Wavelength"=[], "Time"=[], "Time Stamp"=timestamp(0 s since 1904-01-01), "Numeric Control 2"=0.0, "TabControl"=enum."Measure", "Numeric Control 3"=0.0}  # DataQueue
            n861 = Unbundle By Name(w1810) -> ("Abstract_CCD.lvclass"=w1815:refnum<class "Abstract_CCD.lvclass">)
            n862 = Unbundle By Name(w1816) -> ("Numeric 1"=w1807:dbl)
            n863 = call-dynamic "Measure_GetData.vi"("error in (no error)"=w1814, "SpectraCount"=w1807, "Abstract_CCD in"=w1815) -> ("error out"=w1805:errorcluster, "Data_Raw"=w1804:T14, "Time"=w1806:dbl[])  [unwired: 5 in, 1 out]
            n864 = Bundle By Name(cluster=w1813, "QueueAction"=DataQueue_Action."Spectrometer_Measure", "Data_Raw"=w1804, "Time"=w1806) -> (w1812:T8)
            n865 = Enqueue Element(queue=w1809, element=w1812) -> (queue out=w1808:refnum<queue>)  [unwired: 2 in, 2 out]
          }
          frame "Spectrometer_GetData_Short" {
            w1864 = 0 ("index (page)")
            w1859 = nan
            w1880 = T8 {"QueueAction"=enum."TimeOut", "Data"=[], "Data_Raw"=[], "Data_Dark"=[], "Data_Ref"=[], "Device Information"=[], "Numeric Control"=0.0, "Boolean"=FALSE, "Wavelength"=[], "Time"=[], "Time Stamp"=timestamp(0 s since 1904-01-01), "Numeric Control 2"=0.0, "TabControl"=enum."Measure", "Numeric Control 3"=0.0}  # DataQueue
            # "Frames"
            # "Start Time + Offset"
            n866 = Unbundle By Name(w1861) -> ("Abstract_CCD.lvclass"=w1869:refnum<class "Abstract_CCD.lvclass">)
            n867 = local read "Seconds to Spin_Short"() -> (w1844:dbl[unit])
            n868 = Unbundle By Name(w1881) -> ("Numeric 2"=w1835:dbl)
            n869 = call <vilib>:"High Resolution Relative Seconds.vi"() -> ("relative seconds"=w1875:dbl)
            n870 = node("Time Detect") -> (w1874:dbl)
            n871 = To Long Integer(number=w1835) -> (32bit integer=w1830:i32)
            n872 = node(w1844) -> (w1873:dbl)
            n873 = call-dynamic "Measure_GetData_SpectraOutput.vi"("error in (no error)"=w1870, "Abstract_CCD in"=w1869) -> ("error out"=w1872:errorcluster, "Spectra"=w1865:dbl[], "Abstract_CCD out"=w1871:refnum<class "Abstract_CCD.lvclass">, "Time"=w1856:dbl)  [unwired: 6 in]
            n874 = Compound Arithmetic op=ADD(w1875, w1873, w1874) -> (w1862:dbl)
            n875 = Initialize Array(w1859, w1830) -> (w1858:dbl[])
            n876 = Array Size(array=w1865) -> (size(s)=w1868:i32)
            n877 = Initialize Array(w1859, w1830, 1 ("index"), w1868) -> (w1866:dbl[][][])
            n878 = Replace Array Subset(array=w1858, new element=w1856, index=0) -> (w1855:dbl[])
            n879 = Replace Array Subset(array=w1866, new element=w1865, index (dim 0)=w1864, index (dim 1)=w1864) -> (w1863:dbl[][][])  [unwired: 1 in]
            n880 = while {
              shift-right: [w1935] -> w1840
              shift-left: w1872 -> [w1936]
              shift-right: [w1932] -> w1841
              shift-left: w1863 -> [w1934]
              tunnel: w1862 -> [w1931]
              shift-right: [w1928] -> w1842
              shift-left: w1855 -> [w1930]
              tunnel: [w1925] -> w1843
              tunnel: [w1923] -> w1838
              shift-right: [w1922] -> w1839
              shift-left: w1871 -> [w1937]
              i -> [w1924]
              stop <- w1926 stop-if-true
              # "Wait for correct Time"
              n881 = call <vilib>:"High Resolution Relative Seconds.vi"() -> ("relative seconds"=w1927:dbl)
              n882 = call-dynamic "Measure_GetData_SpectraOutput.vi"("error in (no error)"=w1936, "Abstract_CCD in"=w1937) -> ("error out"=w1935:errorcluster, "Spectra"=w1925:dbl[], "Abstract_CCD out"=w1922:refnum<class "Abstract_CCD.lvclass">, "Time"=w1929:dbl)  [unwired: 6 in]
              n883 = Greater?(x=w1927, y=w1931) -> (0:w1926:bool)
              n884 = Increment(x=w1924) -> (x+1=w1923:i32)
              n885 = Replace Array Subset(array=w1930, new element=w1929, index=w1923) -> (w1928:dbl[])
              n886 = Replace Array Subset(array=w1934, new element=w1925, index (dim 0)=w1923, index (dim 1)=0 ("disabled index (row)")) -> (w1932:dbl[][][])  [unwired: 1 in]
            }
            n887 = local read "WL-Det\nPos"() -> (w1837:i32)
            n888 = Increment(x=w1838) -> (x+1=w1823:i32)
            n889 = Index Array(array=w1843, index=w1837) -> (element=w1836:dbl)
            n890 = while {
              shift-right: [w1915] -> w1832
              shift-left: w1842 -> [w1917]
              shift-right: [w1913] -> w1833
              shift-left: w1841 -> [w1914]
              shift-right: [w1905] -> w1822
              shift-left: w1840 -> [w1921]
              tunnel: w1823 -> [w1919]
              tunnel: w1837 -> [w1907]
              tunnel: w1830 -> [w1904]
              tunnel: [w1899] -> w1828
              tunnel: [w1898] -> w1819
              shift-right: [w1900] -> w1831
              shift-left: w1839 -> [w1920]
              i -> [w1918]
              stop <- w1901 stop-if-true
              # "Wait for threshold"
              n891 = call-dynamic "Measure_GetData_SpectraOutput.vi"("error in (no error)"=w1921, "Abstract_CCD in"=w1920) -> ("error out"=w1905:errorcluster, "Spectra"=w1908:dbl[], "Abstract_CCD out"=w1900:refnum<class "Abstract_CCD.lvclass">, "Time"=w1916:dbl)  [unwired: 6 in]
              n892 = Add(x=w1919, y=w1918) -> (x+y=w1899:i32)
              n893 = Index Array(array=w1908, index=w1907) -> (element=w1909:dbl)
              n894 = Replace Array Subset(array=w1917, new element=w1916, index=w1899) -> (w1915:dbl[])
              n895 = Replace Array Subset(array=w1914, new element=w1908, index (dim 0)=w1899, index (dim 1)=0 ("disabled index (row)")) -> (w1913:dbl[][][])  [unwired: 1 in]
              n896 = Divide(x=w1909, y="Reference\nValue") -> (x/y=w1910:dbl)
              n897 = Less?(x=w1910, y="Threshold") -> (x < y?=w1903:bool)
              n898 = Equal?(x=w1904, y=w1899) -> (x = y?=w1902:bool)
              n899 = call <vilib>:"High Resolution Relative Seconds.vi"() -> ("relative seconds"=w1898:dbl)
              n900 = Or(x=w1902, y=w1903) -> (x .or. y?=w1901:bool)
            }
            n901 = local write "Reference\nValue"(w1836) -> ()
            n902 = Unbundle By Name(w1861) -> ("SpinCoater.lvclass"=w1834:refnum<class "SpinCoater.lvclass">)
            n903 = Subtract(x=w1830, y=w1828) -> (x-y=w1829:i32)
            n904 = Increment(x=w1828) -> (x+1=w1826:i32)
            n905 = call-dynamic "Stop_Short.vi"("error in (no error)"=w1822, "SpinCoater in"=w1834) -> ("error out"=w1821:errorcluster)  [unwired: 8 in, 1 out]
            n906 = for {
              N: w1829 -> [_]
              shift-right: [w1893] -> w1827
              shift-left: w1832 -> [w1892]
              shift-right: [w1889] -> w1825
              shift-left: w1833 -> [w1890]
              tunnel: w1826 -> [w1895]
              shift-right: [w1885] -> w1824
              shift-left: w1822 -> [w1897]
              shift-right: [w1884] -> _
              shift-left: w1831 -> [w1896]
              i -> [w1894]
              n907 = call-dynamic "Measure_GetData_SpectraOutput.vi"("error in (no error)"=w1897, "Abstract_CCD in"=w1896) -> ("error out"=w1885:errorcluster, "Spectra"=w1886:dbl[], "Abstract_CCD out"=w1884:refnum<class "Abstract_CCD.lvclass">, "Time"=w1891:dbl)  [unwired: 6 in]
              n908 = Add(x=w1894, y=w1895) -> (x+y=w1888:i32)
              n909 = Replace Array Subset(array=w1892, new element=w1891, index=w1888) -> (w1893:dbl[])
              n910 = Replace Array Subset(array=w1890, new element=w1886, index (dim 0)=w1888, index (dim 1)=0 ("disabled index (row)")) -> (w1889:dbl[][][])  [unwired: 1 in]
            }
            n911 = flat-sequence {
              tunnel: w1821 -> [_]
              tunnel: [w1883] -> w1820
              frame #0 {
                n912 = call <vilib>:"High Resolution Relative Seconds.vi"() -> ("relative seconds"=w1883:dbl)
              }
            }
            n913 = Subtract(x=w1819, y=w1820) -> (x-y=→"x-y":dbl)
            n914 = Array Size(array=w1825) -> (size(s)=w1853:i32[])
            n915 = Index Array(array=w1853, index #1=0 ("index"), index #2=1 ("index"), index #3=2 ("index")) -> (element #1=w1850:i32, element #2=w1851:i32, element #3=w1852:i32)
            n916 = Bundle By Name(cluster=T15 {"Image"=[], "Frame Size"={"F"=0, "Y"=0, "X"=0}} ("Cluster"), "Image"=w1825, "Frame Size.F"=w1850, "Frame Size.Y"=w1851, "Frame Size.X"=w1852) -> (w1846:T15)
            n917 = Build Array(w1846) -> (w1845:T14)
            n918 = Bundle By Name(cluster=w1880, "QueueAction"=DataQueue_Action."Spectrometer_Measure", "Data_Raw"=w1845, "Time"=w1827) -> (w1879:T8)
            n919 = Enqueue Element(queue=w1877, element=w1879) -> (queue out=w1876:refnum<queue>)  [unwired: 2 in, 2 out]
          }
          frame "Spectrometer_SetIntegrationTime" {
            n920 = Unbundle By Name(w1946) -> ("Numeric 1"=w1948:dbl)
            n921 = Unbundle By Name(w1942) -> ("Abstract_CCD.lvclass"=w1950:refnum<class "Abstract_CCD.lvclass">)
            n922 = Unbundle By Name(w1946) -> ("TabControl"=w1938:T10, "Boolean 1"=w1945:bool)
            n923 = node(w1948) -> (w1947:dbl[unit])
            n924 = call-dynamic "Set_ExposureTime.vi"("error in (no error)"=w1949, "Exposure Time"=w1947, "Abstract_CCD in"=w1950) -> ("error out"=w1953:errorcluster, "Abstract_CCD out"=w1952:refnum<class "Abstract_CCD.lvclass">)  [unwired: 7 in]
            n925 = call-dynamic "Get_FrameRate.vi"("error in (no error)"=w1953, "Abstract_CCD in"=w1952) -> ("error out"=w1943:errorcluster, "Frame Rate"=w1944:dbl[unit], "Abstract_CCD out"=w1941:refnum<class "Abstract_CCD.lvclass">)  [unwired: 7 in]
            n926 = Bundle By Name(cluster=w1942, "Abstract_CCD.lvclass"=w1941) -> (w1940:T6)
            n927 = case shown="\"Measure\"" w1938 {
              tunnel: w1945 -> [_ _ w1956]
              tunnel: w1944 -> [_ w1954 w1955]
              frame Default {
              }
              frame "Spectral Stability" {
                "SpectralStability_FrameRate" <- w1954
              }
              frame "Measure" {
                n928 = case shown="True" w1956 {
                  tunnel: w1955 -> [_ w1960]
                  frame False {
                  }
                  frame True {
                    n929 = property on="Program Spin Coater" class="Arr (strict)"() -> ("Value"=w1957:T2)  [unwired: 2 in, 2 out]
                    n930 = property on="Seconds to Spin_Normal" class="DigNum (strict)"() -> ("Value"=w1962:dbl[unit])  [unwired: 2 in, 2 out]
                    n931 = property on="Seconds after Spin" class="DigNum (strict)"() -> ("Value"=w1961:dbl[unit])  [unwired: 2 in, 2 out]
                    n932 = call "CalculateFrames_v03.vi"("Program Spin Coater"=w1957, "Seconds End"=w1961, "Seconds Start"=w1962, "Frame Rate"=w1960) -> ("Time"=w1959:dbl, "Frames"=w1958:i32)  [unwired: 6 in]
                    n933 = property on="Frames" class="DigNum (strict)"("Value"=w1958) -> ()  [unwired: 2 in, 2 out]
                    n934 = property on="Overall Time" class="DigNum (strict)"("Value"=w1959) -> ()  [unwired: 2 in, 2 out]
                  }
                }
                "Measure_FrameRate" <- w1955
              }
            }
          }
          frame "Spectrometer_SetFrames" {
            n935 = Unbundle By Name(w1964) -> ("Abstract_CCD.lvclass"=w1969:refnum<class "Abstract_CCD.lvclass">)
            n936 = Unbundle By Name(w1972) -> ("Numeric 1"=w1966:dbl)
            n937 = call-dynamic "Set_Frames.vi"("error in (no error)"=w1968, "Frames"=w1966, "Abstract_CCD in"=w1969) -> ("error out"=w1967:errorcluster, "Abstract_CCD out"=w1963:refnum<class "Abstract_CCD.lvclass">)  [unwired: 7 in]
            n938 = Bundle By Name(cluster=w1964, "Abstract_CCD.lvclass"=w1963) -> (w1965:T6)
          }
          frame "Spectrometer_SetDarkspec" {
            w1987 = T8 {"QueueAction"=enum."TimeOut", "Data"=[], "Data_Raw"=[], "Data_Dark"=[], "Data_Ref"=[], "Device Information"=[], "Numeric Control"=0.0, "Boolean"=FALSE, "Wavelength"=[], "Time"=[], "Time Stamp"=timestamp(0 s since 1904-01-01), "Numeric Control 2"=0.0, "TabControl"=enum."Measure", "Numeric Control 3"=0.0}  # DataQueue
            n939 = Unbundle By Name(w1982) -> ("Abstract_CCD.lvclass"=w1980:refnum<class "Abstract_CCD.lvclass">)
            n940 = call-dynamic "Measure.vi"("error in (no error)"=w1979, "Abstract_CCD in"=w1980) -> ("error out"=w1977:errorcluster, "Data Raw"=w1984:T14, "Abstract_CCD out"=w1978:refnum<class "Abstract_CCD.lvclass">)  [unwired: 3 in, 4 out]
            n941 = Bundle By Name(cluster=w1987, "QueueAction"=DataQueue_Action."Set_Dark", "Data_Dark"=w1984) -> (w1988:T8)
            n942 = Enqueue Element(queue=w1986, element=w1988) -> (queue out=w1983:refnum<queue>)  [unwired: 2 in, 2 out]
            n943 = Bundle By Name(cluster=w1982, "Abstract_CCD.lvclass"=w1978) -> (w1981:T6)
            n944 = property on="Measure:\nRecord_Darkspec" class="Bool (strict)"(error in=w1977, "Value"=FALSE ("Record_Darkspec")) -> (error out=w1975:errorcluster)  [unwired: 1 in, 1 out]
            n945 = property on="SpectralStability:\nRecord_Darkspec" class="Bool (strict)"(error in=w1975, "Value"=FALSE ("SpectralStability:\nRecord_Darkspec")) -> (error out=w1974:errorcluster)  [unwired: 1 in, 1 out]
          }
          frame "Spectrometer_SetReference" {
            w2002 = T8 {"QueueAction"=enum."TimeOut", "Data"=[], "Data_Raw"=[], "Data_Dark"=[], "Data_Ref"=[], "Device Information"=[], "Numeric Control"=0.0, "Boolean"=FALSE, "Wavelength"=[], "Time"=[], "Time Stamp"=timestamp(0 s since 1904-01-01), "Numeric Control 2"=0.0, "TabControl"=enum."Measure", "Numeric Control 3"=0.0}  # DataQueue
            n946 = Unbundle By Name(w1997) -> ("Abstract_CCD.lvclass"=w1994:refnum<class "Abstract_CCD.lvclass">)
            n947 = call-dynamic "Measure.vi"("error in (no error)"=w1995, "Abstract_CCD in"=w1994) -> ("error out"=w1992:errorcluster, "Data Raw"=w1999:T14, "Abstract_CCD out"=w1993:refnum<class "Abstract_CCD.lvclass">)  [unwired: 3 in, 4 out]
            n948 = Bundle By Name(cluster=w2002, "QueueAction"=DataQueue_Action."Set_Ref", "Data_Ref"=w1999) -> (w2003:T8)
            n949 = Enqueue Element(queue=w2001, element=w2003) -> (queue out=w1998:refnum<queue>)  [unwired: 2 in, 2 out]
            n950 = Bundle By Name(cluster=w1997, "Abstract_CCD.lvclass"=w1993) -> (w1996:T6)
            n951 = property on="Record RefSpec" class="Bool (strict)"(error in=w1992, "Value"=FALSE ("Record RefSpec")) -> (error out=w1991:errorcluster)  [unwired: 1 in, 1 out]
          }
          frame "Spectrometer_SetTriggerMode" {
            n952 = Unbundle By Name(w2008) -> ("Abstract_CCD.lvclass"=w2013:refnum<class "Abstract_CCD.lvclass">)
            n953 = Unbundle By Name(w2012) -> ("Numeric 1"=w2010:dbl)
            n954 = call-dynamic "Set_TriggerMode.vi"("error in (no error)"=w2011, "Trigger Mode"=w2010, "Abstract_CCD in"=w2013) -> ("error out"=w2009:errorcluster, "Abstract_CCD out"=w2007:refnum<class "Abstract_CCD.lvclass">)  [unwired: 7 in]
            n955 = Bundle By Name(cluster=w2008, "Abstract_CCD.lvclass"=w2007) -> (w2006:T6)
          }
          frame "Spectrometer_DeviceInformation" {
            w2021 = T8 {"QueueAction"=enum."TimeOut", "Data"=[], "Data_Raw"=[], "Data_Dark"=[], "Data_Ref"=[], "Device Information"=[], "Numeric Control"=0.0, "Boolean"=FALSE, "Wavelength"=[], "Time"=[], "Time Stamp"=timestamp(0 s since 1904-01-01), "Numeric Control 2"=0.0, "TabControl"=enum."Measure", "Numeric Control 3"=0.0}  # DataQueue
            n956 = Unbundle By Name(w2015) -> ("Abstract_CCD.lvclass"=w2023:refnum<class "Abstract_CCD.lvclass">)
            n957 = call-dynamic "Get_DeviceInformation.vi"("error in (no error)"=w2022, "Abstract_CCD in"=w2023) -> ("error out"=w2017:errorcluster, "Array"=w2024:string[])  [unwired: 7 in, 1 out]
            n958 = Bundle By Name(cluster=w2021, "QueueAction"=DataQueue_Action."Transfer_Settings", "Device Information"=w2024) -> (w2019:T8)
            n959 = Enqueue Element(queue=w2020, element=w2019, error in (no error)=w2017) -> (queue out=w2018:refnum<queue>, error out=w2016:errorcluster)  [unwired: 1 in, 1 out]
          }
          frame "Arduino_Init" {
            n960 = Unbundle By Name(w2036) -> ("SpinCoater.lvclass"=w2035:refnum<class "SpinCoater.lvclass">)
            n961 = call-dynamic "Init.vi"("error in (no error)"=w2034, "Variant"="Port Arduino", "SpinCoater in"=w2035) -> ("error out"=w2031:errorcluster, "SpinCoater out"=w2032:refnum<class "SpinCoater.lvclass">)  [unwired: 7 in]
            n962 = call-dynamic "IsInit.vi"("error in (no error)"=w2031, "SpinCoater in"=w2032) -> ("error out"=w2028:errorcluster, "Init"=w2029:bool, "SpinCoater out"=w2030:refnum<class "SpinCoater.lvclass">)  [unwired: 7 in]
            n963 = property on="Arduino" class="Bool (strict)"("Value"=w2029) -> ()  [unwired: 2 in, 2 out]
            n964 = case shown="False" w2029 {
              tunnel: [w2040 w2042] -> w2037
              tunnel: w2028 -> [w2040 w2042]
              frame False {
              }
              frame True {
                n965 = property on="Program Spin Coater" class="Arr (strict)"() -> ("Value"=w2041:T2)  [unwired: 2 in, 2 out]
                n966 = property on="Program Spin Coater" class="Arr (strict)"("Val(Sgnl)"=w2041) -> ()  [unwired: 2 in, 2 out]
              }
            }
            n967 = Bundle By Name(cluster=w2036, "SpinCoater.lvclass"=w2030) -> (w2038:T6)
          }
          frame "Arduino_Close" {
            n968 = Unbundle By Name(w2045) -> ("SpinCoater.lvclass"=w2053:refnum<class "SpinCoater.lvclass">)
            n969 = property on="Arduino" class="Bool (strict)"() -> (error out=w2047:errorcluster, "Value"=w2046:bool)  [unwired: 2 in, 1 out]
            n970 = property on="Arduino" class="Bool (strict)"(error in=w2047, "Value"=FALSE ("Arduino")) -> ()  [unwired: 1 in, 2 out]
            n971 = case shown="False" w2046 {
              tunnel: w2053 -> [w2054 w2059]
              tunnel: w2052 -> [w2055 w2058]
              tunnel: [w2055 w2057] -> w2051
              tunnel: [w2054 w2056] -> w2044
              frame False {
              }
              frame True {
                n972 = call-dynamic "Close.vi"("error in (no error)"=w2058, "SpinCoater in"=w2059) -> ("error out"=w2057:errorcluster, "SpinCoater out"=w2056:refnum<class "SpinCoater.lvclass">)  [unwired: 8 in]
              }
            }
            n973 = Bundle By Name(cluster=w2045, "SpinCoater.lvclass"=w2044) -> (w2043:T6)
          }
          frame "Arduino_LoadProgram" {
            n974 = Unbundle By Name(w2071) -> ("Spin Prg v07"=w2062:T2, "Numeric 1"=w2070:dbl, "Numeric 2"=w2061:dbl)
            n975 = Unbundle By Name(w2066) -> ("SpinCoater.lvclass"=w2069:refnum<class "SpinCoater.lvclass">)
            n976 = node(w2070) -> (w2068:dbl[unit])
            n977 = node(w2061) -> (w2060:dbl[unit])
            n978 = call-dynamic "Program_Load_v03.vi"("Time Spin"=w2060, "error in (no error)"=w2067, "Time Start"=w2068, "Program Spin Coater"=w2062, "SpinCoater in"=w2069) -> ("error out"=w2064:errorcluster, "SpinCoater out"=w2065:refnum<class "SpinCoater.lvclass">)  [unwired: 5 in]
            n979 = Bundle By Name(cluster=w2066, "SpinCoater.lvclass"=w2065) -> (w2063:T6)
          }
          frame "Arduino_StartProgram" {
            n980 = Unbundle By Name(w2081) -> ("SpinCoater.lvclass"=w2078:refnum<class "SpinCoater.lvclass">)
            n981 = Unbundle By Name(w2075) -> ("Numeric 1"=w2074:dbl)
            n982 = call-dynamic "Program_Run.vi"("error in (no error)"=w2077, "Numeric"=w2074, "SpinCoater in"=w2078) -> ("error out"=w2076:errorcluster)  [unwired: 7 in, 1 out]
            n983 = property on="Action" class="Str"("Value"="Measuring" ("Action")) -> ()  [unwired: 2 in, 2 out]
          }
          frame "Arduino_SetSpeed" {
            n984 = Unbundle By Name(w2090) -> ("SpinCoater.lvclass"=w2086:refnum<class "SpinCoater.lvclass">)
            n985 = Unbundle By Name(w2089) -> ("Numeric 1"=w2088:dbl)
            n986 = To Unsigned Long Integer(number=w2088) -> (unsigned 32bit integer=w2084:u32)
            n987 = call-dynamic "Debug_SetSpeed.vi"("error in (no error)"=w2085, "Speed"=w2084, "SpinCoater in"=w2086) -> ("error out"=w2083:errorcluster)  [unwired: 7 in, 1 out]
          }
          frame "Arduino_SetMillis" {
            n988 = Unbundle By Name(w2096) -> ("SpinCoater.lvclass"=w2095:refnum<class "SpinCoater.lvclass">)
            n989 = Unbundle By Name(w2098) -> ("Numeric 1"=w2100:dbl)
            n990 = To Unsigned Long Integer(number=w2100) -> (unsigned 32bit integer=w2092:u32)
            n991 = call-dynamic "Debug_SetMillis.vi"("error in (no error)"=w2094, "Milliseconds"=w2092, "SpinCoater in"=w2095) -> ("error out"=w2093:errorcluster)  [unwired: 7 in, 1 out]
          }
          frame "Arduino_StopSpin" {
            n992 = Unbundle By Name(w2104) -> ("SpinCoater.lvclass"=w2103:refnum<class "SpinCoater.lvclass">)
            n993 = call-dynamic "Stop_Spin.vi"("error in (no error)"=w2102, "SpinCoater in"=w2103) -> ("error out"=w2101:errorcluster)  [unwired: 8 in, 1 out]
          }
          frame "Arduino_ShortStop" {
            n994 = Unbundle By Name(w2110) -> ("SpinCoater.lvclass"=w2109:refnum<class "SpinCoater.lvclass">)
            n995 = call-dynamic "Stop_Short.vi"("error in (no error)"=w2108, "SpinCoater in"=w2109) -> ("error out"=w2107:errorcluster)  [unwired: 8 in, 1 out]
          }
          frame "Arduino_Shutter_SetPosition" {
            n996 = Unbundle By Name(w2119) -> ("Numeric 1"=w2118:dbl)
            n997 = Unbundle By Name(w2121) -> ("SpinCoater.lvclass"=w2120:refnum<class "SpinCoater.lvclass">)
            n998 = Number To Decimal String(number=w2118) -> (decimal integer string=w2117:string)  [unwired: 1 in]
            n999 = Concatenate Strings("!shu_M" ("string"), w2117) -> (w2115:string)
            n1000 = call-dynamic "Send_String.vi"("error in (no error)"=w2114, "String"=w2115, "SpinCoater in"=w2120) -> ("error out"=w2113:errorcluster)  [unwired: 6 in, 2 out]
          }
          frame "Arduino_Shutter_Close" {
            n1001 = Unbundle By Name(w2128) -> ("SpinCoater.lvclass"=w2127:refnum<class "SpinCoater.lvclass">)
            n1002 = call-dynamic "Send_String.vi"("error in (no error)"=w2126, "String"="!shuOFF" ("string"), "SpinCoater in"=w2127) -> ("error out"=w2125:errorcluster)  [unwired: 6 in, 2 out]
          }
          frame "Arduino_Shutter_Open" {
            n1003 = Unbundle By Name(w2135) -> ("SpinCoater.lvclass"=w2134:refnum<class "SpinCoater.lvclass">)
            n1004 = call-dynamic "Send_String.vi"("error in (no error)"=w2133, "String"="!shuON" ("string"), "SpinCoater in"=w2134) -> ("error out"=w2132:errorcluster)  [unwired: 6 in, 2 out]
          }
          frame "Measure_Stop" {
            w2144 = T8 {"QueueAction"=enum."TimeOut", "Data"=[], "Data_Raw"=[], "Data_Dark"=[], "Data_Ref"=[], "Device Information"=[], "Numeric Control"=0.0, "Boolean"=FALSE, "Wavelength"=[], "Time"=[], "Time Stamp"=timestamp(0 s since 1904-01-01), "Numeric Control 2"=0.0, "TabControl"=enum."Measure", "Numeric Control 3"=0.0}  # DataQueue
            n1005 = Bundle By Name(cluster=w2144, "QueueAction"=DataQueue_Action."Stop_Measurement") -> (w2145:T8)
            n1006 = Enqueue Element(queue=w2142, element=w2145, error in (no error)=w2139) -> (queue out=w2141:refnum<queue>, error out=w2138:errorcluster)  [unwired: 1 in, 1 out]
          }
          frame "Measure_InSitu" {
            w2186 = T11 {"QueueAction"=enum."TimeOut", "Numeric 1"=0.0, "Numeric 2"=0.0, "Boolean 1"=FALSE, "Boolean 2"=FALSE, "Spin Program"=[], "Spin Prg v07"=[], "Time Stamp"=timestamp(0 s since 1904-01-01), "TabControl"=enum."Measure"}  # Device Queue
            w2193 = T11 {"QueueAction"=enum."TimeOut", "Numeric 1"=0.0, "Numeric 2"=0.0, "Boolean 1"=FALSE, "Boolean 2"=FALSE, "Spin Program"=[], "Spin Prg v07"=[], "Time Stamp"=timestamp(0 s since 1904-01-01), "TabControl"=enum."Measure"}  # Device Queue
            n1007 = Bundle By Name(cluster=w2193, "QueueAction"=DeviceQueue_Action."Spectrometer_SetTriggerMode", "Numeric 1"=1.0) -> (w2191:T11)
            n1008 = Bundle By Name(cluster=w2186, "QueueAction"=DeviceQueue_Action."Spectrometer_DeviceInformation") -> (w2183:T11)
            n1009 = Bundle By Name(cluster=w2183, "QueueAction"=DeviceQueue_Action."Spectrometer_StartMeasurement") -> (w2179:T11)
            n1010 = Enqueue Element(queue=w2192, element=w2191, error in (no error)=w2148) -> (queue out=w2188:refnum<queue>, error out=w2189:errorcluster)  [unwired: 1 in, 1 out]
            n1011 = property on="Frames" class="DigNum (strict)"() -> ("Value"=w2149:i32)  [unwired: 2 in, 2 out]
            n1012 = Bundle By Name(cluster=w2179, "QueueAction"=DeviceQueue_Action."Arduino_StartProgram") -> (w2174:T11)
            n1013 = Enqueue Element(queue=w2188, element=w2183, error in (no error)=w2189) -> (queue out=w2185:refnum<queue>, error out=w2184:errorcluster)  [unwired: 1 in, 1 out]
            n1014 = Bundle By Name(cluster=w2174, "QueueAction"=DeviceQueue_Action."Spectrometer_GetData", "Numeric 1"="Dividider Get Spectra") -> (w2169:T11)
            n1015 = Divide(x=w2149, y="Dividider Get Spectra") -> (x/y=w2181:dbl)
            n1016 = Round Toward +Infinity(x=w2181) -> (ceil(x): smallest int >= x=w2180:dbl)
            n1017 = Enqueue Element(queue=w2185, element=w2179, error in (no error)=w2184) -> (queue out=w2178:refnum<queue>, error out=w2177:errorcluster)  [unwired: 1 in, 1 out]
            n1018 = Enqueue Element(queue=w2178, element=w2174, error in (no error)=w2177) -> (queue out=w2175:refnum<queue>, error out=w2172:errorcluster)  [unwired: 1 in, 1 out]
            n1019 = for {
              N: w2180 -> [_]
              shift-right: [w2196] -> w2171
              shift-left: w2175 -> [w2200]
              tunnel: w2169 -> [w2197]
              shift-right: [w2198] -> w2170
              shift-left: w2172 -> [w2199]
              n1020 = Enqueue Element(queue=w2200, element=w2197, error in (no error)=w2199) -> (queue out=w2196:refnum<queue>, error out=w2198:errorcluster)  [unwired: 1 in, 1 out]
            }
            n1021 = Bundle By Name(cluster=w2169, "QueueAction"=DeviceQueue_Action."Spectrometer_StopMeasurement") -> (w2165:T11)
            n1022 = property on="Measure_FramesSpectrometer" class="DigNum (strict)"() -> ("Value"=w2151:dbl)  [unwired: 2 in, 2 out]
            n1023 = Bundle By Name(cluster=w2165, "QueueAction"=DeviceQueue_Action."Measure_Stop") -> (w2158:T11)
            n1024 = Enqueue Element(queue=w2171, element=w2165, error in (no error)=w2170) -> (queue out=w2166:refnum<queue>, error out=w2167:errorcluster)  [unwired: 1 in, 1 out]
            n1025 = Bundle By Name(cluster=w2158, "QueueAction"=DeviceQueue_Action."Spectrometer_SetTriggerMode", "Numeric 1"=0.0) -> (w2153:T11)
            n1026 = Enqueue Element(queue=w2166, element=w2158, error in (no error)=w2167) -> (queue out=w2161:refnum<queue>, error out=w2162:errorcluster)  [unwired: 1 in, 1 out]
            n1027 = Bundle By Name(cluster=w2153, "QueueAction"=DeviceQueue_Action."Spectrometer_SetFrames", "Numeric 1"=w2151) -> (w2150:T11)
            n1028 = Enqueue Element(queue=w2161, element=w2153, error in (no error)=w2162) -> (queue out=w2160:refnum<queue>, error out=w2159:errorcluster)  [unwired: 1 in, 1 out]
            n1029 = Enqueue Element(queue=w2160, element=w2150, error in (no error)=w2159) -> (queue out=w2154:refnum<queue>, error out=w2155:errorcluster)  [unwired: 1 in, 1 out]
          }
          frame "Measure_InSituAdvanced" {
            w2288 = T11 {"QueueAction"=enum."TimeOut", "Numeric 1"=0.0, "Numeric 2"=0.0, "Boolean 1"=FALSE, "Boolean 2"=FALSE, "Spin Program"=[], "Spin Prg v07"=[], "Time Stamp"=timestamp(0 s since 1904-01-01), "TabControl"=enum."Measure"}  # Device Queue
            n1030 = property on="Dividider Get Spectra" class="DigNum (strict)"() -> ("Value"=w2247:u32)  [unwired: 2 in, 2 out]
            n1031 = Bundle By Name(cluster=w2288, "QueueAction"=DeviceQueue_Action."Spectrometer_SetTriggerMode", "Numeric 1"=1.0) -> (w2243:T11)
            n1032 = Bundle By Name(cluster=w2243, "QueueAction"=DeviceQueue_Action."Spectrometer_DeviceInformation") -> (w2280:T11)
            n1033 = Bundle By Name(cluster=w2280, "QueueAction"=DeviceQueue_Action."Spectrometer_StartMeasurement") -> (w2276:T11)
            n1034 = Enqueue Element(queue=w2287, element=w2243, error in (no error)=w2248) -> (queue out=w2284:refnum<queue>, error out=w2285:errorcluster)  [unwired: 1 in, 1 out]
            n1035 = Bundle By Name(cluster=w2276, "QueueAction"=DeviceQueue_Action."Arduino_StartProgram", "Numeric 1"=1.0) -> (w2271:T11)
            n1036 = property on="Frames" class="DigNum (strict)"() -> ("Value"=w2249:i32)  [unwired: 2 in, 2 out]
            n1037 = Unbundle By Name(w2230) -> ("Time Stamp"=w2229:timestamp)
            n1038 = Enqueue Element(queue=w2284, element=w2280, error in (no error)=w2285) -> (queue out=w2282:refnum<queue>, error out=w2281:errorcluster)  [unwired: 1 in, 1 out]
            n1039 = Divide(x=w2249, y=w2247) -> (x/y=w2278:dbl)
            n1040 = Bundle By Name(cluster=w2271, "QueueAction"=DeviceQueue_Action."Spectrometer_GetData", "Numeric 1"=w2247) -> (w2266:T11)
            n1041 = Round Toward +Infinity(x=w2278) -> (ceil(x): smallest int >= x=w2277:dbl)
            n1042 = Enqueue Element(queue=w2282, element=w2276, error in (no error)=w2281) -> (queue out=w2275:refnum<queue>, error out=w2274:errorcluster)  [unwired: 1 in, 1 out]
            n1043 = Enqueue Element(queue=w2275, element=w2271, error in (no error)=w2274) -> (queue out=w2272:refnum<queue>, error out=w2269:errorcluster)  [unwired: 1 in, 1 out]
            n1044 = Bundle By Name(cluster=w2266, "QueueAction"=DeviceQueue_Action."Spectrometer_StopMeasurement") -> (w2262:T11)
            n1045 = for {
              N: w2277 -> [_]
              shift-right: [w2338] -> w2268
              shift-left: w2272 -> [w2342]
              tunnel: w2266 -> [w2339]
              shift-right: [w2340] -> w2267
              shift-left: w2269 -> [w2341]
              n1046 = Enqueue Element(queue=w2342, element=w2339, error in (no error)=w2341) -> (queue out=w2338:refnum<queue>, error out=w2340:errorcluster)  [unwired: 1 in, 1 out]
            }
            n1047 = property on="Measure_FramesSpectrometer" class="DigNum (strict)"() -> ("Value"=w2250:dbl)  [unwired: 2 in, 2 out]
            n1048 = property on="periodic time" class="DigNum (strict)"() -> ("Value"=w2242:dbl[unit])  [unwired: 2 in, 2 out]
            n1049 = Bundle By Name(cluster=w2262, "QueueAction"=DeviceQueue_Action."Measure_Stop") -> (w2255:T11)
            n1050 = property on="Duration after" class="DigNum (strict)"() -> ("Value"=w2241:dbl[unit])  [unwired: 2 in, 2 out]
            n1051 = node(w2242) -> (w2212:dbl)
            n1052 = property on="periodic time" class="DigNum (strict)"() -> ("Value"=w2240:dbl[unit])  [unwired: 2 in, 2 out]
            n1053 = Bundle By Name(cluster=w2255, "QueueAction"=DeviceQueue_Action."Spectrometer_SetTriggerMode", "Numeric 1"=0.0) -> (w2252:T11)
            n1054 = Enqueue Element(queue=w2268, element=w2262, error in (no error)=w2267) -> (queue out=w2263:refnum<queue>, error out=w2264:errorcluster)  [unwired: 1 in, 1 out]
            n1055 = node(w2241) -> (w2235:dbl)
            n1056 = Bundle By Name(cluster=w2252, "QueueAction"=DeviceQueue_Action."Spectrometer_SetFrames", "Numeric 1"=w2250) -> (w2232:T11)
            n1057 = Enqueue Element(queue=w2263, element=w2255, error in (no error)=w2264) -> (queue out=w2258:refnum<queue>, error out=w2259:errorcluster)  [unwired: 1 in, 1 out]
            n1058 = node(w2240) -> (w2234:dbl)
            n1059 = Bundle By Name(cluster=w2232, "QueueAction"=DeviceQueue_Action."Wait", "Numeric 1"=w2212) -> (w2214:T11)
            n1060 = Enqueue Element(queue=w2258, element=w2252, error in (no error)=w2259) -> (queue out=w2257:refnum<queue>, error out=w2256:errorcluster)  [unwired: 1 in, 1 out]
            n1061 = Not Equal To 0?(x=w2234) -> (x != 0?=w2238:bool)
            n1062 = Not Equal To 0?(x=w2235) -> (x != 0?=w2239:bool)
            n1063 = Divide(x=w2235, y=w2234) -> (x/y=w2236:dbl)
            n1064 = Bundle By Name(cluster=w2214, "QueueAction"=DeviceQueue_Action."Spectrometer_MeasureAdvanced", "Time Stamp"=w2229) -> (w2213:T11)
            n1065 = And(x=w2239, y=w2238) -> (x .and. y?=w2237:bool)
            n1066 = Round Toward +Infinity(x=w2236) -> (ceil(x): smallest int >= x=w2233:dbl)
            n1067 = Enqueue Element(queue=w2257, element=w2232, error in (no error)=w2256) -> (queue out=w2246:refnum<queue>, error out=w2245:errorcluster)  [unwired: 1 in, 1 out]
            n1068 = Bundle By Name(cluster=w2213, "QueueAction"=DeviceQueue_Action."Arduino_SetSpeed", "Numeric 1"=1500.0) -> (w2224:T11)
            n1069 = Bundle By Name(cluster=w2224, "Numeric 1"=0.0) -> (w2216:T11)
            n1070 = property on="Measure_FrameRate" class="DigNum (strict)"() -> ("Value"=w2221:dbl[unit])  [unwired: 2 in, 2 out]
            n1071 = property on="Measure_FramesSpectrometer" class="DigNum (strict)"() -> ("Value"=w2220:dbl)  [unwired: 2 in, 2 out]
            n1072 = Divide(x=w2220, y=w2221) -> (x/y=w2222:dbl[unit])
            n1073 = Bundle By Name(cluster=w2214, "Numeric 1"=1.0) -> (w2217:T11)
            n1074 = node(w2222) -> (w2211:dbl)
            n1075 = Subtract(x=w2212, y=w2211) -> (x-y=w2210:dbl)
            n1076 = Bundle By Name(cluster=w2214, "Numeric 1"=w2210) -> (w2209:T11)
            n1077 = Round Toward +Infinity(x=w2211) -> (ceil(x): smallest int >= x=w2223:dbl)
            n1078 = Add(x=w2223, y=2.0) -> (x+y=w2218:dbl)
            n1079 = Bundle By Name(cluster=w2217, "Numeric 1"=w2218) -> (w2206:T11)
            n1080 = case shown="True" w2237 {
              tunnel: w2246 -> [w2292 w2294]
              tunnel: w2245 -> [w2291 w2297]
              tunnel: w2233 -> [_ w2310]
              tunnel: w2213 -> [_ w2309]
              tunnel: w2209 -> [_ w2305]
              tunnel: w2224 -> [_ w2304]
              tunnel: w2217 -> [_ w2303]
              tunnel: w2213 -> [_ w2302]
              tunnel: w2206 -> [_ w2301]
              tunnel: w2216 -> [_ w2300]
              tunnel: [w2291 w2299] -> w2208
              tunnel: [w2292 w2298] -> w2207
              tunnel: w2214 -> [_ w2293]
              frame False {
              }
              frame True {
                n1081 = Enqueue Element(queue=w2294, element=w2293, error in (no error)=w2297) -> (queue out=w2295:refnum<queue>, error out=w2296:errorcluster)  [unwired: 1 in, 1 out]
                n1082 = for {
                  N: w2310 -> [_]
                  shift-right: [w2331] -> w2307
                  shift-left: w2295 -> [w2337]
                  shift-right: [w2330] -> w2306
                  shift-left: w2296 -> [w2336]
                  tunnel: w2309 -> [w2335]
                  tunnel: w2305 -> [w2332]
                  n1083 = Enqueue Element(queue=w2337, element=w2335, error in (no error)=w2336) -> (queue out=w2333:refnum<queue>, error out=w2334:errorcluster)  [unwired: 1 in, 1 out]
                  n1084 = Enqueue Element(queue=w2333, element=w2332, error in (no error)=w2334) -> (queue out=w2331:refnum<queue>, error out=w2330:errorcluster)  [unwired: 1 in, 1 out]
                }
                n1085 = case shown="True" "Spin at end" {
                  tunnel: w2307 -> [w2312 w2329]
                  tunnel: w2306 -> [w2311 w2328]
                  tunnel: w2304 -> [_ w2323]
                  tunnel: w2303 -> [_ w2322]
                  tunnel: w2302 -> [_ w2321]
                  tunnel: w2301 -> [_ w2316]
                  tunnel: w2300 -> [_ w2315]
                  tunnel: [w2311 w2314] -> w2299
                  tunnel: [w2312 w2313] -> w2298
                  frame False {
                  }
                  frame True {
                    n1086 = Enqueue Element(queue=w2329, element=w2323, error in (no error)=w2328) -> (queue out=w2327:refnum<queue>, error out=w2326:errorcluster)  [unwired: 1 in, 1 out]
                    n1087 = Enqueue Element(queue=w2327, element=w2322, error in (no error)=w2326) -> (queue out=w2325:refnum<queue>, error out=w2324:errorcluster)  [unwired: 1 in, 1 out]
                    n1088 = Enqueue Element(queue=w2325, element=w2321, error in (no error)=w2324) -> (queue out=w2320:refnum<queue>, error out=w2319:errorcluster)  [unwired: 1 in, 1 out]
                    n1089 = Enqueue Element(queue=w2320, element=w2316, error in (no error)=w2319) -> (queue out=w2317:refnum<queue>, error out=w2318:errorcluster)  [unwired: 1 in, 1 out]
                    n1090 = Enqueue Element(queue=w2317, element=w2315, error in (no error)=w2318) -> (queue out=w2313:refnum<queue>, error out=w2314:errorcluster)  [unwired: 1 in, 1 out]
                  }
                }
              }
            }
            n1091 = Bundle By Name(cluster=w2206, "QueueAction"=DeviceQueue_Action."Arduino_Shutter_Close") -> (w2205:T11)
            n1092 = Enqueue Element(queue=w2207, element=w2205, error in (no error)=w2208) -> (queue out=w2203:refnum<queue>, error out=w2202:errorcluster)  [unwired: 1 in, 1 out]
            "Nr After Spin" <- u16 0 ("Nr After Spin")
          }
          frame "Measure_InSituAdvanced_Short" {
            w2391 = T11 {"QueueAction"=enum."TimeOut", "Numeric 1"=0.0, "Numeric 2"=0.0, "Boolean 1"=FALSE, "Boolean 2"=FALSE, "Spin Program"=[], "Spin Prg v07"=[], "Time Stamp"=timestamp(0 s since 1904-01-01), "TabControl"=enum."Measure"}  # Device Queue
            n1093 = property on="Nr After Spin" class="DigNum (strict)"("Value"=u16 0 ("Nr After Spin")) -> ()  [unwired: 2 in, 2 out]
            n1094 = Bundle By Name(cluster=w2391, "QueueAction"=DeviceQueue_Action."Spectrometer_SetTriggerMode", "Numeric 1"=1.0) -> (w2353:T11)
            n1095 = Bundle By Name(cluster=w2353, "QueueAction"=DeviceQueue_Action."Spectrometer_DeviceInformation") -> (w2383:T11)
            n1096 = property on="Frames" class="DigNum (strict)"() -> ("Value"=w2344:i32)  [unwired: 2 in, 2 out]
            n1097 = Bundle By Name(cluster=w2383, "QueueAction"=DeviceQueue_Action."Spectrometer_StartMeasurement") -> (w2381:T11)
            n1098 = Enqueue Element(queue=w2390, element=w2353, error in (no error)=w2354) -> (queue out=w2387:refnum<queue>, error out=w2388:errorcluster)  [unwired: 1 in, 1 out]
            n1099 = Bundle By Name(cluster=w2381, "QueueAction"=DeviceQueue_Action."Arduino_StartProgram", "Numeric 1"=2.0) -> (w2376:T11)
            n1100 = Enqueue Element(queue=w2387, element=w2383, error in (no error)=w2388) -> (queue out=w2385:refnum<queue>, error out=w2384:errorcluster)  [unwired: 1 in, 1 out]
            n1101 = Bundle By Name(cluster=w2376, "QueueAction"=DeviceQueue_Action."Spectrometer_GetData_Short", "Numeric 2"=w2344) -> (w2371:T11)
            n1102 = Enqueue Element(queue=w2385, element=w2381, error in (no error)=w2384) -> (queue out=w2380:refnum<queue>, error out=w2379:errorcluster)  [unwired: 1 in, 1 out]
            n1103 = Enqueue Element(queue=w2380, element=w2376, error in (no error)=w2379) -> (queue out=w2377:refnum<queue>, error out=w2374:errorcluster)  [unwired: 1 in, 1 out]
            n1104 = Bundle By Name(cluster=w2371, "QueueAction"=DeviceQueue_Action."Spectrometer_StopMeasurement") -> (w2367:T11)
            n1105 = property on="Measure_FramesSpectrometer" class="DigNum (strict)"() -> ("Value"=w2355:dbl)  [unwired: 2 in, 2 out]
            n1106 = Enqueue Element(queue=w2377, element=w2371, error in (no error)=w2374) -> (queue out=w2373:refnum<queue>, error out=w2372:errorcluster)  [unwired: 1 in, 1 out]
            n1107 = Bundle By Name(cluster=w2367, "QueueAction"=DeviceQueue_Action."Measure_Stop") -> (w2360:T11)
            n1108 = Bundle By Name(cluster=w2360, "QueueAction"=DeviceQueue_Action."Spectrometer_SetTriggerMode", "Numeric 1"=0.0) -> (w2357:T11)
            n1109 = Enqueue Element(queue=w2373, element=w2367, error in (no error)=w2372) -> (queue out=w2368:refnum<queue>, error out=w2369:errorcluster)  [unwired: 1 in, 1 out]
            n1110 = Bundle By Name(cluster=w2357, "QueueAction"=DeviceQueue_Action."Spectrometer_SetFrames", "Numeric 1"=w2355) -> (w2349:T11)
            n1111 = Enqueue Element(queue=w2368, element=w2360, error in (no error)=w2369) -> (queue out=w2363:refnum<queue>, error out=w2364:errorcluster)  [unwired: 1 in, 1 out]
            n1112 = Enqueue Element(queue=w2363, element=w2357, error in (no error)=w2364) -> (queue out=w2362:refnum<queue>, error out=w2361:errorcluster)  [unwired: 1 in, 1 out]
            n1113 = Enqueue Element(queue=w2362, element=w2349, error in (no error)=w2361) -> (queue out=w2348:refnum<queue>, error out=w2347:errorcluster)  [unwired: 1 in, 1 out]
            n1114 = Bundle By Name(cluster=w2349, "QueueAction"=DeviceQueue_Action."Arduino_Shutter_Close") -> (w2352:T11)
            n1115 = Enqueue Element(queue=w2348, element=w2352, error in (no error)=w2347) -> (queue out=w2350:refnum<queue>, error out=w2343:errorcluster)  [unwired: 1 in, 1 out]
          }
          frame "Measure_Spectrum" {
            n1116 = Unbundle By Name(w2394) -> ("Time Stamp"=w2395:timestamp)
            n1117 = Bundle By Name(cluster=w2394, "QueueAction"=DeviceQueue_Action."Spectrometer_Measure", "Time Stamp"=w2395) -> (w2400:T11)
            n1118 = Bundle By Name(cluster=w2400, "QueueAction"=DeviceQueue_Action."Measure_Stop") -> (w2398:T11)
            n1119 = Enqueue Element(queue=w2406, element=w2400, error in (no error)=w2405) -> (queue out=w2401:refnum<queue>, error out=w2402:errorcluster)  [unwired: 1 in, 1 out]
            n1120 = Enqueue Element(queue=w2401, element=w2398, error in (no error)=w2402) -> (queue out=w2397:refnum<queue>, error out=w2396:errorcluster)  [unwired: 1 in, 1 out]
          }
          frame "Measure_SpectralStability" {
            n1121 = Bundle By Name(cluster=w2410, "QueueAction"=DeviceQueue_Action."Spectrometer_DeviceInformation") -> (w2413:T11)
            n1122 = property on="SpectralStability_\nFrameRate" class="DigNum (strict)"() -> ("Value"=w2433:dbl[unit])  [unwired: 2 in, 2 out]
            n1123 = property on="SpectralStability_\nFramesSpectrometer" class="DigNum (strict)"() -> ("Value"=w2434:dbl)  [unwired: 2 in, 2 out]
            n1124 = Bundle By Name(cluster=w2413, "QueueAction"=DeviceQueue_Action."Spectrometer_Measure") -> (w2412:T11)
            n1125 = Enqueue Element(queue=w2416, element=w2413, error in (no error)=w2415) -> (queue out=w2418:refnum<queue>, error out=w2417:errorcluster)  [unwired: 1 in, 1 out]
            n1126 = Divide(x=w2434, y=w2433) -> (x/y=w2428:dbl[unit])
            n1127 = Unbundle By Name(w2410) -> ("Numeric 1"=w2409:dbl)
            n1128 = Subtract(x="SpectralStability_\nPeriodicTime", y=w2428) -> (x-y=w2427:dbl[unit])
            n1129 = Enqueue Element(queue=w2418, element=w2412, error in (no error)=w2417) -> (queue out=w2432:refnum<queue>, error out=w2431:errorcluster)  [unwired: 1 in, 1 out]
            n1130 = node(w2427) -> (w2426:dbl)
            n1131 = Decrement(x=w2409) -> (x-1=w2408:dbl)
            n1132 = Bundle By Name(cluster=w2412, "QueueAction"=DeviceQueue_Action."Wait", "Numeric 1"=w2426) -> (w2422:T11)
            n1133 = for {
              N: w2408 -> [_]
              shift-right: [w2438] -> w2425
              shift-left: w2432 -> [w2444]
              shift-right: [w2437] -> w2424
              shift-left: w2431 -> [w2443]
              tunnel: w2422 -> [w2440]
              tunnel: w2412 -> [w2439]
              n1134 = Enqueue Element(queue=w2444, element=w2440, error in (no error)=w2443) -> (queue out=w2442:refnum<queue>, error out=w2441:errorcluster)  [unwired: 1 in, 1 out]
              n1135 = Enqueue Element(queue=w2442, element=w2439, error in (no error)=w2441) -> (queue out=w2438:refnum<queue>, error out=w2437:errorcluster)  [unwired: 1 in, 1 out]
            }
            n1136 = Bundle By Name(cluster=w2422, "QueueAction"=DeviceQueue_Action."Measure_Stop") -> (w2421:T11)
            n1137 = Enqueue Element(queue=w2425, element=w2421, error in (no error)=w2424) -> (queue out=w2419:refnum<queue>, error out=w2420:errorcluster)  [unwired: 1 in, 1 out]
          }
        }
      }
      frame Error {
        w2449 = T19 4 items=["no dialog", "OK message", "continue or stop message", "OK message + warnings", "continue/stop + warnings"] ("type of dialog (OK msg:1)")
        n1138 = call <vilib>:"General Error Handler.vi"("type of dialog (OK msg:1)"=w2449, "error in (no error)"=w2450) -> ("error out"=w2448:errorcluster)  [unwired: 9 in, 4 out]
        n1139 = call <vilib>:"Clear Errors.vi"("error in (no error)"=w2448) -> ("error out"=w2447:errorcluster)  [unwired: 5 in, 1 out]
      }
    }
  }
  n1140 = disable-structure shown="Disabled" {
    frame Disabled {
      w2453 = T11 {"QueueAction"=enum."TimeOut", "Numeric 1"=0.0, "Numeric 2"=0.0, "Boolean 1"=FALSE, "Boolean 2"=FALSE, "Spin Program"=[], "Spin Prg v07"=[], "Time Stamp"=timestamp(0 s since 1904-01-01), "TabControl"=enum."Measure"}  # Device Queue
      n1141 = Bundle By Name(cluster=w2453, "QueueAction"=DeviceQueue_Action."Arduino_SetSpeed") -> (w2454:T11)  [unwired: 1 in]
      n1142 = Enqueue Element(element=w2454) -> ()  [unwired: 3 in, 3 out]
    }
    frame Enabled {
    }
  }
  n1143 = Release Queue(queue=w9) -> ()  [unwired: 2 in, 3 out]
  n1144 = Release Queue(queue=w10) -> ()  [unwired: 2 in, 3 out]
